vi "BeamPointing General hacking.vi"() -> ()   [LabVIEW 2013]
doc: "This example illustrates how to perform a continuous acquisition with a USB camera."
uses:
  <vilib>/vision/Image Controls.llb/IMAQ Image.ctl
  <vilib>/userdefined/High Color/IMAQdx.ctl
  shared programs/GUI_Template/GUI_master/tcp_new_data_event.ctl
  shared programs/GUI_Template/GUI_master/tcp new data cluster.ctl
  Add ROI Offset ImgData.vi
  Add Or Replace Coord Array.vi
  Add Or Replace Img Array.vi
  Add ROI Offset RectFilter.vi
  Add Or Replace String Array.vi
  <vilib>/regexp/Match Regular Expression.xnode
  <vilib>/vision/NI_Vision_Development_Module.lvlib
  <resource>/objmgr/IMAQImage.rc
  <vilib>/Analysis/NI_AALBase.lvlib
  <vilib>/Analysis/NI_AALPro.lvlib
panel:
  out "Main processing loop i":i32=3683
  out "image::1":T1(plugin-control) caption="Mode1"
  out "image::4":T1(plugin-control) caption="Mode1"
  out "image::5":T1(plugin-control) caption="Mode1"
  out "image::6":T1(plugin-control) caption="Mode1"
  out "image::7":T1(plugin-control) caption="Mode1"
  out "image::8":T1(plugin-control) caption="Mode1"
  out "GUIdevice 5":string="M1Cam"
  out "GUIdevice 4":string="M1Cam"
  out "GUIdevice 7":string="M1Cam"
  out "GUIdevice 6":string="M1Cam"
  out "GUIdevice 8":string="M1Cam"
  out "GUIdevice 9":string="M1Cam"
  out "image::9":T1(plugin-control) caption="Mode1"
  out "GUIdevice 3":string="M1Cam"
  out "GUIdevice 1":string="M1Cam"
  out "GUIdevice 2":string="M1Cam"
  out "image::2":T1(plugin-control) caption="Mode1"
  out "image::3":T1(plugin-control) caption="Mode1"
  out "error IO 2":errorcluster
  in  "insert tag":bool=TRUE
  out "tcp data event":T2
  out "configarraychanged":bool
  out "image names":string[](array[string])
  in  "recenter":bool
  out "Beam Detected":bool
  out "Move Y":bool
  out "Move X":bool
  in  "LoopMode":bool caption="Mode"
  in  "rescale":bool=TRUE
  in  "Step Size":u16=5
  in  "Feedback":bool
  out "MoveInProgress":bool caption="Move In Progress"
  in  "USB cameras":i32(listbox)=1 caption="Select Camera"
  in  "Manual Move":T3={"Down"=FALSE, "Up"=FALSE, "Right"=FALSE, "Left"=FALSE, "APulses X"=200, "APulses Y"=200, "StopButton"=FALSE}
  out "Status":string
  in  "Internal controls and indicators":T4(tab)
  out "grab loop i":i32=4
  out "Current ImageServer":cluster{"IPAddress":string, "Port":i32}={"IPAddress"="234.5.6.8", "Port"=58445}
  out "Ann. Images":T1[](array[typedef])=["imageserver0", "imageserver1", "imageserver2", "imageserver3", "imageserver4", "imageserver5"]
  in  "Tab Control 2":enum32{"Image saving", "stats", "TCP", "cams"}(tab)=enum."cams"
  in  "Boolean":bool
  in  "Base Directory":path
  out "SaveImgError":errorcluster
  in  "SavePict":bool
  out "error CamS":errorcluster
  out "Switch Time":u32=200
  out "one loop":u32=130
  out "# imgs in buffer":i32=5
  out "ImgBufferSize":i32=5
  out "AcqTime":u32=610845
  out "State":i32=12
  out "TCPconnecAnswer":bool=TRUE
  out "TCPconnecCmd":bool=TRUE
  out "error close connect":errorcluster
  in  "Remove Camera":bool
  in  "Mirror List Path":path=path "Z:/Software/control-common/Configuration files/DeviceList100TW.xml"
  out "XML Config File Path":path=path "Z:/Software/control-common/Configuration files/ConfigFile_192_168_10_184.xml"
  in  "Add Camera":bool
  out "# of cams":i32=6
  in  "Corr":bool[](array[boolean])=[FALSE, FALSE, FALSE, FALSE, FALSE, FALSE]
  out "Det":bool[](array[boolean])
  out "error out":errorcluster
  out "IMAQ status":bool
  out "Avg Img Buffer":u8[][][](array[numeric])
  out "Switch in":u32=299180745
  out "MirrorList":string[][](array[string])
  out "Corrective Move XY":T5(array[cluster])
  out "Cameras Names":string[](array[string])=["Null", "Null", "Null", "Null", "Null", "Null"]
  out "Deviation":cluster{"Dev. X":sgl, "Dev. Y":sgl}={"Dev. X"=0.0, "Dev. Y"=-5.0} {"Dev. X" format="%.1f"; "Dev. Y" format="%.1f"}
  out "Buffer2":T1
  out "DownloadedImg":T1
  out "CurrentName":string="*100TW M10"
  out "XML errors":bool
  out "Image Odd Out":T1
  out "DeviceNames":string[](array[string])=["no-device", "GasJet", "Godzilla_M1", "Godzilla_M2", "Godzilla_M3", "Godzilla_M4", "Godzilla_M6", "Godzilla_M8_Steer", "Chihuahua_M1", "Chihuahua_M2", "Collider_M4", "Collider_M5", "Collider_M8 Translation s3c4", "HeaterBlue-M1", "HeaterBlue-M2", "HeaterBlue-M3", "THz OAP Down", "G Spot Camera", "G Spot Monitor", "C Spot Monitor", "p15c4-Free", "THz_M5", "THz_M7A & Xtal", "THz_M7B", "THz MIrror Top", "THz OAP Top", "p2s2c2-Free", "p2s2c3-Free", "p2s2c4-Free", "Heater_M0", "Heater_M4", "Heater_M5", "Ignitor Iris", "Ignitor_M4", "Collider_M6", "Collder_M7", "C Spot Camera", "p2s5c1-FREE", "p2s5c2-FREE", "p2s5c3-FREE", "p2c5c4-FREE", "*100TW M9", "*100TW M10", "*100TW Preamp Up", "*100TW Input Preamp2", "*100TW Output Preamp2", "*100TW M0", "*100TW M2", "*100TW M4", "*100TW M6", "*100TW M8", "*100TW M13", "*100TW M20", "*100TW M22", "*100TW M23", "no pico", "no pico", "no pico", "mobile no ir", "regen out-salad#1", "preamp in-salad#2", "XPW 1", "blue periscope regen", "godzilla 1st", "godzilla IN", "Chihuahua IN", "Chihuahua 1st", "??XPW pico2", "Preamp 3rd pass", "Blue regen out"]
  out "size(s)":i32[](array[numeric])=[964, 1288]
  out "Iteration":u32
  in  "Onward":bool=TRUE
  out "Ellipse edges":cluster{"X":sgl, "Y":sgl}[](array[cluster])
  out "Buffer":T1
  out "Output Img":T1
  out "Reference Img":T1
  out "Background Img":T1
  out "counter":i32
  out "First step":bool
  out "IMAQ Session":refnum<k11>
  out "IMAQ Session Array":refnum<k11>[](array[refnum])
  out "Display Current":bool=TRUE
  out "Region of Interest":i32[](array[numeric])
  out "Acq Img":T1
  out "MoveInProgressTimeIN":u32=296721656
  out "IMAQdx Session":T6="cam2"
  out "start":u32=299180614
  out "Avg Deviation":cluster{sgl, sgl}={0.0, -5.0}
  out "InProgress":string[](array[string])
  out "Centroid Avg Buffer":cluster{"X Centroid":sgl, "Y Centroid":sgl}[](array[cluster])=[{"X Centroid"=343.0, "Y Centroid"=203.0}, {"X Centroid"=301.0, "Y Centroid"=181.0}, {"X Centroid"=334.0, "Y Centroid"=201.0}, {"X Centroid"=289.0, "Y Centroid"=154.0}, {"X Centroid"=319.0, "Y Centroid"=232.0}]
  out "Img Buffer":T1[](array[typedef])=["Buffer0", "Buffer1", "Buffer2", "Buffer3", "Buffer4"]
  out "OpenTime":u32=298569900
  out "RunON/OFF":bool
  out "last move time":u32=281970384
  out "DeviationArray":cluster{"X Centroid":sgl, "Y Centroid":sgl}[](array[cluster])
  out "ConnectArray":T7(array[cluster])=[{"IPaddress"="192.168.10.34", "Port"=63420, "connection ID"=refnum, "TCP error"={"status"=FALSE, "code"=0, "source"=""}}, {"IPaddress"="192.168.10.184", "Port"=63430, "connection ID"=refnum, "TCP error"={"status"=FALSE, "code"=0, "source"=""}}]
  out "Raw images":T1[](array[typedef])=["imageserver0", "imageserver1", "imageserver2", "imageserver3", "imageserver4", "imageserver5"]
  in  "XML Config File Path 2":path=path "H:/Software/control-common/Configuration files/ConfigFile_192_168_10_184.xml"
  out "AddCameraCluster":T8={"Add?"=FALSE, "Channel"=6, "Device Name"="no-device"}
  out "RemoveCameraCluster":cluster{"Remove?":bool, "number":i32}={"Remove?"=FALSE, "number"=-1}
  out "NewAvg":bool
  out "Thresh Img":T1
  out "Avg Img":T1
  out "really save cfg?":bool
  out "Buffer3":T1
  out "CamConfigArray":T9(array[cluster])=[{"ID"=64.0, "Name"="*100TW M8", "DeviceID"={"Slot Connector"=24, "IP Adress"="192.168.10.34", "Port"=63420, "Type"="picodriver"}, "CorrectConfig Cluster"={"Detection Parameters"={"Contrast"=0, "Treshold"=0, "Max Intensity"=0, "Max Intensity%"=0, "Rx"=0, "Ry"=0, "R%"=0.0}, "Reverse"={"Reverse X"=FALSE, "Reverse Y"=FALSE}, "Target"={"X Target"=0.0, "Y Target"=0.0}, "Region of Interest"=[0, 0, 0, 0], "Correction Parameters"={"X"=0.0, "Y"=0.0, "Movement Type"=0}, "Acquisition Parameters"={"Brightness"=0.0, "Contrast"=0.0, "Saturation"=0.0, "White level"=0.0}, "Background Path"=path "", "Reference Path"=path "", "XCalibration"=[], "YCalibration"=[]}, "Ontrak Channel"=0, "IMAQdx Session 2"="cam2", "ImageServer"={"IPAddress"="234.5.6.8", "Port"=58450}}, {"ID"=55.0, "Name"="*100TW M9", "DeviceID"={"Slot Connector"=31, "IP Adress"="192.168.10.34", "Port"=63420, "Type"="picodriver"}, "CorrectConfig Cluster"={"Detection Parameters"={"Contrast"=0, "Treshold"=0, "Max Intensity"=0, "Max Intensity%"=0, "Rx"=0, "Ry"=0, "R%"=0.0}, "Reverse"={"Reverse X"=FALSE, "Reverse Y"=FALSE}, "Target"={"X Target"=631.0, "Y Target"=473.0}, "Region of Interest"=[0, 0, 0, 0], "Correction Parameters"={"X"=0.0, "Y"=0.0, "Movement Type"=0}, "Acquisition Parameters"={"Brightness"=0.0, "Contrast"=0.0, "Saturation"=0.0, "White level"=0.0}, "Background Path"=path "", "Reference Path"=path "", "XCalibration"=[], "YCalibration"=[]}, "Ontrak Channel"=0, "IMAQdx Session 2"="cam2", "ImageServer"={"IPAddress"="234.5.6.8", "Port"=58444}}, {"ID"=56.0, "Name"="*100TW M10", "DeviceID"={"Slot Connector"=32, "IP Adress"="192.168.10.34", "Port"=63420, "Type"="picodriver"}, "CorrectConfig Cluster"={"Detection Parameters"={"Contrast"=53, "Treshold"=53, "Max Intensity"=255, "Max Intensity%"=80, "Rx"=116, "Ry"=92, "R%"=50.0}, "Reverse"={"Reverse X"=FALSE, "Reverse Y"=TRUE}, "Target"={"X Target"=334.0, "Y Target"=206.0}, "Region of Interest"=[0, 0, 0, 0], "Correction Parameters"={"X"=100.0, "Y"=100.0, "Movement Type"=0}, "Acquisition Parameters"={"Brightness"=0.0, "Contrast"=0.0, "Saturation"=0.0, "White level"=0.0}, "Background Path"=path "", "Reference Path"=path "", "XCalibration"=[], "YCalibration"=[]}, "Ontrak Channel"=0, "IMAQdx Session 2"="cam2", "ImageServer"={"IPAddress"="234.5.6.8", "Port"=58445}}, {"ID"=0.0, "Name"="*100TW M20", "DeviceID"={"Slot Connector"=1, "IP Adress"="192.168.10.184", "Port"=63430, "Type"="picodriver"}, "CorrectConfig Cluster"={"Detection Parameters"={"Contrast"=66, "Treshold"=66, "Max Intensity"=255, "Max Intensity%"=80, "Rx"=30, "Ry"=30, "R%"=50.0}, "Reverse"={"Reverse X"=TRUE, "Reverse Y"=TRUE}, "Target"={"X Target"=284.6373, "Y Target"=160.1435}, "Region of Interest"=[0, 0, 0, 0], "Correction Parameters"={"X"=20.0, "Y"=20.0, "Movement Type"=0}, "Acquisition Parameters"={"Brightness"=0.0, "Contrast"=0.0, "Saturation"=0.0, "White level"=0.0}, "Background Path"=path "", "Reference Path"=path "", "XCalibration"=[{-23000.0, -242.0}, {-22000.0, -229.0}, {-21000.0, -215.0}, {-20000.0, -203.0}, {-19000.0, -192.0}, {-18000.0, -182.0}, {-17000.0, -172.0}, {-16000.0, -162.0}, {-15000.0, -153.0}, {-14000.0, -141.0}, {-13000.0, -126.0}, {-12000.0, -105.0}, {-11000.0, -77.0}, {-10000.0, -44.0}, {0.0, 4.0}, {11000.0, 98.0}, {12000.0, 109.0}, {13000.0, 119.0}, {14000.0, 130.0}, {15000.0, 140.0}, {16000.0, 151.0}, {17000.0, 161.0}, {18000.0, 171.0}, {19000.0, 182.0}, {20000.0, 193.0}, {21000.0, 205.0}, {22000.0, 217.0}, {23000.0, 229.0}], "YCalibration"=[{-23000.0, 196.0}, {-22000.0, 189.0}, {-21000.0, 182.0}, {-20000.0, 174.0}, {-19000.0, 164.0}, {-18000.0, 153.0}, {-17000.0, 141.0}, {-16000.0, 133.0}, {-15000.0, 126.0}, {-14000.0, 117.0}, {-13000.0, 105.0}, {-12000.0, 90.0}, {-11000.0, 69.0}, {-10000.0, 42.0}, {0.0, -4.0}, {11000.0, -96.0}, {12000.0, -99.0}, {13000.0, -101.0}, {14000.0, -103.0}, {15000.0, -109.0}, {16000.0, -118.0}, {17000.0, -129.0}, {18000.0, -143.0}, {19000.0, -155.0}, {20000.0, -166.0}, {21000.0, -174.0}, {22000.0, -181.0}, {23000.0, -187.0}]}, "Ontrak Channel"=0, "IMAQdx Session 2"="cam2", "ImageServer"={"IPAddress"="234.5.6.8", "Port"=58443}}, {"ID"=12.0, "Name"="*100TW M22", "DeviceID"={"Slot Connector"=3, "IP Adress"="192.168.10.184", "Port"=63430, "Type"="picodriver"}, "CorrectConfig Cluster"={"Detection Parameters"={"Contrast"=59, "Treshold"=59, "Max Intensity"=255, "Max Intensity%"=80, "Rx"=47, "Ry"=33, "R%"=50.0}, "Reverse"={"Reverse X"=FALSE, "Reverse Y"=TRUE}, "Target"={"X Target"=319.0, "Y Target"=219.0}, "Region of Interest"=[0, 0, 0, 0], "Correction Parameters"={"X"=10000.0, "Y"=10000.0, "Movement Type"=0}, "Acquisition Parameters"={"Brightness"=0.0, "Contrast"=0.0, "Saturation"=0.0, "White level"=0.0}, "Background Path"=path "", "Reference Path"=path "", "XCalibration"=[], "YCalibration"=[]}, "Ontrak Channel"=0, "IMAQdx Session 2"="cam2", "ImageServer"={"IPAddress"="234.5.6.8", "Port"=58446}}, {"ID"=12.0, "Name"="*100TW M23", "DeviceID"={"Slot Connector"=4, "IP Adress"="192.168.10.184", "Port"=63430, "Type"="picodriver"}, "CorrectConfig Cluster"={"Detection Parameters"={"Contrast"=11, "Treshold"=11, "Max Intensity"=255, "Max Intensity%"=90, "Rx"=180, "Ry"=110, "R%"=50.0}, "Reverse"={"Reverse X"=FALSE, "Reverse Y"=TRUE}, "Target"={"X Target"=303.0, "Y Target"=342.0}, "Region of Interest"=[0, 0, 0, 0], "Correction Parameters"={"X"=0.0, "Y"=0.0, "Movement Type"=0}, "Acquisition Parameters"={"Brightness"=0.0, "Contrast"=0.0, "Saturation"=0.0, "White level"=0.0}, "Background Path"=path "", "Reference Path"=path "", "XCalibration"=[], "YCalibration"=[]}, "Ontrak Channel"=0, "IMAQdx Session 2"="cam2", "ImageServer"={"IPAddress"="234.5.6.8", "Port"=58442}}] {"CorrectConfig Cluster"."Acquisition Parameters"."White level" scale=0.3..1.26 scale format="%#_2f"; "CorrectConfig Cluster"."Acquisition Parameters"."Saturation" scale=0.5..1.5 scale format="%#_3f"; "CorrectConfig Cluster"."Acquisition Parameters"."Contrast" scale=0.4..1.5 scale format="%#_3f"; "CorrectConfig Cluster"."Acquisition Parameters"."Brightness" scale=-50.0..50.0 scale format="%#_2f"; "CorrectConfig Cluster"."Correction Parameters"."Movement Type" items=["Step", "Proportionnal"]; "CorrectConfig Cluster"."Target"."X Target" format="%#_5g"; "CorrectConfig Cluster"."Target"."Y Target" format="%#_5g"; "CorrectConfig Cluster"."Detection Parameters"."Max Intensity%" max=100 step=1}
  out "Ellipse":T10 {"Minor Axis"."Point 2"."Y" format="%.2f"; "Minor Axis"."Point 2"."X" format="%.2f"; "Minor Axis"."Point 1"."Y" format="%.2f"; "Minor Axis"."Point 1"."X" format="%.2f"; "Major Axis"."Point 2"."Y" format="%.2f"; "Major Axis"."Point 2"."X" format="%.2f"; "Major Axis"."Point 1"."Y" format="%.2f"; "Major Axis"."Point 1"."X" format="%.2f"; "Center"."Y" format="%.2f"; "Center"."X" format="%.2f"}
  out "Avg Variation":cluster{"mean X":dbl, "mean Y":dbl}={"mean X"=nan, "mean Y"=nan} {"mean X" format="%#_4g"; "mean Y" format="%#_4g"}
  in  "Acquisition Parameters dx":T11 {"Parameter4" min=0.0 max=0.1 scale=0.0..0.1 scale format="%#_2f"; "Parameter3" min=0.0 max=3.0 scale=0.0..3.0 scale format="%#_3f"; "Parameter2" min=1.0 max=10.0 scale=1.0..10.0 scale format="%#_3f"; "Parameter1" min=1 max=1048576 step=1 scale=1.0..1048576.0}
  in  "set scales":bool
  out "Image Ports":i32[](array[numeric])
  out "Image IPs":string[](array[string])
  out "device associated":string
  in  "Background Path":path
  in  "Reference Path":path
  out "BestRects Cluster":T12={"PreviousCenter"={"X"=0.0, "Y"=0.0}, "CurrentCenter"={"X"=334.0, "Y"=201.0}}
  out "Default devices":string[](array[string])=["*100TW M8", "*100TW M9", "*100TW M10", "*100TW M20", "*100TW M22", "*100TW M23"]
  out "Img Size":i32[](array[numeric])=[0, 0, 1288, 964]
  out "RectFilter":T13={"Left"=257, "Top"=144, "Right"=399, "Bottom"=260, "Rotation"=10.484647750854492} {"Rotation" format="%.2f"; "Left" scale=0.0..1024.0; "Right" scale=0.0..1024.0}
  out "History XY Buffer":T14(array[cluster])
  out "ImgDataArray":T15(array[cluster])
  out "DeviceList":T16(array[cluster])=[{"ID"=0.0, "Name"="no-device", "DeviceID"={"Slot Connector"=0, "IP Adress"="Ipaddress", "Port"=0, "Type"="Type"}, "Detection Parameters"={"Contrast"=0, "Treshold"=0, "Max Intensity"=0, "Max Intensity%"=0, "Rx"=0, "Ry"=0, "R%"=0.0}, "Reverse"={"Reverse X"=FALSE, "Reverse Y"=FALSE}, "Target"={"X Target"=0.0, "Y Target"=0.0}, "Region of Interest"=[0, 0, 0, 0], "Correction Parameters"={"X"=0.0, "Y"=0.0, "Movement Type"=0}, "Acquisition Parameters"={"Brightness"=0.0, "Contrast"=0.0, "Saturation"=0.0, "White level"=0.0}, "Background Path"=path "", "Reference Path"=path "", "XCalibration"=[], "YCalibration"=[], "ImageServer"={"IPAddress"="127.0.0.1", "Port"=3500}}, {"ID"=0.0, "Name"="GasJet", "DeviceID"={"Slot Connector"=44, "IP Adress"="192.168.10.183", "Port"=63400, "Type"="picodriver"}, "Detection Parameters"={"Contrast"=0, "Treshold"=0, "Max Intensity"=0, "Max Intensity%"=0, "Rx"=0, "Ry"=0, "R%"=0.0}, "Reverse"={"Reverse X"=FALSE, "Reverse Y"=FALSE}, "Target"={"X Target"=0.0, "Y Target"=0.0}, "Region of Interest"=[0, 0, 0, 0], "Correction Parameters"={"X"=0.0, "Y"=0.0, "Movement Type"=0}, "Acquisition Parameters"={"Brightness"=0.0, "Contrast"=0.0, "Saturation"=0.0, "White level"=0.0}, "Background Path"=path "", "Reference Path"=path "", "XCalibration"=[], "YCalibration"=[], "ImageServer"={"IPAddress"="127.0.0.1", "Port"=3500}}, {"ID"=14.0, "Name"="Godzilla_M1", "DeviceID"={"Slot Connector"=11, "IP Adress"="192.168.10.183", "Port"=63400, "Type"="picodriver"}, "Detection Parameters"={"Contrast"=0, "Treshold"=0, "Max Intensity"=0, "Max Intensity%"=0, "Rx"=0, "Ry"=0, "R%"=0.0}, "Reverse"={"Reverse X"=FALSE, "Reverse Y"=FALSE}, "Target"={"X Target"=0.0, "Y Target"=0.0}, "Region of Interest"=[0, 0, 0, 0], "Correction Parameters"={"X"=0.0, "Y"=0.0, "Movement Type"=0}, "Acquisition Parameters"={"Brightness"=0.0, "Contrast"=0.0, "Saturation"=0.0, "White level"=0.0}, "Background Path"=path "", "Reference Path"=path "", "XCalibration"=[], "YCalibration"=[], "ImageServer"={"IPAddress"="127.0.0.1", "Port"=3500}}, {"ID"=15.0, "Name"="Godzilla_M2", "DeviceID"={"Slot Connector"=12, "IP Adress"="192.168.10.183", "Port"=63400, "Type"="picodriver"}, "Detection Parameters"={"Contrast"=0, "Treshold"=0, "Max Intensity"=0, "Max Intensity%"=0, "Rx"=0, "Ry"=0, "R%"=0.0}, "Reverse"={"Reverse X"=FALSE, "Reverse Y"=FALSE}, "Target"={"X Target"=0.0, "Y Target"=0.0}, "Region of Interest"=[0, 0, 0, 0], "Correction Parameters"={"X"=0.0, "Y"=0.0, "Movement Type"=0}, "Acquisition Parameters"={"Brightness"=0.0, "Contrast"=0.0, "Saturation"=0.0, "White level"=0.0}, "Background Path"=path "", "Reference Path"=path "", "XCalibration"=[], "YCalibration"=[], "ImageServer"={"IPAddress"="127.0.0.1", "Port"=3500}}, {"ID"=16.0, "Name"="Godzilla_M3", "DeviceID"={"Slot Connector"=13, "IP Adress"="192.168.10.183", "Port"=63400, "Type"="picodriver"}, "Detection Parameters"={"Contrast"=0, "Treshold"=0, "Max Intensity"=0, "Max Intensity%"=0, "Rx"=0, "Ry"=0, "R%"=0.0}, "Reverse"={"Reverse X"=FALSE, "Reverse Y"=FALSE}, "Target"={"X Target"=0.0, "Y Target"=0.0}, "Region of Interest"=[0, 0, 0, 0], "Correction Parameters"={"X"=0.0, "Y"=0.0, "Movement Type"=0}, "Acquisition Parameters"={"Brightness"=0.0, "Contrast"=0.0, "Saturation"=0.0, "White level"=0.0}, "Background Path"=path "", "Reference Path"=path "", "XCalibration"=[], "YCalibration"=[], "ImageServer"={"IPAddress"="127.0.0.1", "Port"=3500}}, {"ID"=17.0, "Name"="Godzilla_M4", "DeviceID"={"Slot Connector"=14, "IP Adress"="192.168.10.183", "Port"=63400, "Type"="picodriver"}, "Detection Parameters"={"Contrast"=0, "Treshold"=0, "Max Intensity"=0, "Max Intensity%"=0, "Rx"=0, "Ry"=0, "R%"=0.0}, "Reverse"={"Reverse X"=FALSE, "Reverse Y"=FALSE}, "Target"={"X Target"=0.0, "Y Target"=0.0}, "Region of Interest"=[0, 0, 0, 0], "Correction Parameters"={"X"=0.0, "Y"=0.0, "Movement Type"=0}, "Acquisition Parameters"={"Brightness"=0.0, "Contrast"=0.0, "Saturation"=0.0, "White level"=0.0}, "Background Path"=path "", "Reference Path"=path "", "XCalibration"=[], "YCalibration"=[], "ImageServer"={"IPAddress"="127.0.0.1", "Port"=3500}}, {"ID"=18.0, "Name"="Godzilla_M6", "DeviceID"={"Slot Connector"=21, "IP Adress"="192.168.10.183", "Port"=63400, "Type"="picodriver"}, "Detection Parameters"={"Contrast"=0, "Treshold"=0, "Max Intensity"=0, "Max Intensity%"=0, "Rx"=0, "Ry"=0, "R%"=0.0}, "Reverse"={"Reverse X"=FALSE, "Reverse Y"=FALSE}, "Target"={"X Target"=0.0, "Y Target"=0.0}, "Region of Interest"=[0, 0, 0, 0], "Correction Parameters"={"X"=0.0, "Y"=0.0, "Movement Type"=0}, "Acquisition Parameters"={"Brightness"=0.0, "Contrast"=0.0, "Saturation"=0.0, "White level"=0.0}, "Background Path"=path "", "Reference Path"=path "", "XCalibration"=[], "YCalibration"=[], "ImageServer"={"IPAddress"="127.0.0.1", "Port"=3500}}, {"ID"=19.0, "Name"="Godzilla_M8_Steer", "DeviceID"={"Slot Connector"=22, "IP Adress"="192.168.10.183", "Port"=63400, "Type"="picodriver"}, "Detection Parameters"={"Contrast"=0, "Treshold"=0, "Max Intensity"=0, "Max Intensity%"=0, "Rx"=0, "Ry"=0, "R%"=0.0}, "Reverse"={"Reverse X"=FALSE, "Reverse Y"=FALSE}, "Target"={"X Target"=0.0, "Y Target"=0.0}, "Region of Interest"=[0, 0, 0, 0], "Correction Parameters"={"X"=0.0, "Y"=0.0, "Movement Type"=0}, "Acquisition Parameters"={"Brightness"=0.0, "Contrast"=0.0, "Saturation"=0.0, "White level"=0.0}, "Background Path"=path "", "Reference Path"=path "", "XCalibration"=[], "YCalibration"=[], "ImageServer"={"IPAddress"="127.0.0.1", "Port"=3500}}, {"ID"=20.0, "Name"="Chihuahua_M1", "DeviceID"={"Slot Connector"=23, "IP Adress"="192.168.10.183", "Port"=63400, "Type"="picodriver"}, "Detection Parameters"={"Contrast"=0, "Treshold"=0, "Max Intensity"=0, "Max Intensity%"=0, "Rx"=0, "Ry"=0, "R%"=0.0}, "Reverse"={"Reverse X"=FALSE, "Reverse Y"=FALSE}, "Target"={"X Target"=0.0, "Y Target"=0.0}, "Region of Interest"=[0, 0, 0, 0], "Correction Parameters"={"X"=0.0, "Y"=0.0, "Movement Type"=0}, "Acquisition Parameters"={"Brightness"=0.0, "Contrast"=0.0, "Saturation"=0.0, "White level"=0.0}, "Background Path"=path "", "Reference Path"=path "", "XCalibration"=[], "YCalibration"=[], "ImageServer"={"IPAddress"="127.0.0.1", "Port"=3500}}, {"ID"=21.0, "Name"="Chihuahua_M2", "DeviceID"={"Slot Connector"=24, "IP Adress"="192.168.10.183", "Port"=63400, "Type"="picodriver"}, "Detection Parameters"={"Contrast"=0, "Treshold"=0, "Max Intensity"=0, "Max Intensity%"=0, "Rx"=0, "Ry"=0, "R%"=0.0}, "Reverse"={"Reverse X"=FALSE, "Reverse Y"=FALSE}, "Target"={"X Target"=0.0, "Y Target"=0.0}, "Region of Interest"=[0, 0, 0, 0], "Correction Parameters"={"X"=0.0, "Y"=0.0, "Movement Type"=0}, "Acquisition Parameters"={"Brightness"=0.0, "Contrast"=0.0, "Saturation"=0.0, "White level"=0.0}, "Background Path"=path "", "Reference Path"=path "", "XCalibration"=[], "YCalibration"=[], "ImageServer"={"IPAddress"="127.0.0.1", "Port"=3500}}, {"ID"=22.0, "Name"="Collider_M4", "DeviceID"={"Slot Connector"=31, "IP Adress"="192.168.10.183", "Port"=63400, "Type"="picodriver"}, "Detection Parameters"={"Contrast"=0, "Treshold"=0, "Max Intensity"=0, "Max Intensity%"=0, "Rx"=0, "Ry"=0, "R%"=0.0}, "Reverse"={"Reverse X"=FALSE, "Reverse Y"=FALSE}, "Target"={"X Target"=0.0, "Y Target"=0.0}, "Region of Interest"=[0, 0, 0, 0], "Correction Parameters"={"X"=0.0, "Y"=0.0, "Movement Type"=0}, "Acquisition Parameters"={"Brightness"=0.0, "Contrast"=0.0, "Saturation"=0.0, "White level"=0.0}, "Background Path"=path "", "Reference Path"=path "", "XCalibration"=[], "YCalibration"=[], "ImageServer"={"IPAddress"="127.0.0.1", "Port"=3500}}, {"ID"=23.0, "Name"="Collider_M5", "DeviceID"={"Slot Connector"=32, "IP Adress"="192.168.10.183", "Port"=63400, "Type"="picodriver"}, "Detection Parameters"={"Contrast"=0, "Treshold"=0, "Max Intensity"=0, "Max Intensity%"=0, "Rx"=0, "Ry"=0, "R%"=0.0}, "Reverse"={"Reverse X"=FALSE, "Reverse Y"=FALSE}, "Target"={"X Target"=0.0, "Y Target"=0.0}, "Region of Interest"=[0, 0, 0, 0], "Correction Parameters"={"X"=0.0, "Y"=0.0, "Movement Type"=0}, "Acquisition Parameters"={"Brightness"=0.0, "Contrast"=0.0, "Saturation"=0.0, "White level"=0.0}, "Background Path"=path "", "Reference Path"=path "", "XCalibration"=[], "YCalibration"=[], "ImageServer"={"IPAddress"="127.0.0.1", "Port"=3500}}, {"ID"=24.0, "Name"="Collider_M8 Translation s3c4", "DeviceID"={"Slot Connector"=33, "IP Adress"="192.168.10.183", "Port"=63400, "Type"="picodriver"}, "Detection Parameters"={"Contrast"=0, "Treshold"=0, "Max Intensity"=0, "Max Intensity%"=0, "Rx"=0, "Ry"=0, "R%"=0.0}, "Reverse"={"Reverse X"=FALSE, "Reverse Y"=FALSE}, "Target"={"X Target"=0.0, "Y Target"=0.0}, "Region of Interest"=[0, 0, 0, 0], "Correction Parameters"={"X"=0.0, "Y"=0.0, "Movement Type"=0}, "Acquisition Parameters"={"Brightness"=0.0, "Contrast"=0.0, "Saturation"=0.0, "White level"=0.0}, "Background Path"=path "", "Reference Path"=path "", "XCalibration"=[], "YCalibration"=[], "ImageServer"={"IPAddress"="127.0.0.1", "Port"=3500}}, {"ID"=26.0, "Name"="HeaterBlue-M1", "DeviceID"={"Slot Connector"=34, "IP Adress"="192.168.10.183", "Port"=63400, "Type"="picodriver"}, "Detection Parameters"={"Contrast"=0, "Treshold"=0, "Max Intensity"=0, "Max Intensity%"=0, "Rx"=0, "Ry"=0, "R%"=0.0}, "Reverse"={"Reverse X"=FALSE, "Reverse Y"=FALSE}, "Target"={"X Target"=0.0, "Y Target"=0.0}, "Region of Interest"=[0, 0, 0, 0], "Correction Parameters"={"X"=0.0, "Y"=0.0, "Movement Type"=0}, "Acquisition Parameters"={"Brightness"=0.0, "Contrast"=0.0, "Saturation"=0.0, "White level"=0.0}, "Background Path"=path "", "Reference Path"=path "", "XCalibration"=[], "YCalibration"=[], "ImageServer"={"IPAddress"="127.0.0.1", "Port"=3500}}, {"ID"=27.0, "Name"="HeaterBlue-M2", "DeviceID"={"Slot Connector"=41, "IP Adress"="192.168.10.183", "Port"=63400, "Type"="picodriver"}, "Detection Parameters"={"Contrast"=0, "Treshold"=0, "Max Intensity"=0, "Max Intensity%"=0, "Rx"=0, "Ry"=0, "R%"=0.0}, "Reverse"={"Reverse X"=FALSE, "Reverse Y"=FALSE}, "Target"={"X Target"=0.0, "Y Target"=0.0}, "Region of Interest"=[0, 0, 0, 0], "Correction Parameters"={"X"=0.0, "Y"=0.0, "Movement Type"=0}, "Acquisition Parameters"={"Brightness"=0.0, "Contrast"=0.0, "Saturation"=0.0, "White level"=0.0}, "Background Path"=path "", "Reference Path"=path "", "XCalibration"=[], "YCalibration"=[], "ImageServer"={"IPAddress"="127.0.0.1", "Port"=3500}}, {"ID"=28.0, "Name"="HeaterBlue-M3", "DeviceID"={"Slot Connector"=42, "IP Adress"="192.168.10.183", "Port"=63400, "Type"="picodriver"}, "Detection Parameters"={"Contrast"=0, "Treshold"=0, "Max Intensity"=0, "Max Intensity%"=0, "Rx"=0, "Ry"=0, "R%"=0.0}, "Reverse"={"Reverse X"=FALSE, "Reverse Y"=FALSE}, "Target"={"X Target"=0.0, "Y Target"=0.0}, "Region of Interest"=[0, 0, 0, 0], "Correction Parameters"={"X"=0.0, "Y"=0.0, "Movement Type"=0}, "Acquisition Parameters"={"Brightness"=0.0, "Contrast"=0.0, "Saturation"=0.0, "White level"=0.0}, "Background Path"=path "", "Reference Path"=path "", "XCalibration"=[], "YCalibration"=[], "ImageServer"={"IPAddress"="127.0.0.1", "Port"=3500}}, {"ID"=29.0, "Name"="THz OAP Down", "DeviceID"={"Slot Connector"=43, "IP Adress"="192.168.10.183", "Port"=63400, "Type"="picodriver"}, "Detection Parameters"={"Contrast"=0, "Treshold"=0, "Max Intensity"=0, "Max Intensity%"=0, "Rx"=0, "Ry"=0, "R%"=0.0}, "Reverse"={"Reverse X"=FALSE, "Reverse Y"=FALSE}, "Target"={"X Target"=0.0, "Y Target"=0.0}, "Region of Interest"=[0, 0, 0, 0], "Correction Parameters"={"X"=0.0, "Y"=0.0, "Movement Type"=0}, "Acquisition Parameters"={"Brightness"=0.0, "Contrast"=0.0, "Saturation"=0.0, "White level"=0.0}, "Background Path"=path "", "Reference Path"=path "", "XCalibration"=[], "YCalibration"=[], "ImageServer"={"IPAddress"="127.0.0.1", "Port"=3500}}, {"ID"=30.0, "Name"="G Spot Camera", "DeviceID"={"Slot Connector"=51, "IP Adress"="192.168.10.183", "Port"=63400, "Type"="picodriver"}, "Detection Parameters"={"Contrast"=0, "Treshold"=0, "Max Intensity"=0, "Max Intensity%"=0, "Rx"=0, "Ry"=0, "R%"=0.0}, "Reverse"={"Reverse X"=FALSE, "Reverse Y"=FALSE}, "Target"={"X Target"=0.0, "Y Target"=0.0}, "Region of Interest"=[0, 0, 0, 0], "Correction Parameters"={"X"=0.0, "Y"=0.0, "Movement Type"=0}, "Acquisition Parameters"={"Brightness"=0.0, "Contrast"=0.0, "Saturation"=0.0, "White level"=0.0}, "Background Path"=path "", "Reference Path"=path "", "XCalibration"=[], "YCalibration"=[], "ImageServer"={"IPAddress"="127.0.0.1", "Port"=3500}}, {"ID"=31.0, "Name"="G Spot Monitor", "DeviceID"={"Slot Connector"=52, "IP Adress"="192.168.10.183", "Port"=63400, "Type"="picodriver"}, "Detection Parameters"={"Contrast"=0, "Treshold"=0, "Max Intensity"=0, "Max Intensity%"=0, "Rx"=0, "Ry"=0, "R%"=0.0}, "Reverse"={"Reverse X"=FALSE, "Reverse Y"=FALSE}, "Target"={"X Target"=0.0, "Y Target"=0.0}, "Region of Interest"=[0, 0, 0, 0], "Correction Parameters"={"X"=0.0, "Y"=0.0, "Movement Type"=0}, "Acquisition Parameters"={"Brightness"=0.0, "Contrast"=0.0, "Saturation"=0.0, "White level"=0.0}, "Background Path"=path "", "Reference Path"=path "", "XCalibration"=[], "YCalibration"=[], "ImageServer"={"IPAddress"="127.0.0.1", "Port"=3500}}, {"ID"=32.0, "Name"="C Spot Monitor", "DeviceID"={"Slot Connector"=53, "IP Adress"="192.168.10.183", "Port"=63400, "Type"="picodriver"}, "Detection Parameters"={"Contrast"=0, "Treshold"=0, "Max Intensity"=0, "Max Intensity%"=0, "Rx"=0, "Ry"=0, "R%"=0.0}, "Reverse"={"Reverse X"=FALSE, "Reverse Y"=FALSE}, "Target"={"X Target"=0.0, "Y Target"=0.0}, "Region of Interest"=[0, 0, 0, 0], "Correction Parameters"={"X"=0.0, "Y"=0.0, "Movement Type"=0}, "Acquisition Parameters"={"Brightness"=0.0, "Contrast"=0.0, "Saturation"=0.0, "White level"=0.0}, "Background Path"=path "", "Reference Path"=path "", "XCalibration"=[], "YCalibration"=[], "ImageServer"={"IPAddress"="127.0.0.1", "Port"=3500}}, {"ID"=33.0, "Name"="p15c4-Free", "DeviceID"={"Slot Connector"=54, "IP Adress"="192.168.10.183", "Port"=63400, "Type"="picodriver"}, "Detection Parameters"={"Contrast"=0, "Treshold"=0, "Max Intensity"=0, "Max Intensity%"=0, "Rx"=0, "Ry"=0, "R%"=0.0}, "Reverse"={"Reverse X"=FALSE, "Reverse Y"=FALSE}, "Target"={"X Target"=0.0, "Y Target"=0.0}, "Region of Interest"=[0, 0, 0, 0], "Correction Parameters"={"X"=0.0, "Y"=0.0, "Movement Type"=0}, "Acquisition Parameters"={"Brightness"=0.0, "Contrast"=0.0, "Saturation"=0.0, "White level"=0.0}, "Background Path"=path "", "Reference Path"=path "", "XCalibration"=[], "YCalibration"=[], "ImageServer"={"IPAddress"="127.0.0.1", "Port"=3500}}, {"ID"=34.0, "Name"="THz_M5", "DeviceID"={"Slot Connector"=11, "IP Adress"="192.168.10.183", "Port"=63410, "Type"="picodriver"}, "Detection Parameters"={"Contrast"=0, "Treshold"=0, "Max Intensity"=0, "Max Intensity%"=0, "Rx"=0, "Ry"=0, "R%"=0.0}, "Reverse"={"Reverse X"=FALSE, "Reverse Y"=FALSE}, "Target"={"X Target"=0.0, "Y Target"=0.0}, "Region of Interest"=[0, 0, 0, 0], "Correction Parameters"={"X"=0.0, "Y"=0.0, "Movement Type"=0}, "Acquisition Parameters"={"Brightness"=0.0, "Contrast"=0.0, "Saturation"=0.0, "White level"=0.0}, "Background Path"=path "", "Reference Path"=path "", "XCalibration"=[], "YCalibration"=[], "ImageServer"={"IPAddress"="127.0.0.1", "Port"=3500}}, {"ID"=35.0, "Name"="THz_M7A & Xtal", "DeviceID"={"Slot Connector"=12, "IP Adress"="192.168.10.183", "Port"=63410, "Type"="picodriver"}, "Detection Parameters"={"Contrast"=0, "Treshold"=0, "Max Intensity"=0, "Max Intensity%"=0, "Rx"=0, "Ry"=0, "R%"=0.0}, "Reverse"={"Reverse X"=FALSE, "Reverse Y"=FALSE}, "Target"={"X Target"=0.0, "Y Target"=0.0}, "Region of Interest"=[0, 0, 0, 0], "Correction Parameters"={"X"=0.0, "Y"=0.0, "Movement Type"=0}, "Acquisition Parameters"={"Brightness"=0.0, "Contrast"=0.0, "Saturation"=0.0, "White level"=0.0}, "Background Path"=path "", "Reference Path"=path "", "XCalibration"=[], "YCalibration"=[], "ImageServer"={"IPAddress"="127.0.0.1", "Port"=3500}}, {"ID"=36.0, "Name"="THz_M7B", "DeviceID"={"Slot Connector"=13, "IP Adress"="192.168.10.183", "Port"=63410, "Type"="picodriver"}, "Detection Parameters"={"Contrast"=0, "Treshold"=0, "Max Intensity"=0, "Max Intensity%"=0, "Rx"=0, "Ry"=0, "R%"=0.0}, "Reverse"={"Reverse X"=FALSE, "Reverse Y"=FALSE}, "Target"={"X Target"=0.0, "Y Target"=0.0}, "Region of Interest"=[0, 0, 0, 0], "Correction Parameters"={"X"=0.0, "Y"=0.0, "Movement Type"=0}, "Acquisition Parameters"={"Brightness"=0.0, "Contrast"=0.0, "Saturation"=0.0, "White level"=0.0}, "Background Path"=path "", "Reference Path"=path "", "XCalibration"=[], "YCalibration"=[], "ImageServer"={"IPAddress"="127.0.0.1", "Port"=3500}}, {"ID"=37.0, "Name"="THz MIrror Top", "DeviceID"={"Slot Connector"=14, "IP Adress"="192.168.10.183", "Port"=63410, "Type"="picodriver"}, "Detection Parameters"={"Contrast"=0, "Treshold"=0, "Max Intensity"=0, "Max Intensity%"=0, "Rx"=0, "Ry"=0, "R%"=0.0}, "Reverse"={"Reverse X"=FALSE, "Reverse Y"=FALSE}, "Target"={"X Target"=0.0, "Y Target"=0.0}, "Region of Interest"=[0, 0, 0, 0], "Correction Parameters"={"X"=0.0, "Y"=0.0, "Movement Type"=0}, "Acquisition Parameters"={"Brightness"=0.0, "Contrast"=0.0, "Saturation"=0.0, "White level"=0.0}, "Background Path"=path "", "Reference Path"=path "", "XCalibration"=[], "YCalibration"=[], "ImageServer"={"IPAddress"="127.0.0.1", "Port"=3500}}, {"ID"=38.0, "Name"="THz OAP Top", "DeviceID"={"Slot Connector"=21, "IP Adress"="192.168.10.183", "Port"=63410, "Type"="picodriver"}, "Detection Parameters"={"Contrast"=0, "Treshold"=0, "Max Intensity"=0, "Max Intensity%"=0, "Rx"=0, "Ry"=0, "R%"=0.0}, "Reverse"={"Reverse X"=FALSE, "Reverse Y"=FALSE}, "Target"={"X Target"=0.0, "Y Target"=0.0}, "Region of Interest"=[0, 0, 0, 0], "Correction Parameters"={"X"=0.0, "Y"=0.0, "Movement Type"=0}, "Acquisition Parameters"={"Brightness"=0.0, "Contrast"=0.0, "Saturation"=0.0, "White level"=0.0}, "Background Path"=path "", "Reference Path"=path "", "XCalibration"=[], "YCalibration"=[], "ImageServer"={"IPAddress"="127.0.0.1", "Port"=3500}}, {"ID"=39.0, "Name"="p2s2c2-Free", "DeviceID"={"Slot Connector"=22, "IP Adress"="192.168.10.183", "Port"=63410, "Type"="picodriver"}, "Detection Parameters"={"Contrast"=0, "Treshold"=0, "Max Intensity"=0, "Max Intensity%"=0, "Rx"=0, "Ry"=0, "R%"=0.0}, "Reverse"={"Reverse X"=FALSE, "Reverse Y"=FALSE}, "Target"={"X Target"=0.0, "Y Target"=0.0}, "Region of Interest"=[0, 0, 0, 0], "Correction Parameters"={"X"=0.0, "Y"=0.0, "Movement Type"=0}, "Acquisition Parameters"={"Brightness"=0.0, "Contrast"=0.0, "Saturation"=0.0, "White level"=0.0}, "Background Path"=path "", "Reference Path"=path "", "XCalibration"=[], "YCalibration"=[], "ImageServer"={"IPAddress"="127.0.0.1", "Port"=3500}}, {"ID"=40.0, "Name"="p2s2c3-Free", "DeviceID"={"Slot Connector"=23, "IP Adress"="192.168.10.183", "Port"=63410, "Type"="picodriver"}, "Detection Parameters"={"Contrast"=0, "Treshold"=0, "Max Intensity"=0, "Max Intensity%"=0, "Rx"=0, "Ry"=0, "R%"=0.0}, "Reverse"={"Reverse X"=FALSE, "Reverse Y"=FALSE}, "Target"={"X Target"=0.0, "Y Target"=0.0}, "Region of Interest"=[0, 0, 0, 0], "Correction Parameters"={"X"=0.0, "Y"=0.0, "Movement Type"=0}, "Acquisition Parameters"={"Brightness"=0.0, "Contrast"=0.0, "Saturation"=0.0, "White level"=0.0}, "Background Path"=path "", "Reference Path"=path "", "XCalibration"=[], "YCalibration"=[], "ImageServer"={"IPAddress"="127.0.0.1", "Port"=3500}}, {"ID"=41.0, "Name"="p2s2c4-Free", "DeviceID"={"Slot Connector"=24, "IP Adress"="192.168.10.183", "Port"=63410, "Type"="picodriver"}, "Detection Parameters"={"Contrast"=0, "Treshold"=0, "Max Intensity"=0, "Max Intensity%"=0, "Rx"=0, "Ry"=0, "R%"=0.0}, "Reverse"={"Reverse X"=FALSE, "Reverse Y"=FALSE}, "Target"={"X Target"=0.0, "Y Target"=0.0}, "Region of Interest"=[0, 0, 0, 0], "Correction Parameters"={"X"=0.0, "Y"=0.0, "Movement Type"=0}, "Acquisition Parameters"={"Brightness"=0.0, "Contrast"=0.0, "Saturation"=0.0, "White level"=0.0}, "Background Path"=path "", "Reference Path"=path "", "XCalibration"=[], "YCalibration"=[], "ImageServer"={"IPAddress"="127.0.0.1", "Port"=3500}}, {"ID"=42.0, "Name"="Heater_M0", "DeviceID"={"Slot Connector"=31, "IP Adress"="192.168.10.183", "Port"=63410, "Type"="picodriver"}, "Detection Parameters"={"Contrast"=0, "Treshold"=0, "Max Intensity"=0, "Max Intensity%"=0, "Rx"=0, "Ry"=0, "R%"=0.0}, "Reverse"={"Reverse X"=FALSE, "Reverse Y"=FALSE}, "Target"={"X Target"=0.0, "Y Target"=0.0}, "Region of Interest"=[0, 0, 0, 0], "Correction Parameters"={"X"=0.0, "Y"=0.0, "Movement Type"=0}, "Acquisition Parameters"={"Brightness"=0.0, "Contrast"=0.0, "Saturation"=0.0, "White level"=0.0}, "Background Path"=path "", "Reference Path"=path "", "XCalibration"=[], "YCalibration"=[], "ImageServer"={"IPAddress"="127.0.0.1", "Port"=3500}}, {"ID"=43.0, "Name"="Heater_M4", "DeviceID"={"Slot Connector"=32, "IP Adress"="192.168.10.183", "Port"=63410, "Type"="picodriver"}, "Detection Parameters"={"Contrast"=0, "Treshold"=0, "Max Intensity"=0, "Max Intensity%"=0, "Rx"=0, "Ry"=0, "R%"=0.0}, "Reverse"={"Reverse X"=FALSE, "Reverse Y"=FALSE}, "Target"={"X Target"=0.0, "Y Target"=0.0}, "Region of Interest"=[0, 0, 0, 0], "Correction Parameters"={"X"=0.0, "Y"=0.0, "Movement Type"=0}, "Acquisition Parameters"={"Brightness"=0.0, "Contrast"=0.0, "Saturation"=0.0, "White level"=0.0}, "Background Path"=path "", "Reference Path"=path "", "XCalibration"=[], "YCalibration"=[], "ImageServer"={"IPAddress"="127.0.0.1", "Port"=3500}}, {"ID"=44.0, "Name"="Heater_M5", "DeviceID"={"Slot Connector"=33, "IP Adress"="192.168.10.183", "Port"=63410, "Type"="picodriver"}, "Detection Parameters"={"Contrast"=0, "Treshold"=0, "Max Intensity"=0, "Max Intensity%"=0, "Rx"=0, "Ry"=0, "R%"=0.0}, "Reverse"={"Reverse X"=FALSE, "Reverse Y"=FALSE}, "Target"={"X Target"=0.0, "Y Target"=0.0}, "Region of Interest"=[0, 0, 0, 0], "Correction Parameters"={"X"=0.0, "Y"=0.0, "Movement Type"=0}, "Acquisition Parameters"={"Brightness"=0.0, "Contrast"=0.0, "Saturation"=0.0, "White level"=0.0}, "Background Path"=path "", "Reference Path"=path "", "XCalibration"=[], "YCalibration"=[], "ImageServer"={"IPAddress"="127.0.0.1", "Port"=3500}}, {"ID"=45.0, "Name"="Ignitor Iris", "DeviceID"={"Slot Connector"=34, "IP Adress"="192.168.10.183", "Port"=63410, "Type"="picodriver"}, "Detection Parameters"={"Contrast"=0, "Treshold"=0, "Max Intensity"=0, "Max Intensity%"=0, "Rx"=0, "Ry"=0, "R%"=0.0}, "Reverse"={"Reverse X"=FALSE, "Reverse Y"=FALSE}, "Target"={"X Target"=0.0, "Y Target"=0.0}, "Region of Interest"=[0, 0, 0, 0], "Correction Parameters"={"X"=0.0, "Y"=0.0, "Movement Type"=0}, "Acquisition Parameters"={"Brightness"=0.0, "Contrast"=0.0, "Saturation"=0.0, "White level"=0.0}, "Background Path"=path "", "Reference Path"=path "", "XCalibration"=[], "YCalibration"=[], "ImageServer"={"IPAddress"="127.0.0.1", "Port"=3500}}, {"ID"=46.0, "Name"="Ignitor_M4", "DeviceID"={"Slot Connector"=41, "IP Adress"="192.168.10.183", "Port"=63410, "Type"="picodriver"}, "Detection Parameters"={"Contrast"=0, "Treshold"=0, "Max Intensity"=0, "Max Intensity%"=0, "Rx"=0, "Ry"=0, "R%"=0.0}, "Reverse"={"Reverse X"=FALSE, "Reverse Y"=FALSE}, "Target"={"X Target"=0.0, "Y Target"=0.0}, "Region of Interest"=[0, 0, 0, 0], "Correction Parameters"={"X"=0.0, "Y"=0.0, "Movement Type"=0}, "Acquisition Parameters"={"Brightness"=0.0, "Contrast"=0.0, "Saturation"=0.0, "White level"=0.0}, "Background Path"=path "", "Reference Path"=path "", "XCalibration"=[], "YCalibration"=[], "ImageServer"={"IPAddress"="127.0.0.1", "Port"=3500}}, {"ID"=47.0, "Name"="Collider_M6", "DeviceID"={"Slot Connector"=42, "IP Adress"="192.168.10.183", "Port"=63410, "Type"="picodriver"}, "Detection Parameters"={"Contrast"=0, "Treshold"=0, "Max Intensity"=0, "Max Intensity%"=0, "Rx"=0, "Ry"=0, "R%"=0.0}, "Reverse"={"Reverse X"=FALSE, "Reverse Y"=FALSE}, "Target"={"X Target"=0.0, "Y Target"=0.0}, "Region of Interest"=[0, 0, 0, 0], "Correction Parameters"={"X"=0.0, "Y"=0.0, "Movement Type"=0}, "Acquisition Parameters"={"Brightness"=0.0, "Contrast"=0.0, "Saturation"=0.0, "White level"=0.0}, "Background Path"=path "", "Reference Path"=path "", "XCalibration"=[], "YCalibration"=[], "ImageServer"={"IPAddress"="127.0.0.1", "Port"=3500}}, {"ID"=48.0, "Name"="Collder_M7", "DeviceID"={"Slot Connector"=43, "IP Adress"="192.168.10.183", "Port"=63410, "Type"="picodriver"}, "Detection Parameters"={"Contrast"=0, "Treshold"=0, "Max Intensity"=0, "Max Intensity%"=0, "Rx"=0, "Ry"=0, "R%"=0.0}, "Reverse"={"Reverse X"=FALSE, "Reverse Y"=FALSE}, "Target"={"X Target"=0.0, "Y Target"=0.0}, "Region of Interest"=[0, 0, 0, 0], "Correction Parameters"={"X"=0.0, "Y"=0.0, "Movement Type"=0}, "Acquisition Parameters"={"Brightness"=0.0, "Contrast"=0.0, "Saturation"=0.0, "White level"=0.0}, "Background Path"=path "", "Reference Path"=path "", "XCalibration"=[], "YCalibration"=[], "ImageServer"={"IPAddress"="127.0.0.1", "Port"=3500}}, {"ID"=49.0, "Name"="C Spot Camera", "DeviceID"={"Slot Connector"=44, "IP Adress"="192.168.10.183", "Port"=63410, "Type"="picodriver"}, "Detection Parameters"={"Contrast"=0, "Treshold"=0, "Max Intensity"=0, "Max Intensity%"=0, "Rx"=0, "Ry"=0, "R%"=0.0}, "Reverse"={"Reverse X"=FALSE, "Reverse Y"=FALSE}, "Target"={"X Target"=0.0, "Y Target"=0.0}, "Region of Interest"=[0, 0, 0, 0], "Correction Parameters"={"X"=0.0, "Y"=0.0, "Movement Type"=0}, "Acquisition Parameters"={"Brightness"=0.0, "Contrast"=0.0, "Saturation"=0.0, "White level"=0.0}, "Background Path"=path "", "Reference Path"=path "", "XCalibration"=[], "YCalibration"=[], "ImageServer"={"IPAddress"="127.0.0.1", "Port"=3500}}, {"ID"=50.0, "Name"="p2s5c1-FREE", "DeviceID"={"Slot Connector"=51, "IP Adress"="192.168.10.183", "Port"=63410, "Type"="picodriver"}, "Detection Parameters"={"Contrast"=0, "Treshold"=0, "Max Intensity"=0, "Max Intensity%"=0, "Rx"=0, "Ry"=0, "R%"=0.0}, "Reverse"={"Reverse X"=FALSE, "Reverse Y"=FALSE}, "Target"={"X Target"=0.0, "Y Target"=0.0}, "Region of Interest"=[0, 0, 0, 0], "Correction Parameters"={"X"=0.0, "Y"=0.0, "Movement Type"=0}, "Acquisition Parameters"={"Brightness"=0.0, "Contrast"=0.0, "Saturation"=0.0, "White level"=0.0}, "Background Path"=path "", "Reference Path"=path "", "XCalibration"=[], "YCalibration"=[], "ImageServer"={"IPAddress"="127.0.0.1", "Port"=3500}}, {"ID"=51.0, "Name"="p2s5c2-FREE", "DeviceID"={"Slot Connector"=52, "IP Adress"="192.168.10.183", "Port"=63410, "Type"="picodriver"}, "Detection Parameters"={"Contrast"=0, "Treshold"=0, "Max Intensity"=0, "Max Intensity%"=0, "Rx"=0, "Ry"=0, "R%"=0.0}, "Reverse"={"Reverse X"=FALSE, "Reverse Y"=FALSE}, "Target"={"X Target"=0.0, "Y Target"=0.0}, "Region of Interest"=[0, 0, 0, 0], "Correction Parameters"={"X"=0.0, "Y"=0.0, "Movement Type"=0}, "Acquisition Parameters"={"Brightness"=0.0, "Contrast"=0.0, "Saturation"=0.0, "White level"=0.0}, "Background Path"=path "", "Reference Path"=path "", "XCalibration"=[], "YCalibration"=[], "ImageServer"={"IPAddress"="127.0.0.1", "Port"=3500}}, {"ID"=52.0, "Name"="p2s5c3-FREE", "DeviceID"={"Slot Connector"=53, "IP Adress"="192.168.10.183", "Port"=63410, "Type"="picodriver"}, "Detection Parameters"={"Contrast"=0, "Treshold"=0, "Max Intensity"=0, "Max Intensity%"=0, "Rx"=0, "Ry"=0, "R%"=0.0}, "Reverse"={"Reverse X"=FALSE, "Reverse Y"=FALSE}, "Target"={"X Target"=0.0, "Y Target"=0.0}, "Region of Interest"=[0, 0, 0, 0], "Correction Parameters"={"X"=0.0, "Y"=0.0, "Movement Type"=0}, "Acquisition Parameters"={"Brightness"=0.0, "Contrast"=0.0, "Saturation"=0.0, "White level"=0.0}, "Background Path"=path "", "Reference Path"=path "", "XCalibration"=[], "YCalibration"=[], "ImageServer"={"IPAddress"="127.0.0.1", "Port"=3500}}, {"ID"=53.0, "Name"="p2c5c4-FREE", "DeviceID"={"Slot Connector"=54, "IP Adress"="192.168.10.183", "Port"=63410, "Type"="picodriver"}, "Detection Parameters"={"Contrast"=0, "Treshold"=0, "Max Intensity"=0, "Max Intensity%"=0, "Rx"=0, "Ry"=0, "R%"=0.0}, "Reverse"={"Reverse X"=FALSE, "Reverse Y"=FALSE}, "Target"={"X Target"=0.0, "Y Target"=0.0}, "Region of Interest"=[0, 0, 0, 0], "Correction Parameters"={"X"=0.0, "Y"=0.0, "Movement Type"=0}, "Acquisition Parameters"={"Brightness"=0.0, "Contrast"=0.0, "Saturation"=0.0, "White level"=0.0}, "Background Path"=path "", "Reference Path"=path "", "XCalibration"=[], "YCalibration"=[], "ImageServer"={"IPAddress"="127.0.0.1", "Port"=3500}}, {"ID"=55.0, "Name"="*100TW M9", "DeviceID"={"Slot Connector"=31, "IP Adress"="192.168.10.34", "Port"=63420, "Type"="picodriver"}, "Detection Parameters"={"Contrast"=0, "Treshold"=0, "Max Intensity"=0, "Max Intensity%"=0, "Rx"=0, "Ry"=0, "R%"=0.0}, "Reverse"={"Reverse X"=FALSE, "Reverse Y"=FALSE}, "Target"={"X Target"=631.0, "Y Target"=473.0}, "Region of Interest"=[0, 0, 0, 0], "Correction Parameters"={"X"=0.0, "Y"=0.0, "Movement Type"=0}, "Acquisition Parameters"={"Brightness"=0.0, "Contrast"=0.0, "Saturation"=0.0, "White level"=0.0}, "Background Path"=path "", "Reference Path"=path "", "XCalibration"=[], "YCalibration"=[], "ImageServer"={"IPAddress"="234.5.6.8", "Port"=58444}}, {"ID"=56.0, "Name"="*100TW M10", "DeviceID"={"Slot Connector"=32, "IP Adress"="192.168.10.34", "Port"=63420, "Type"="picodriver"}, "Detection Parameters"={"Contrast"=53, "Treshold"=53, "Max Intensity"=255, "Max Intensity%"=80, "Rx"=116, "Ry"=92, "R%"=50.0}, "Reverse"={"Reverse X"=FALSE, "Reverse Y"=TRUE}, "Target"={"X Target"=334.0, "Y Target"=206.0}, "Region of Interest"=[0, 0, 0, 0], "Correction Parameters"={"X"=100.0, "Y"=100.0, "Movement Type"=0}, "Acquisition Parameters"={"Brightness"=0.0, "Contrast"=0.0, "Saturation"=0.0, "White level"=0.0}, "Background Path"=path "", "Reference Path"=path "", "XCalibration"=[], "YCalibration"=[], "ImageServer"={"IPAddress"="234.5.6.8", "Port"=58445}}, {"ID"=57.0, "Name"="*100TW Preamp Up", "DeviceID"={"Slot Connector"=11, "IP Adress"="192.168.10.34", "Port"=63420, "Type"="picodriver"}, "Detection Parameters"={"Contrast"=0, "Treshold"=0, "Max Intensity"=0, "Max Intensity%"=0, "Rx"=0, "Ry"=0, "R%"=0.0}, "Reverse"={"Reverse X"=FALSE, "Reverse Y"=FALSE}, "Target"={"X Target"=0.0, "Y Target"=0.0}, "Region of Interest"=[0, 0, 0, 0], "Correction Parameters"={"X"=0.0, "Y"=0.0, "Movement Type"=0}, "Acquisition Parameters"={"Brightness"=0.0, "Contrast"=0.0, "Saturation"=0.0, "White level"=0.0}, "Background Path"=path "", "Reference Path"=path "", "XCalibration"=[], "YCalibration"=[], "ImageServer"={"IPAddress"="127.0.0.1", "Port"=3500}}, {"ID"=58.0, "Name"="*100TW Input Preamp2", "DeviceID"={"Slot Connector"=12, "IP Adress"="192.168.10.34", "Port"=63420, "Type"="picodriver"}, "Detection Parameters"={"Contrast"=0, "Treshold"=0, "Max Intensity"=0, "Max Intensity%"=0, "Rx"=0, "Ry"=0, "R%"=0.0}, "Reverse"={"Reverse X"=FALSE, "Reverse Y"=FALSE}, "Target"={"X Target"=0.0, "Y Target"=0.0}, "Region of Interest"=[0, 0, 0, 0], "Correction Parameters"={"X"=0.0, "Y"=0.0, "Movement Type"=0}, "Acquisition Parameters"={"Brightness"=0.0, "Contrast"=0.0, "Saturation"=0.0, "White level"=0.0}, "Background Path"=path "", "Reference Path"=path "", "XCalibration"=[], "YCalibration"=[], "ImageServer"={"IPAddress"="127.0.0.1", "Port"=3500}}, {"ID"=59.0, "Name"="*100TW Output Preamp2", "DeviceID"={"Slot Connector"=14, "IP Adress"="192.168.10.34", "Port"=63420, "Type"="picodriver"}, "Detection Parameters"={"Contrast"=0, "Treshold"=0, "Max Intensity"=0, "Max Intensity%"=0, "Rx"=0, "Ry"=0, "R%"=0.0}, "Reverse"={"Reverse X"=FALSE, "Reverse Y"=FALSE}, "Target"={"X Target"=0.0, "Y Target"=0.0}, "Region of Interest"=[0, 0, 0, 0], "Correction Parameters"={"X"=0.0, "Y"=0.0, "Movement Type"=0}, "Acquisition Parameters"={"Brightness"=0.0, "Contrast"=0.0, "Saturation"=0.0, "White level"=0.0}, "Background Path"=path "", "Reference Path"=path "", "XCalibration"=[], "YCalibration"=[], "ImageServer"={"IPAddress"="127.0.0.1", "Port"=3500}}, {"ID"=60.0, "Name"="*100TW M0", "DeviceID"={"Slot Connector"=13, "IP Adress"="192.168.10.34", "Port"=63420, "Type"="picodriver"}, "Detection Parameters"={"Contrast"=0, "Treshold"=0, "Max Intensity"=0, "Max Intensity%"=0, "Rx"=0, "Ry"=0, "R%"=0.0}, "Reverse"={"Reverse X"=FALSE, "Reverse Y"=FALSE}, "Target"={"X Target"=0.0, "Y Target"=0.0}, "Region of Interest"=[0, 0, 0, 0], "Correction Parameters"={"X"=0.0, "Y"=0.0, "Movement Type"=0}, "Acquisition Parameters"={"Brightness"=0.0, "Contrast"=0.0, "Saturation"=0.0, "White level"=0.0}, "Background Path"=path "", "Reference Path"=path "", "XCalibration"=[], "YCalibration"=[], "ImageServer"={"IPAddress"="127.0.0.1", "Port"=3500}}, {"ID"=61.0, "Name"="*100TW M2", "DeviceID"={"Slot Connector"=21, "IP Adress"="192.168.10.34", "Port"=63420, "Type"="picodriver"}, "Detection Parameters"={"Contrast"=0, "Treshold"=0, "Max Intensity"=0, "Max Intensity%"=0, "Rx"=0, "Ry"=0, "R%"=0.0}, "Reverse"={"Reverse X"=FALSE, "Reverse Y"=FALSE}, "Target"={"X Target"=0.0, "Y Target"=0.0}, "Region of Interest"=[0, 0, 0, 0], "Correction Parameters"={"X"=0.0, "Y"=0.0, "Movement Type"=0}, "Acquisition Parameters"={"Brightness"=0.0, "Contrast"=0.0, "Saturation"=0.0, "White level"=0.0}, "Background Path"=path "", "Reference Path"=path "", "XCalibration"=[], "YCalibration"=[], "ImageServer"={"IPAddress"="127.0.0.1", "Port"=3500}}, {"ID"=62.0, "Name"="*100TW M4", "DeviceID"={"Slot Connector"=22, "IP Adress"="192.168.10.34", "Port"=63420, "Type"="picodriver"}, "Detection Parameters"={"Contrast"=0, "Treshold"=0, "Max Intensity"=0, "Max Intensity%"=0, "Rx"=0, "Ry"=0, "R%"=0.0}, "Reverse"={"Reverse X"=FALSE, "Reverse Y"=FALSE}, "Target"={"X Target"=0.0, "Y Target"=0.0}, "Region of Interest"=[0, 0, 0, 0], "Correction Parameters"={"X"=0.0, "Y"=0.0, "Movement Type"=0}, "Acquisition Parameters"={"Brightness"=0.0, "Contrast"=0.0, "Saturation"=0.0, "White level"=0.0}, "Background Path"=path "", "Reference Path"=path "", "XCalibration"=[], "YCalibration"=[], "ImageServer"={"IPAddress"="127.0.0.1", "Port"=3500}}, {"ID"=63.0, "Name"="*100TW M6", "DeviceID"={"Slot Connector"=23, "IP Adress"="192.168.10.34", "Port"=63420, "Type"="picodriver"}, "Detection Parameters"={"Contrast"=0, "Treshold"=0, "Max Intensity"=0, "Max Intensity%"=0, "Rx"=0, "Ry"=0, "R%"=0.0}, "Reverse"={"Reverse X"=FALSE, "Reverse Y"=FALSE}, "Target"={"X Target"=0.0, "Y Target"=0.0}, "Region of Interest"=[0, 0, 0, 0], "Correction Parameters"={"X"=0.0, "Y"=0.0, "Movement Type"=0}, "Acquisition Parameters"={"Brightness"=0.0, "Contrast"=0.0, "Saturation"=0.0, "White level"=0.0}, "Background Path"=path "", "Reference Path"=path "", "XCalibration"=[], "YCalibration"=[], "ImageServer"={"IPAddress"="127.0.0.1", "Port"=3500}}, {"ID"=64.0, "Name"="*100TW M8", "DeviceID"={"Slot Connector"=24, "IP Adress"="192.168.10.34", "Port"=63420, "Type"="picodriver"}, "Detection Parameters"={"Contrast"=0, "Treshold"=0, "Max Intensity"=0, "Max Intensity%"=0, "Rx"=0, "Ry"=0, "R%"=0.0}, "Reverse"={"Reverse X"=FALSE, "Reverse Y"=FALSE}, "Target"={"X Target"=0.0, "Y Target"=0.0}, "Region of Interest"=[0, 0, 0, 0], "Correction Parameters"={"X"=0.0, "Y"=0.0, "Movement Type"=0}, "Acquisition Parameters"={"Brightness"=0.0, "Contrast"=0.0, "Saturation"=0.0, "White level"=0.0}, "Background Path"=path "", "Reference Path"=path "", "XCalibration"=[], "YCalibration"=[], "ImageServer"={"IPAddress"="234.5.6.8", "Port"=58450}}, {"ID"=65.0, "Name"="*100TW M13", "DeviceID"={"Slot Connector"=33, "IP Adress"="192.168.10.34", "Port"=63420, "Type"="picodriver"}, "Detection Parameters"={"Contrast"=0, "Treshold"=0, "Max Intensity"=0, "Max Intensity%"=0, "Rx"=0, "Ry"=0, "R%"=0.0}, "Reverse"={"Reverse X"=FALSE, "Reverse Y"=FALSE}, "Target"={"X Target"=0.0, "Y Target"=0.0}, "Region of Interest"=[0, 0, 0, 0], "Correction Parameters"={"X"=0.0, "Y"=0.0, "Movement Type"=0}, "Acquisition Parameters"={"Brightness"=0.0, "Contrast"=0.0, "Saturation"=0.0, "White level"=0.0}, "Background Path"=path "", "Reference Path"=path "", "XCalibration"=[], "YCalibration"=[], "ImageServer"={"IPAddress"="127.0.0.1", "Port"=3500}}, {"ID"=0.0, "Name"="*100TW M20", "DeviceID"={"Slot Connector"=1, "IP Adress"="192.168.10.184", "Port"=63430, "Type"="picodriver"}, "Detection Parameters"={"Contrast"=66, "Treshold"=66, "Max Intensity"=255, "Max Intensity%"=80, "Rx"=30, "Ry"=30, "R%"=50.0}, "Reverse"={"Reverse X"=TRUE, "Reverse Y"=TRUE}, "Target"={"X Target"=295.0, "Y Target"=162.0}, "Region of Interest"=[0, 0, 0, 0], "Correction Parameters"={"X"=20.0, "Y"=20.0, "Movement Type"=0}, "Acquisition Parameters"={"Brightness"=0.0, "Contrast"=0.0, "Saturation"=0.0, "White level"=0.0}, "Background Path"=path "", "Reference Path"=path "", "XCalibration"=[{-23000.0, -242.0}, {-22000.0, -229.0}, {-21000.0, -215.0}, {-20000.0, -203.0}, {-19000.0, -192.0}, {-18000.0, -182.0}, {-17000.0, -172.0}, {-16000.0, -162.0}, {-15000.0, -153.0}, {-14000.0, -141.0}, {-13000.0, -126.0}, {-12000.0, -105.0}, {-11000.0, -77.0}, {-10000.0, -44.0}, {0.0, 4.0}, {11000.0, 98.0}, {12000.0, 109.0}, {13000.0, 119.0}, {14000.0, 130.0}, {15000.0, 140.0}, {16000.0, 151.0}, {17000.0, 161.0}, {18000.0, 171.0}, {19000.0, 182.0}, {20000.0, 193.0}, {21000.0, 205.0}, {22000.0, 217.0}, {23000.0, 229.0}], "YCalibration"=[{-23000.0, 196.0}, {-22000.0, 189.0}, {-21000.0, 182.0}, {-20000.0, 174.0}, {-19000.0, 164.0}, {-18000.0, 153.0}, {-17000.0, 141.0}, {-16000.0, 133.0}, {-15000.0, 126.0}, {-14000.0, 117.0}, {-13000.0, 105.0}, {-12000.0, 90.0}, {-11000.0, 69.0}, {-10000.0, 42.0}, {0.0, -4.0}, {11000.0, -96.0}, {12000.0, -99.0}, {13000.0, -101.0}, {14000.0, -103.0}, {15000.0, -109.0}, {16000.0, -118.0}, {17000.0, -129.0}, {18000.0, -143.0}, {19000.0, -155.0}, {20000.0, -166.0}, {21000.0, -174.0}, {22000.0, -181.0}, {23000.0, -187.0}], "ImageServer"={"IPAddress"="234.5.6.8", "Port"=58443}}, {"ID"=12.0, "Name"="*100TW M22", "DeviceID"={"Slot Connector"=3, "IP Adress"="192.168.10.184", "Port"=63430, "Type"="picodriver"}, "Detection Parameters"={"Contrast"=59, "Treshold"=59, "Max Intensity"=255, "Max Intensity%"=80, "Rx"=47, "Ry"=33, "R%"=50.0}, "Reverse"={"Reverse X"=FALSE, "Reverse Y"=TRUE}, "Target"={"X Target"=319.0, "Y Target"=219.0}, "Region of Interest"=[0, 0, 0, 0], "Correction Parameters"={"X"=10000.0, "Y"=10000.0, "Movement Type"=0}, "Acquisition Parameters"={"Brightness"=0.0, "Contrast"=0.0, "Saturation"=0.0, "White level"=0.0}, "Background Path"=path "", "Reference Path"=path "", "XCalibration"=[], "YCalibration"=[], "ImageServer"={"IPAddress"="234.5.6.8", "Port"=58446}}, {"ID"=12.0, "Name"="*100TW M23", "DeviceID"={"Slot Connector"=4, "IP Adress"="192.168.10.184", "Port"=63430, "Type"="picodriver"}, "Detection Parameters"={"Contrast"=11, "Treshold"=11, "Max Intensity"=255, "Max Intensity%"=90, "Rx"=180, "Ry"=110, "R%"=50.0}, "Reverse"={"Reverse X"=FALSE, "Reverse Y"=TRUE}, "Target"={"X Target"=303.0, "Y Target"=342.0}, "Region of Interest"=[0, 0, 0, 0], "Correction Parameters"={"X"=0.0, "Y"=0.0, "Movement Type"=0}, "Acquisition Parameters"={"Brightness"=0.0, "Contrast"=0.0, "Saturation"=0.0, "White level"=0.0}, "Background Path"=path "", "Reference Path"=path "", "XCalibration"=[], "YCalibration"=[], "ImageServer"={"IPAddress"="234.5.6.8", "Port"=58442}}, {"ID"=6.0, "Name"="no pico", "DeviceID"={"Slot Connector"=0, "IP Adress"="127.0.0.1", "Port"=0, "Type"="picodriver"}, "Detection Parameters"={"Contrast"=0, "Treshold"=0, "Max Intensity"=0, "Max Intensity%"=0, "Rx"=0, "Ry"=0, "R%"=0.0}, "Reverse"={"Reverse X"=FALSE, "Reverse Y"=FALSE}, "Target"={"X Target"=0.0, "Y Target"=0.0}, "Region of Interest"=[0, 0, 0, 0], "Correction Parameters"={"X"=0.0, "Y"=0.0, "Movement Type"=0}, "Acquisition Parameters"={"Brightness"=0.0, "Contrast"=0.0, "Saturation"=0.0, "White level"=0.0}, "Background Path"=path "", "Reference Path"=path "", "XCalibration"=[], "YCalibration"=[], "ImageServer"={"IPAddress"="127.0.0.1", "Port"=3500}}, {"ID"=6.0, "Name"="no pico", "DeviceID"={"Slot Connector"=0, "IP Adress"="127.0.0.1", "Port"=0, "Type"="picodriver"}, "Detection Parameters"={"Contrast"=0, "Treshold"=0, "Max Intensity"=0, "Max Intensity%"=0, "Rx"=0, "Ry"=0, "R%"=0.0}, "Reverse"={"Reverse X"=FALSE, "Reverse Y"=FALSE}, "Target"={"X Target"=0.0, "Y Target"=0.0}, "Region of Interest"=[0, 0, 0, 0], "Correction Parameters"={"X"=0.0, "Y"=0.0, "Movement Type"=0}, "Acquisition Parameters"={"Brightness"=0.0, "Contrast"=0.0, "Saturation"=0.0, "White level"=0.0}, "Background Path"=path "", "Reference Path"=path "", "XCalibration"=[], "YCalibration"=[], "ImageServer"={"IPAddress"="127.0.0.1", "Port"=3500}}, {"ID"=6.0, "Name"="no pico", "DeviceID"={"Slot Connector"=0, "IP Adress"="127.0.0.1", "Port"=0, "Type"="picodriver"}, "Detection Parameters"={"Contrast"=0, "Treshold"=0, "Max Intensity"=0, "Max Intensity%"=0, "Rx"=0, "Ry"=0, "R%"=0.0}, "Reverse"={"Reverse X"=FALSE, "Reverse Y"=FALSE}, "Target"={"X Target"=0.0, "Y Target"=0.0}, "Region of Interest"=[0, 0, 0, 0], "Correction Parameters"={"X"=0.0, "Y"=0.0, "Movement Type"=0}, "Acquisition Parameters"={"Brightness"=0.0, "Contrast"=0.0, "Saturation"=0.0, "White level"=0.0}, "Background Path"=path "", "Reference Path"=path "", "XCalibration"=[], "YCalibration"=[], "ImageServer"={"IPAddress"="127.0.0.1", "Port"=3500}}, {"ID"=6.0, "Name"="mobile no ir", "DeviceID"={"Slot Connector"=0, "IP Adress"="127.0.0.1", "Port"=0, "Type"="picodriver"}, "Detection Parameters"={"Contrast"=0, "Treshold"=0, "Max Intensity"=0, "Max Intensity%"=0, "Rx"=0, "Ry"=0, "R%"=0.0}, "Reverse"={"Reverse X"=FALSE, "Reverse Y"=FALSE}, "Target"={"X Target"=0.0, "Y Target"=0.0}, "Region of Interest"=[0, 0, 0, 0], "Correction Parameters"={"X"=0.0, "Y"=0.0, "Movement Type"=0}, "Acquisition Parameters"={"Brightness"=0.0, "Contrast"=0.0, "Saturation"=0.0, "White level"=0.0}, "Background Path"=path "", "Reference Path"=path "", "XCalibration"=[], "YCalibration"=[], "ImageServer"={"IPAddress"="127.0.0.1", "Port"=3500}}, {"ID"=1.0, "Name"="regen out-salad#1", "DeviceID"={"Slot Connector"=11, "IP Adress"="192.168.10.11", "Port"=63450, "Type"="picodriver"}, "Detection Parameters"={"Contrast"=0, "Treshold"=0, "Max Intensity"=0, "Max Intensity%"=0, "Rx"=0, "Ry"=0, "R%"=0.0}, "Reverse"={"Reverse X"=FALSE, "Reverse Y"=FALSE}, "Target"={"X Target"=0.0, "Y Target"=0.0}, "Region of Interest"=[0, 0, 0, 0], "Correction Parameters"={"X"=0.0, "Y"=0.0, "Movement Type"=0}, "Acquisition Parameters"={"Brightness"=0.0, "Contrast"=0.0, "Saturation"=0.0, "White level"=0.0}, "Background Path"=path "", "Reference Path"=path "", "XCalibration"=[], "YCalibration"=[], "ImageServer"={"IPAddress"="127.0.0.1", "Port"=3500}}, {"ID"=2.0, "Name"="preamp in-salad#2", "DeviceID"={"Slot Connector"=12, "IP Adress"="192.168.10.11", "Port"=63450, "Type"="picodriver"}, "Detection Parameters"={"Contrast"=0, "Treshold"=0, "Max Intensity"=0, "Max Intensity%"=0, "Rx"=0, "Ry"=0, "R%"=0.0}, "Reverse"={"Reverse X"=FALSE, "Reverse Y"=FALSE}, "Target"={"X Target"=0.0, "Y Target"=0.0}, "Region of Interest"=[0, 0, 0, 0], "Correction Parameters"={"X"=0.0, "Y"=0.0, "Movement Type"=0}, "Acquisition Parameters"={"Brightness"=0.0, "Contrast"=0.0, "Saturation"=0.0, "White level"=0.0}, "Background Path"=path "", "Reference Path"=path "", "XCalibration"=[], "YCalibration"=[], "ImageServer"={"IPAddress"="127.0.0.1", "Port"=3500}}, {"ID"=3.0, "Name"="XPW 1", "DeviceID"={"Slot Connector"=13, "IP Adress"="192.168.10.11", "Port"=63450, "Type"="picodriver"}, "Detection Parameters"={"Contrast"=0, "Treshold"=0, "Max Intensity"=0, "Max Intensity%"=0, "Rx"=0, "Ry"=0, "R%"=0.0}, "Reverse"={"Reverse X"=FALSE, "Reverse Y"=FALSE}, "Target"={"X Target"=0.0, "Y Target"=0.0}, "Region of Interest"=[0, 0, 0, 0], "Correction Parameters"={"X"=0.0, "Y"=0.0, "Movement Type"=0}, "Acquisition Parameters"={"Brightness"=0.0, "Contrast"=0.0, "Saturation"=0.0, "White level"=0.0}, "Background Path"=path "", "Reference Path"=path "", "XCalibration"=[], "YCalibration"=[], "ImageServer"={"IPAddress"="127.0.0.1", "Port"=3500}}, {"ID"=4.0, "Name"="blue periscope regen", "DeviceID"={"Slot Connector"=14, "IP Adress"="192.168.10.11", "Port"=63450, "Type"="picodriver"}, "Detection Parameters"={"Contrast"=0, "Treshold"=0, "Max Intensity"=0, "Max Intensity%"=0, "Rx"=0, "Ry"=0, "R%"=0.0}, "Reverse"={"Reverse X"=FALSE, "Reverse Y"=FALSE}, "Target"={"X Target"=0.0, "Y Target"=0.0}, "Region of Interest"=[0, 0, 0, 0], "Correction Parameters"={"X"=0.0, "Y"=0.0, "Movement Type"=0}, "Acquisition Parameters"={"Brightness"=0.0, "Contrast"=0.0, "Saturation"=0.0, "White level"=0.0}, "Background Path"=path "", "Reference Path"=path "", "XCalibration"=[], "YCalibration"=[], "ImageServer"={"IPAddress"="127.0.0.1", "Port"=3500}}, {"ID"=8.0, "Name"="godzilla 1st", "DeviceID"={"Slot Connector"=22, "IP Adress"="192.168.10.11", "Port"=63450, "Type"="picodriver"}, "Detection Parameters"={"Contrast"=0, "Treshold"=0, "Max Intensity"=0, "Max Intensity%"=0, "Rx"=0, "Ry"=0, "R%"=0.0}, "Reverse"={"Reverse X"=FALSE, "Reverse Y"=FALSE}, "Target"={"X Target"=0.0, "Y Target"=0.0}, "Region of Interest"=[0, 0, 0, 0], "Correction Parameters"={"X"=0.0, "Y"=0.0, "Movement Type"=0}, "Acquisition Parameters"={"Brightness"=0.0, "Contrast"=0.0, "Saturation"=0.0, "White level"=0.0}, "Background Path"=path "", "Reference Path"=path "", "XCalibration"=[], "YCalibration"=[], "ImageServer"={"IPAddress"="127.0.0.1", "Port"=3500}}, {"ID"=9.0, "Name"="godzilla IN", "DeviceID"={"Slot Connector"=21, "IP Adress"="192.168.10.11", "Port"=63450, "Type"="picodriver"}, "Detection Parameters"={"Contrast"=0, "Treshold"=0, "Max Intensity"=0, "Max Intensity%"=0, "Rx"=0, "Ry"=0, "R%"=0.0}, "Reverse"={"Reverse X"=FALSE, "Reverse Y"=FALSE}, "Target"={"X Target"=0.0, "Y Target"=0.0}, "Region of Interest"=[0, 0, 0, 0], "Correction Parameters"={"X"=0.0, "Y"=0.0, "Movement Type"=0}, "Acquisition Parameters"={"Brightness"=0.0, "Contrast"=0.0, "Saturation"=0.0, "White level"=0.0}, "Background Path"=path "", "Reference Path"=path "", "XCalibration"=[], "YCalibration"=[], "ImageServer"={"IPAddress"="127.0.0.1", "Port"=3500}}, {"ID"=10.0, "Name"="Chihuahua IN", "DeviceID"={"Slot Connector"=23, "IP Adress"="192.168.10.11", "Port"=63450, "Type"="picodriver"}, "Detection Parameters"={"Contrast"=0, "Treshold"=0, "Max Intensity"=0, "Max Intensity%"=0, "Rx"=0, "Ry"=0, "R%"=0.0}, "Reverse"={"Reverse X"=FALSE, "Reverse Y"=FALSE}, "Target"={"X Target"=0.0, "Y Target"=0.0}, "Region of Interest"=[0, 0, 0, 0], "Correction Parameters"={"X"=0.0, "Y"=0.0, "Movement Type"=0}, "Acquisition Parameters"={"Brightness"=0.0, "Contrast"=0.0, "Saturation"=0.0, "White level"=0.0}, "Background Path"=path "", "Reference Path"=path "", "XCalibration"=[], "YCalibration"=[], "ImageServer"={"IPAddress"="127.0.0.1", "Port"=3500}}, {"ID"=11.0, "Name"="Chihuahua 1st", "DeviceID"={"Slot Connector"=24, "IP Adress"="192.168.10.11", "Port"=63450, "Type"="picodriver"}, "Detection Parameters"={"Contrast"=0, "Treshold"=0, "Max Intensity"=0, "Max Intensity%"=0, "Rx"=0, "Ry"=0, "R%"=0.0}, "Reverse"={"Reverse X"=FALSE, "Reverse Y"=FALSE}, "Target"={"X Target"=0.0, "Y Target"=0.0}, "Region of Interest"=[0, 0, 0, 0], "Correction Parameters"={"X"=0.0, "Y"=0.0, "Movement Type"=0}, "Acquisition Parameters"={"Brightness"=0.0, "Contrast"=0.0, "Saturation"=0.0, "White level"=0.0}, "Background Path"=path "", "Reference Path"=path "", "XCalibration"=[], "YCalibration"=[], "ImageServer"={"IPAddress"="127.0.0.1", "Port"=3500}}, {"ID"=12.0, "Name"="??XPW pico2", "DeviceID"={"Slot Connector"=34, "IP Adress"="192.168.10.11", "Port"=63450, "Type"="picodriver"}, "Detection Parameters"={"Contrast"=0, "Treshold"=0, "Max Intensity"=0, "Max Intensity%"=0, "Rx"=0, "Ry"=0, "R%"=0.0}, "Reverse"={"Reverse X"=FALSE, "Reverse Y"=FALSE}, "Target"={"X Target"=0.0, "Y Target"=0.0}, "Region of Interest"=[0, 0, 0, 0], "Correction Parameters"={"X"=0.0, "Y"=0.0, "Movement Type"=0}, "Acquisition Parameters"={"Brightness"=0.0, "Contrast"=0.0, "Saturation"=0.0, "White level"=0.0}, "Background Path"=path "", "Reference Path"=path "", "XCalibration"=[], "YCalibration"=[], "ImageServer"={"IPAddress"="127.0.0.1", "Port"=3500}}, {"ID"=13.0, "Name"="Preamp 3rd pass", "DeviceID"={"Slot Connector"=31, "IP Adress"="192.168.10.11", "Port"=63450, "Type"="picodriver"}, "Detection Parameters"={"Contrast"=0, "Treshold"=0, "Max Intensity"=0, "Max Intensity%"=0, "Rx"=0, "Ry"=0, "R%"=0.0}, "Reverse"={"Reverse X"=FALSE, "Reverse Y"=FALSE}, "Target"={"X Target"=0.0, "Y Target"=0.0}, "Region of Interest"=[0, 0, 0, 0], "Correction Parameters"={"X"=0.0, "Y"=0.0, "Movement Type"=0}, "Acquisition Parameters"={"Brightness"=0.0, "Contrast"=0.0, "Saturation"=0.0, "White level"=0.0}, "Background Path"=path "", "Reference Path"=path "", "XCalibration"=[], "YCalibration"=[], "ImageServer"={"IPAddress"="127.0.0.1", "Port"=3500}}, {"ID"=14.0, "Name"="Blue regen out", "DeviceID"={"Slot Connector"=33, "IP Adress"="192.168.10.11", "Port"=63450, "Type"="picodriver"}, "Detection Parameters"={"Contrast"=0, "Treshold"=0, "Max Intensity"=0, "Max Intensity%"=0, "Rx"=0, "Ry"=0, "R%"=0.0}, "Reverse"={"Reverse X"=FALSE, "Reverse Y"=FALSE}, "Target"={"X Target"=0.0, "Y Target"=0.0}, "Region of Interest"=[0, 0, 0, 0], "Correction Parameters"={"X"=0.0, "Y"=0.0, "Movement Type"=0}, "Acquisition Parameters"={"Brightness"=0.0, "Contrast"=0.0, "Saturation"=0.0, "White level"=0.0}, "Background Path"=path "", "Reference Path"=path "", "XCalibration"=[], "YCalibration"=[], "ImageServer"={"IPAddress"="127.0.0.1", "Port"=3500}}] {"Acquisition Parameters"."White level" scale=0.3..1.26 scale format="%#_2f"; "Acquisition Parameters"."Saturation" scale=0.5..1.5 scale format="%#_3f"; "Acquisition Parameters"."Contrast" scale=0.4..1.5 scale format="%#_3f"; "Acquisition Parameters"."Brightness" scale=-50.0..50.0 scale format="%#_2f"; "Correction Parameters"."Movement Type" items=["Step", "Proportionnal"]; "Target"."X Target" format="%#_5g"; "Target"."Y Target" format="%#_5g"; "Detection Parameters"."Max Intensity%" max=100 step=1}
  out "Images for analysis":T1[](array[typedef])=["imageserver0", "imageserver1", "imageserver2", "imageserver3", "imageserver4", "imageserver5"]
  out "history last shots":T17(array[cluster])
  out "Fancy Display":picture
  in  "Main tab":T18(tab)=enum."Expert Configure"
  out "Detection status":string[](array[string])
  out "MirrorsNames":string[](array[string])
  in  "CamOn":bool[](array[boolean])=[FALSE, FALSE, FALSE, FALSE, FALSE, FALSE, FALSE, FALSE, FALSE]
  in  "Auto":bool[](array[boolean])=[FALSE, FALSE, FALSE, FALSE, FALSE, FALSE, FALSE, FALSE, FALSE]
  out "Last Move":string[](array[string])
  out "element 9":string
  out "element 8":string
  out "element 7":string
  out "element 6":string
  out "element 5":string
  out "element 4":string
  out "element 3":string
  out "element 2":string
  out "Image 9":T1(plugin-control) caption="no cam"
  out "Image 8":T1(plugin-control) caption="no cam"
  out "Image 7":T1(plugin-control) caption="no cam"
  out "Image 6":T1(plugin-control) caption="no cam"
  out "Image 5":T1(plugin-control) caption="no cam"
  out "Image 4":T1(plugin-control) caption="no cam"
  out "Image 3":T1(plugin-control) caption="no cam"
  out "Image 2":T1(plugin-control) caption="no cam"
  out "Image":T1(plugin-control) caption="no cam"
  out "element":string
  out "History Display 2":cluster{timestamp[], dbl[]}[](graph)
  in  "History # of points":i32=1000
  out "History Display 3":cluster{timestamp[], dbl[]}[](graph)
  out "History Display 4":cluster{timestamp[], dbl[]}[](graph)
  out "History Display 5":cluster{timestamp[], dbl[]}[](graph)
  out "History Display 6":cluster{timestamp[], dbl[]}[](graph)
  out "History Display 7":cluster{timestamp[], dbl[]}[](graph)
  out "History Display 8":cluster{timestamp[], dbl[]}[](graph)
  out "History Display 9":cluster{timestamp[], dbl[]}[](graph)
  out "History Display 10":cluster{timestamp[], dbl[]}[](graph)
  out "will move":bool caption="Move In Progress"
  in  "Image Selector":u16(ring) items=["Acquired Image", "Averaged Image", "Thresholded Image"]
  in  "Tab Control":T19(tab)=enum."Correction"
  in  "Tab Control 4":enum32{"User", "Advanced 1", "Advanced 2"}(tab)
  in  "Auto Detect Param":bool
  in  "Set Target (Cursor)":bool
  in  "Set Centroid as Target":bool
  in  "Target":cluster{"X Target":sgl, "Y Target":sgl}={"X Target"=334.0, "Y Target"=206.0} {"X Target" format="%#_5g"; "Y Target" format="%#_5g"}
  in  "Grab reference Image":bool
  in  "Grab Backround Image":bool
  in  "Substract":u16(ring) items=["None", "Background", "Reference"]
  in  "Reset ROI":bool
  in  "Select ROI":bool
  in  "smooth":bool=TRUE
  in  "Size & Tolerance":T20={"X Size"=5, "Y Size"=5, "% Tolerance"=10}
  out "Centroid Detection":bool=TRUE caption="Detection"
  in  "Detection Parameters":T21={"Contrast"=53, "Treshold"=53, "Max Intensity"=255, "Max Intensity%"=80, "Rx"=116, "Ry"=92, "R%"=50.0} {"Max Intensity%" max=100 step=1}
  out "Img Data":T22 caption="Current Image Data" {"Centroid"."X" format="%#_5g"; "Centroid"."Y" format="%#_5g"; "Max Intensity" format="%#_4g"; "Radius"."Rx" format="%#_5g"; "Radius"."Ry" format="%#_5g"}
  out "ImgData Avg":T23={"Centroid Avg"={"X"=334.0, "Y"=201.0}, "Max Intensity Avg"=255.0, "Radius Avg"={"Rx"=122.0, "Ry"=109.0}} caption="Data Average" {"Centroid Avg"."X" format="%#_5g"; "Centroid Avg"."Y" format="%#_5g"; "Max Intensity Avg" format="%#_4g"; "Radius Avg"."Rx" format="%#_5g"; "Radius Avg"."Ry" format="%#_5g"}
  in  "Pretreatment":bool
  in  "milliseconds to wait":u32
  in  "# imgs/trigger":i32=3 caption="# imgs grabbed after trigger"
  in  "Avg data/ data of avg img":bool
  in  "Tab Control 3":enum32{"User", "Advanced 1", "Advanced 2"}(tab)
  in  "# imgs to avg":i32=10
  in  "Initiate Correction Range":i16=3 min=0 max=100 step=1
  in  "Correction Parameters":cluster{"X":sgl, "Y":sgl, "Movement Type":u16}={"X"=100.0, "Y"=100.0, "Movement Type"=0} {"Movement Type" items=["Step", "Proportionnal"]}
  out "Move":bool
  in  "Calibrate":bool
  out "% XY State True":cluster{"X":dbl, "Y":dbl}={"X"=0.0, "Y"=100.0}
  in  "Threshold [%]":dbl=50.0
  in  "use % Out of Range":bool
  in  "use Avg Out of Range?":bool=TRUE
  out "Out of Range?":cluster{"Dev. X":bool, "Dev. Y":bool}
  out "%Out of Range":cluster{"Dev. X":bool, "Dev. Y":bool}
  in  "Auto Time Out (ms)":u32=10000
  in  "Min time between moves (s)":u32=5
  in  "Mirrors":u8[](array[ring])=[50, 41, 42, 52, 53, 54]
  in  "UDP timeout ms":i32=200
  out "#loops waiting for new image":i32
  out "# loops waiting 4 move":i32
  in  "Reverse":cluster{"Reverse X":bool, "Reverse Y":bool}={"Reverse X"=FALSE, "Reverse Y"=TRUE}
  in  "Fancy Display Options":T24
  in  "Target Area  Display":T25={"Show Variance"=FALSE, "Show Target Reached"=TRUE, "Show Init Correction"=TRUE}
  in  "Display":T26={"Show Best Rect"=TRUE, "Show Centroid"=TRUE, "Show Avg Centroid"=FALSE, "Show Target"=FALSE, "Show Target Area"=TRUE}
  in  "Open CamCenter":bool
  in  "Set Color Map":bool
  in  "Acquisition Parameters":T27 {"White level" scale=0.3..1.26 scale format="%#_2f"; "Saturation" scale=0.5..1.5 scale format="%#_3f"; "Contrast" scale=0.4..1.5 scale format="%#_3f"; "Brightness" scale=-50.0..50.0 scale format="%#_2f"}
  in  "Graph":T28(tab)=enum."X Cal"
  out "X Intensity":u8[](graph)
  out "Y Intensity":u8[][](graph)
  out "Target Area":cluster{dbl[], dbl[]}[](graph)=[{[0.0, 0.0006342391823892943, 0.0012659245074418742, 0.0018925124013031524, 0.002511479815674843, 0.0031203343872399612, 0.0037166244735302428, 0.004297949024825067, 0.004861967252331248, 0.005406408053713336, 0.005929079158021155, 0.006427875953191165, 0.0069007899605764405, 0.00734591692238129, 0.0077614644694353144, 0.008145759338431443, 0.008497254109566709, 0.00881453343745564, 0.009096319750226588, 0.00934147839385275, 0.009549022201003456, 0.009718115466018603, 0.009848077310000394, 0.009938384422472335, 0.009988673168565831, 0.009998741053249468, 0.009968547536705018, 0.009898214197566995, 0.009788024243368392, 0.009638421370163911, 0.009450007975922542, 0.009223542734883563, 0.008959937542643143, 0.008660253844272625, 0.00832569836025385, 0.007957618227441692, 0.007557495574619389, 0.00712694155448907, 0.006667689856128432, 0.0061815897240367545, 0.005670598511879952, 0.005136773800918219, 0.004582265114852496, 0.004009305264451178, 0.0034202013568092296, 0.0028173255054421632, 0.0022031052786221665, 0.0015800139244174349, 0.0009505604117951475, 0.0003172793278889308, -0.00031727932788892837, -0.000950560411795145, -0.0015800139244174323, -0.0022031052786221643, -0.00281732550544216, -0.0034202013568092274, -0.004009305264451176, -0.004582265114852494, -0.005136773800918217, -0.00567059851187995, -0.006181589724036752, -0.0066676898561284295, -0.007126941554489069, -0.0075574955746193885, -0.007957618227441688, -0.008325698360253849, -0.008660253844272622, -0.008959937542643145, -0.009223542734883563, -0.00945000797592254, -0.00963842137016391, -0.009788024243368392, -0.009898214197566995, -0.009968547536705017, -0.009998741053249468, -0.009988673168565831, -0.009938384422472335, -0.009848077310000395, -0.009718115466018607, -0.009549022201003456, -0.00934147839385275, -0.009096319750226591, -0.00881453343745564, -0.008497254109566709, -0.008145759338431445, -0.007761464469435318, -0.00734591692238129, -0.006900789960576441, -0.006427875953191169, -0.00592907915802116, -0.005406408053713335, -0.004861967252331249, -0.0042979490248250705, -0.0037166244735302484, -0.0031203343872399604, -0.002511479815674844, -0.0018925124013031568, -0.001265924507441881, -0.0006342391823892944, -2.4492126529005845e-18], [0.009999999776482582, 0.00997986654165144, 0.009919547906588775, 0.009819286753148901, 0.009679486797610168, 0.009500710965052011, 0.009283679122654322, 0.009029265181046405, 0.008738493575377293, 0.008412535140276995, 0.008052702395318658, 0.007660444259965505, 0.0072373402192835385, 0.00678509396391265, 0.006305526529905721, 0.005800568966059159, 0.005272254558260948, 0.004722710642166016, 0.004154150037166373, 0.0035688621361484323, 0.0029692036869158737, 0.0023575893023980443, 0.0017364817378559118, 0.0011083819742358427, 0.0004758191476020371, -0.0001586596348017588, -0.0007924995508541375, -0.0014231483509230048, -0.0020480666348740477, -0.0026647380773388092, -0.00327067956006883, -0.003863451170576422, -0.004440666026801119, -0.0049999998882412884, -0.0055392005148503206, -0.006056096736012351, -0.00654860719308007, -0.007014748720271355, -0.007452644330177961, -0.007860530771731315, -0.008236765630192265, -0.008579833940575534, -0.008888354287879029, -0.0091610843695545, -0.009396925997821414, -0.009594929521681582, -0.009754297650828523, -0.009874388666054152, -0.009954719003225532, -0.009994965200426965, -0.009994965200426965, -0.009954719003225532, -0.009874388666054154, -0.009754297650828523, -0.009594929521681584, -0.009396925997821416, -0.0091610843695545, -0.00888835428787903, -0.008579833940575534, -0.008236765630192265, -0.007860530771731315, -0.007452644330177963, -0.007014748720271357, -0.006548607193080072, -0.006056096736012352, -0.005539200514850322, -0.004999999888241295, -0.004440666026801117, -0.003863451170576422, -0.0032706795600688323, -0.002664738077338816, -0.0020480666348740477, -0.0014231483509230072, -0.0007924995508541421, -0.0001586596348017657, 0.00047581914760203687, 0.0011083819742358403, 0.0017364817378559075, 0.002357589302398038, 0.0029692036869158737, 0.00356886213614843, 0.0041541500371663695, 0.004722710642166017, 0.005272254558260948, 0.005800568966059157, 0.006305526529905717, 0.006785093963912651, 0.007237340219283538, 0.007660444259965502, 0.008052702395318655, 0.008412535140276995, 0.008738493575377293, 0.009029265181046402, 0.00928367912265432, 0.009500710965052011, 0.009679486797610168, 0.0098192867531489, 0.009919547906588774, 0.00997986654165144, 0.009999999776482582]}, {[], []}, {[nan, nan, nan, nan, nan, nan, nan, nan, nan, nan, nan, nan, nan, nan, nan, nan, nan, nan, nan, nan, nan, nan, nan, nan, nan, nan, nan, nan, nan, nan, nan, nan, nan, nan, nan, nan, nan, nan, nan, nan, nan, nan, nan, nan, nan, nan, nan, nan, nan, nan, nan, nan, nan, nan, nan, nan, nan, nan, nan, nan, nan, nan, nan, nan, nan, nan, nan, nan, nan, nan, nan, nan, nan, nan, nan, nan, nan, nan, nan, nan, nan, nan, nan, nan, nan, nan, nan, nan, nan, nan, nan, nan, nan, nan, nan, nan, nan, nan, nan, nan], [nan, nan, nan, nan, nan, nan, nan, nan, nan, nan, nan, nan, nan, nan, nan, nan, nan, nan, nan, nan, nan, nan, nan, nan, nan, nan, nan, nan, nan, nan, nan, nan, nan, nan, nan, nan, nan, nan, nan, nan, nan, nan, nan, nan, nan, nan, nan, nan, nan, nan, nan, nan, nan, nan, nan, nan, nan, nan, nan, nan, nan, nan, nan, nan, nan, nan, nan, nan, nan, nan, nan, nan, nan, nan, nan, nan, nan, nan, nan, nan, nan, nan, nan, nan, nan, nan, nan, nan, nan, nan, nan, nan, nan, nan, nan, nan, nan, nan, nan, nan]}]
  out "History Display":T17(graph)=[{"seconds since 1Jan1904"=timestamp(3366343832.03125 s since 1904-01-01), "number: 0 to 1"=334.0, "number: 0 to 1"=201.0}, {"seconds since 1Jan1904"=timestamp(3366343831.828125 s since 1904-01-01), "number: 0 to 1"=334.0, "number: 0 to 1"=201.0}, {"seconds since 1Jan1904"=timestamp(3366343831.71875 s since 1904-01-01), "number: 0 to 1"=334.0, "number: 0 to 1"=201.0}, {"seconds since 1Jan1904"=timestamp(3366343831.59375 s since 1904-01-01), "number: 0 to 1"=334.0, "number: 0 to 1"=201.0}, {"seconds since 1Jan1904"=timestamp(3366343831.484375 s since 1904-01-01), "number: 0 to 1"=334.0, "number: 0 to 1"=201.0}, {"seconds since 1Jan1904"=timestamp(3366343831.359375 s since 1904-01-01), "number: 0 to 1"=334.0, "number: 0 to 1"=201.0}, {"seconds since 1Jan1904"=timestamp(3366343831.21875 s since 1904-01-01), "number: 0 to 1"=334.0, "number: 0 to 1"=201.0}, {"seconds since 1Jan1904"=timestamp(3366343831.09375 s since 1904-01-01), "number: 0 to 1"=334.0, "number: 0 to 1"=201.0}, {"seconds since 1Jan1904"=timestamp(3366343830.984375 s since 1904-01-01), "number: 0 to 1"=334.0, "number: 0 to 1"=201.0}, {"seconds since 1Jan1904"=timestamp(3366343830.859375 s since 1904-01-01), "number: 0 to 1"=334.0, "number: 0 to 1"=201.0}, {"seconds since 1Jan1904"=timestamp(3366343830.734375 s since 1904-01-01), "number: 0 to 1"=334.0, "number: 0 to 1"=201.0}, {"seconds since 1Jan1904"=timestamp(3366343830.59375 s since 1904-01-01), "number: 0 to 1"=334.0, "number: 0 to 1"=201.0}, {"seconds since 1Jan1904"=timestamp(3366343830.46875 s since 1904-01-01), "number: 0 to 1"=334.0, "number: 0 to 1"=201.0}, {"seconds since 1Jan1904"=timestamp(3366343830.359375 s since 1904-01-01), "number: 0 to 1"=334.0, "number: 0 to 1"=201.0}, {"seconds since 1Jan1904"=timestamp(3366343830.234375 s since 1904-01-01), "number: 0 to 1"=334.0, "number: 0 to 1"=201.0}, {"seconds since 1Jan1904"=timestamp(3366343830.109375 s since 1904-01-01), "number: 0 to 1"=334.0, "number: 0 to 1"=201.0}, {"seconds since 1Jan1904"=timestamp(3366343829.96875 s since 1904-01-01), "number: 0 to 1"=334.0, "number: 0 to 1"=201.0}, {"seconds since 1Jan1904"=timestamp(3366343829.859375 s since 1904-01-01), "number: 0 to 1"=334.0, "number: 0 to 1"=201.0}, {"seconds since 1Jan1904"=timestamp(3366343829.734375 s since 1904-01-01), "number: 0 to 1"=334.0, "number: 0 to 1"=201.0}, {"seconds since 1Jan1904"=timestamp(3366343829.578125 s since 1904-01-01), "number: 0 to 1"=334.0, "number: 0 to 1"=201.0}]
  out "X calibration":cluster{dbl, dbl}[](graph)
  out "Y calibration":cluster{dbl, dbl}[](graph)
  out "Displayed Image":u8[][](graph)
  in  "restart":bool
  out "conn req":bool caption="Move In Progress"
  out "MoveInProgress 2":bool caption="Move In Progress"
  out "Image IP":string
  out "Image to save":u8[][](graph)
  in  "Save Changes?":bool=TRUE
  out "Warning !":string="Warning : The beam has not been detected, so the averaged and tresholded images have not been calculated"
  in  "stop":bool
  out "USB cameras Indic":i32(listbox)=1 caption="USB cameras"
  # "Beam Pointing 20120418, LOASIS Program"
  # "Times"
  # "MOTOR/CAMERA LIST"
  # "CONTROLS"
  # "INDICATORS"
  # "loop mode diagnostics"
  # "px"
  # "px"
  # "Int"
  # "Int"
  # "Int"
  # "% of Max"
  # "px"
  # "px"
  # "% of Radius"
  # "Int"
  # "Int"
  # "% of Radius"
  # "Detection settings :                                                                                                                                                                         - contrast : This parameter is used during the edge detection of the beam. Contrast specifies the threshold for the contrast of the edge. Only edges with a contrast greater than this value are used in the detection process. Contrast is defined as the difference between the average pixel intensity before the edge and the average pixel intensity after the edge.                                                                                                                                                                                     - The treshold value is used during the processing of the tresholded image. Each pixel intensity value (ranged between 0 and 255) below this parameter will be set to 0, and each pixel above this value will be set to 255.                                                     - Max intensity is maximum intensity of the beam.                                                                                                                         - Max Intensity % is the tolerance about the beam maximum intensity. Practically, to be detected, the peak intensity in the picture must be ranged between Max intensity +/- Max intensity %                                                                                             - Rx is the beam radius on the X axis (in pixels).                                                                                                                                             - Ry is the beam radius on the Y axis (in pixels).                                                                                                                                             - R% is the tolerance about the beam radius. Practically, the X and Y radius must respectively be comprised between Rx +/- R% and Ry +/- R%"
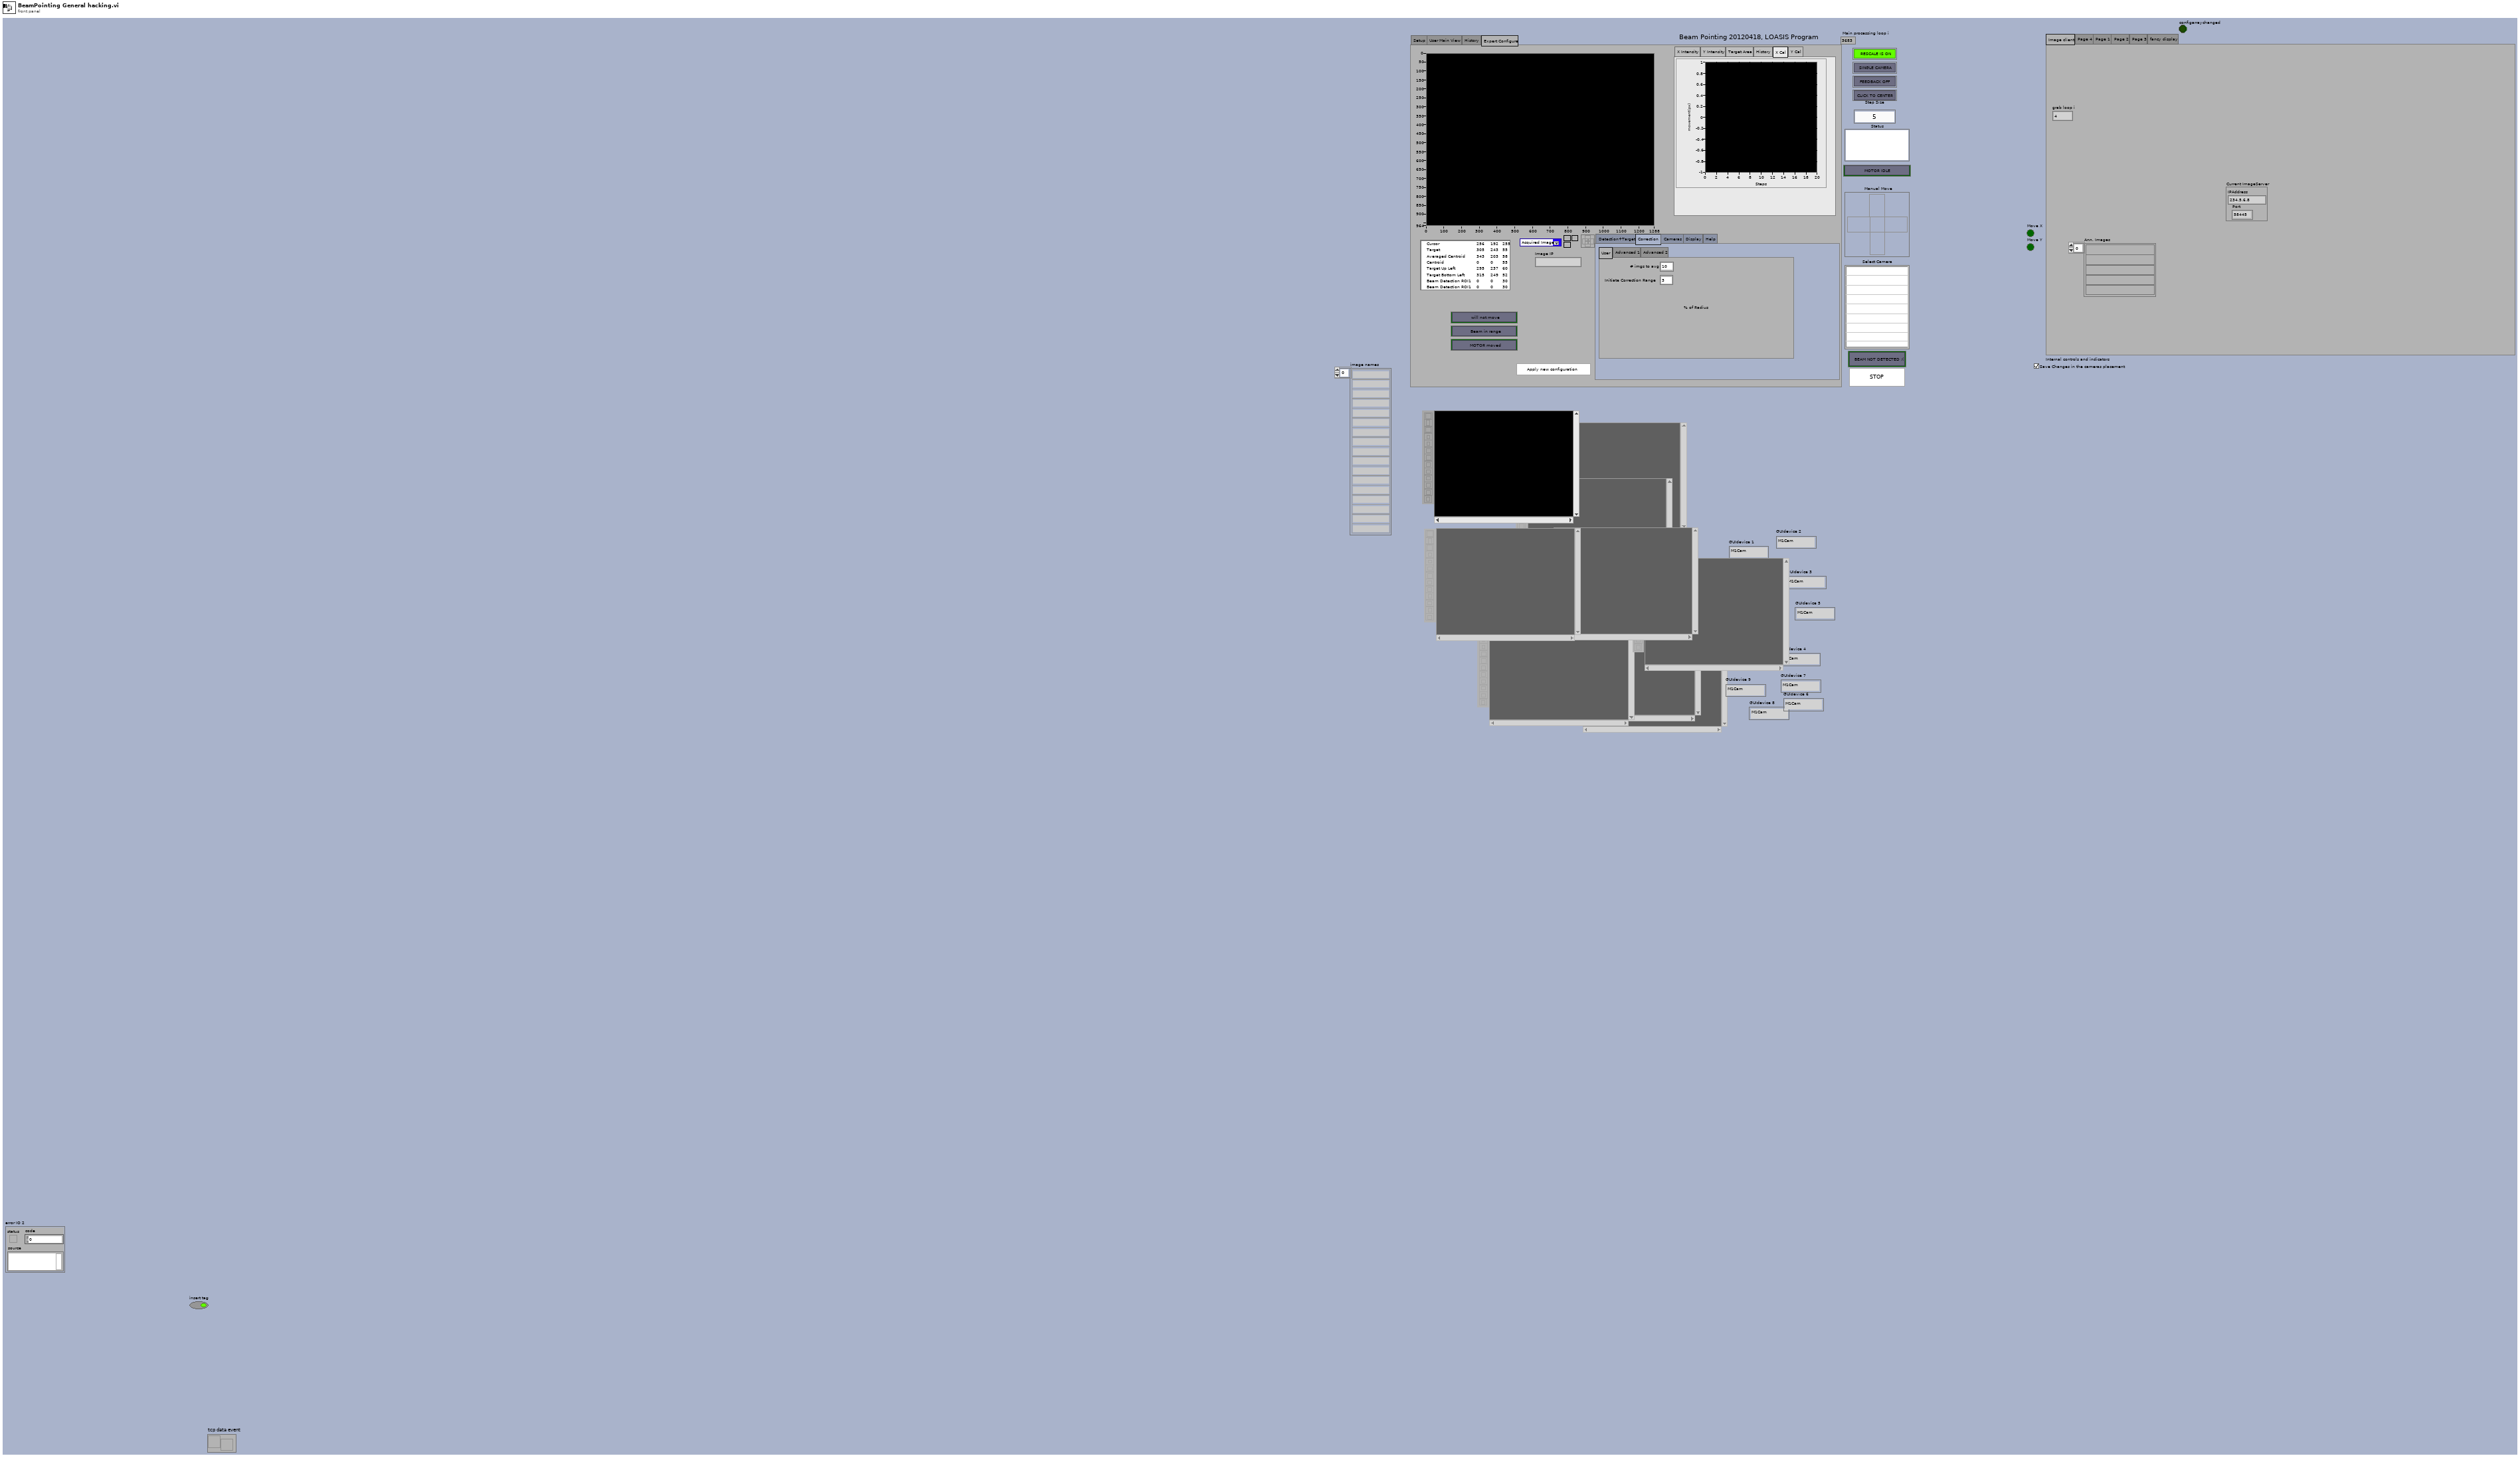
[diagram p1: front panel]
types:
  T1 = typedef "IMAQ Image.ctl" = refnum<image>
  T2 = typedef "tcp_new_data_event.ctl" = refnum<user-event>
  T3 = cluster{"Down":bool, "Up":bool, "Right":bool, "Left":bool, "APulses X":u16, "APulses Y":u16, "StopButton":bool}
  T4 = enum32{"Image client", "Page 4", "Page 1", "Page 2", "Page 3", "fancy display"}
  T5 = cluster{"Down":bool, "Up":bool, "Right":bool, "Left":bool, "APulses X":u16, "APulses Y":u16, "StopButton":bool}[]
  T6 = typedef "IMAQdx.ctl" = refnum<k21>
  T7 = cluster{"IPaddress":string, "Port":i32, "connection ID":refnum<k5>, "TCP error":errorcluster}[]
  T8 = cluster{"Add?":bool, "Channel":i32, "Device Name":string}
  T9 = cluster{"ID":dbl, "Name":string, "DeviceID":cluster{"Slot Connector":i32, "IP Adress":string, "Port":i32, "Type":string}, "CorrectConfig Cluster":cluster{"Detection Parameters":cluster{"Contrast":i32, "Treshold":u8, "Max Intensity":i32, "Max Intensity%":u8, "Rx":i32, "Ry":i32, "R%":sgl}, "Reverse":cluster{"Reverse X":bool, "Reverse Y":bool}, "Target":cluster{"X Target":sgl, "Y Target":sgl}, "Region of Interest":i32[], "Correction Parameters":cluster{"X":sgl, "Y":sgl, "Movement Type":u16}, "Acquisition Parameters":cluster{"Brightness":dbl, "Contrast":dbl, "Saturation":dbl, "White level":dbl}, "Background Path":path, "Reference Path":path, "XCalibration":cluster{dbl, dbl}[], "YCalibration":cluster{dbl, dbl}[]}, "Ontrak Channel":i16, "IMAQdx Session 2":T6, "ImageServer":cluster{"IPAddress":string, "Port":i32}}[]
  T10 = cluster{"Center":cluster{"X":sgl, "Y":sgl}, "Major Axis":cluster{"Point 1":cluster{"X":sgl, "Y":sgl}, "Point 2":cluster{"X":sgl, "Y":sgl}}, "Minor Axis":cluster{"Point 1":cluster{"X":sgl, "Y":sgl}, "Point 2":cluster{"X":sgl, "Y":sgl}}}
  T11 = cluster{"Parameter1":i32, "Parameter2":dbl, "Parameter3":dbl, "Parameter4":dbl}
  T12 = cluster{"PreviousCenter":cluster{"X":dbl, "Y":dbl}, "CurrentCenter":cluster{"X":dbl, "Y":dbl}}
  T13 = typedef "IMAQ Rectangle" = cluster{"Left":i32, "Top":i32, "Right":i32, "Bottom":i32, "Rotation":dbl}
  T14 = cluster{"seconds since 1Jan1904":timestamp, "number: 0 to 1":dbl, "number: 0 to 1":dbl}[][]
  T15 = cluster{"X Intensity":u8[], "Y Intensity":u8[], "Max Intensity":sgl, "Center":cluster{"X":sgl, "Y":sgl}, "Radius":cluster{"Rx":sgl, "Ry":sgl}}[]
  T16 = cluster{"ID":dbl, "Name":string, "DeviceID":cluster{"Slot Connector":i32, "IP Adress":string, "Port":i32, "Type":string}, "Detection Parameters":cluster{"Contrast":i32, "Treshold":u8, "Max Intensity":i32, "Max Intensity%":u8, "Rx":i32, "Ry":i32, "R%":sgl}, "Reverse":cluster{"Reverse X":bool, "Reverse Y":bool}, "Target":cluster{"X Target":sgl, "Y Target":sgl}, "Region of Interest":i32[], "Correction Parameters":cluster{"X":sgl, "Y":sgl, "Movement Type":u16}, "Acquisition Parameters":cluster{"Brightness":dbl, "Contrast":dbl, "Saturation":dbl, "White level":dbl}, "Background Path":path, "Reference Path":path, "XCalibration":cluster{dbl, dbl}[], "YCalibration":cluster{dbl, dbl}[], "ImageServer":cluster{"IPAddress":string, "Port":i32}}[]
  T17 = cluster{"seconds since 1Jan1904":timestamp, "number: 0 to 1":dbl, "number: 0 to 1":dbl}[]
  T18 = enum32{"Setup", "User Main View", "History", "Expert Configure"}
  T19 = enum32{"Detection+Target", "Correction", "Cameras", "Display", "Help"}
  T20 = cluster{"X Size":i32, "Y Size":i32, "% Tolerance":i32}
  T21 = cluster{"Contrast":i32, "Treshold":u8, "Max Intensity":i32, "Max Intensity%":u8, "Rx":i32, "Ry":i32, "R%":sgl}
  T22 = cluster{"Centroid":cluster{"X":sgl, "Y":sgl}, "Max Intensity":sgl, "Radius":cluster{"Rx":sgl, "Ry":sgl}}
  T23 = cluster{"Centroid Avg":cluster{"X":sgl, "Y":sgl}, "Max Intensity Avg":sgl, "Radius Avg":cluster{"Rx":sgl, "Ry":sgl}}
  T24 = cluster{"Use fancy display":bool, "Show Edges":bool, "Show Full Ellipse":bool, "Show Ellipses points":bool, "show acquired image":bool}
  T25 = cluster{"Show Variance":bool, "Show Target Reached":bool, "Show Init Correction":bool}
  T26 = cluster{"Show Best Rect":bool, "Show Centroid":bool, "Show Avg Centroid":bool, "Show Target":bool, "Show Target Area":bool}
  T27 = cluster{"Brightness":dbl, "Contrast":dbl, "Saturation":dbl, "White level":dbl}
  T28 = enum32{"X Intensity", "Y Intensity", "Target Area", "History", "X Cal", "Y Cal"}
  T29 = typedef "Image Type" = u32
  T30 = enum16{"open", "replace", "create", "open or create", "replace or create", "replace or create with confirmation"}
  T31 = cluster{"X Intensity":u8[], "Y Intensity":u8[], "Max Intensity":i32, "Center":cluster{"X":i32, "Y":i32}, "Radius":cluster{"Rx":i32, "Ry":i32}}
  T32 = cluster{"Slot Connector":i32, "IP Adress":string, "Port":i32, "Type":string}
  T33 = cluster{"left":i16, "top":i16, "right":i16, "bottom":i16}
  T34 = cluster{"Width":i16, "Style":enum32{"Solid", "Dash", "Dot", "DashDot", "DashDotDot"}}
  T35 = cluster{"Width":u16, "Style":enum32{"Solid", "Dash", "Dot", "DashDot", "DashDotDot"}}
  T36 = cluster{"ID":dbl, "Name":string, "DeviceID":cluster{"Slot Connector":i32, "IP Adress":string, "Port":i32, "Type":string}, "CorrectConfig Cluster":cluster{"Detection Parameters":cluster{"Contrast":i32, "Treshold":u8, "Max Intensity":i32, "Max Intensity%":u8, "Rx":i32, "Ry":i32, "R%":sgl}, "Reverse":cluster{"Reverse X":bool, "Reverse Y":bool}, "Target":cluster{"X Target":sgl, "Y Target":sgl}, "Region of Interest":i32[], "Correction Parameters":cluster{"X":sgl, "Y":sgl, "Movement Type":u16}, "Acquisition Parameters":cluster{"Brightness":dbl, "Contrast":dbl, "Saturation":dbl, "White level":dbl}, "Background Path":path, "Reference Path":path, "XCalibration":cluster{dbl, dbl}[], "YCalibration":cluster{dbl, dbl}[]}, "Ontrak Channel":i16, "IMAQdx Session 2":T6, "ImageServer":cluster{"IPAddress":string, "Port":i32}}
  T37 = cluster{"X Intensity":u8[], "Y Intensity":u8[], "Max Intensity":i32, "Center":cluster{"X":i32, "Y":i32}, "Radius":cluster{"Rx":i32, "Ry":i32}}[]
  T38 = cluster{"Down":bool, "Up":bool, "Right":bool, "Left":bool, "APulses X":i32, "APulses Y":i32, "Stop":bool}
  T39 = cluster{"Down":bool, "Up":bool, "Right":bool, "Left":bool, "APulses X":i32, "APulses Y":i32, "Stop":bool}[]
  T40 = typedef "LVPointDoubleTypeDef.ctl" = cluster{"Cursor X":dbl, "Cursor Y":dbl}
  T41 = cluster{"Show Best Rect":bool, "Show Centroid":bool}
  T42 = cluster{"X Intensity":u8[], "Y Intensity":u8[], "Max Intensity":u8, "Centroid":cluster{"X":i32, "Y":i32}, "Radius":cluster{"Rx":i32, "Ry":i32}}
  T43 = cluster{"X Intensity":u8[], "Y Intensity":u8[], "Max Intensity":sgl, "Center":cluster{"X":sgl, "Y":sgl}, "Radius":cluster{"Rx":sgl, "Ry":sgl}}
  T44 = typedef "imagedata.ctl" = cluster{"image type":i32, "image depth":i32, "image":u8[], "mask":u8[], "colors":u32[], "Rectangle":cluster{"left":i16, "top":i16, "right":i16, "bottom":i16}}
  T45 = cluster{"Left":i32, "Top":i32, "Right":i32, "Bottom":i32}
  T46 = typedef "tcp new data cluster.ctl" = cluster{"EventEnum":enum16{"new data", "connection status update"}, "Device name":string}
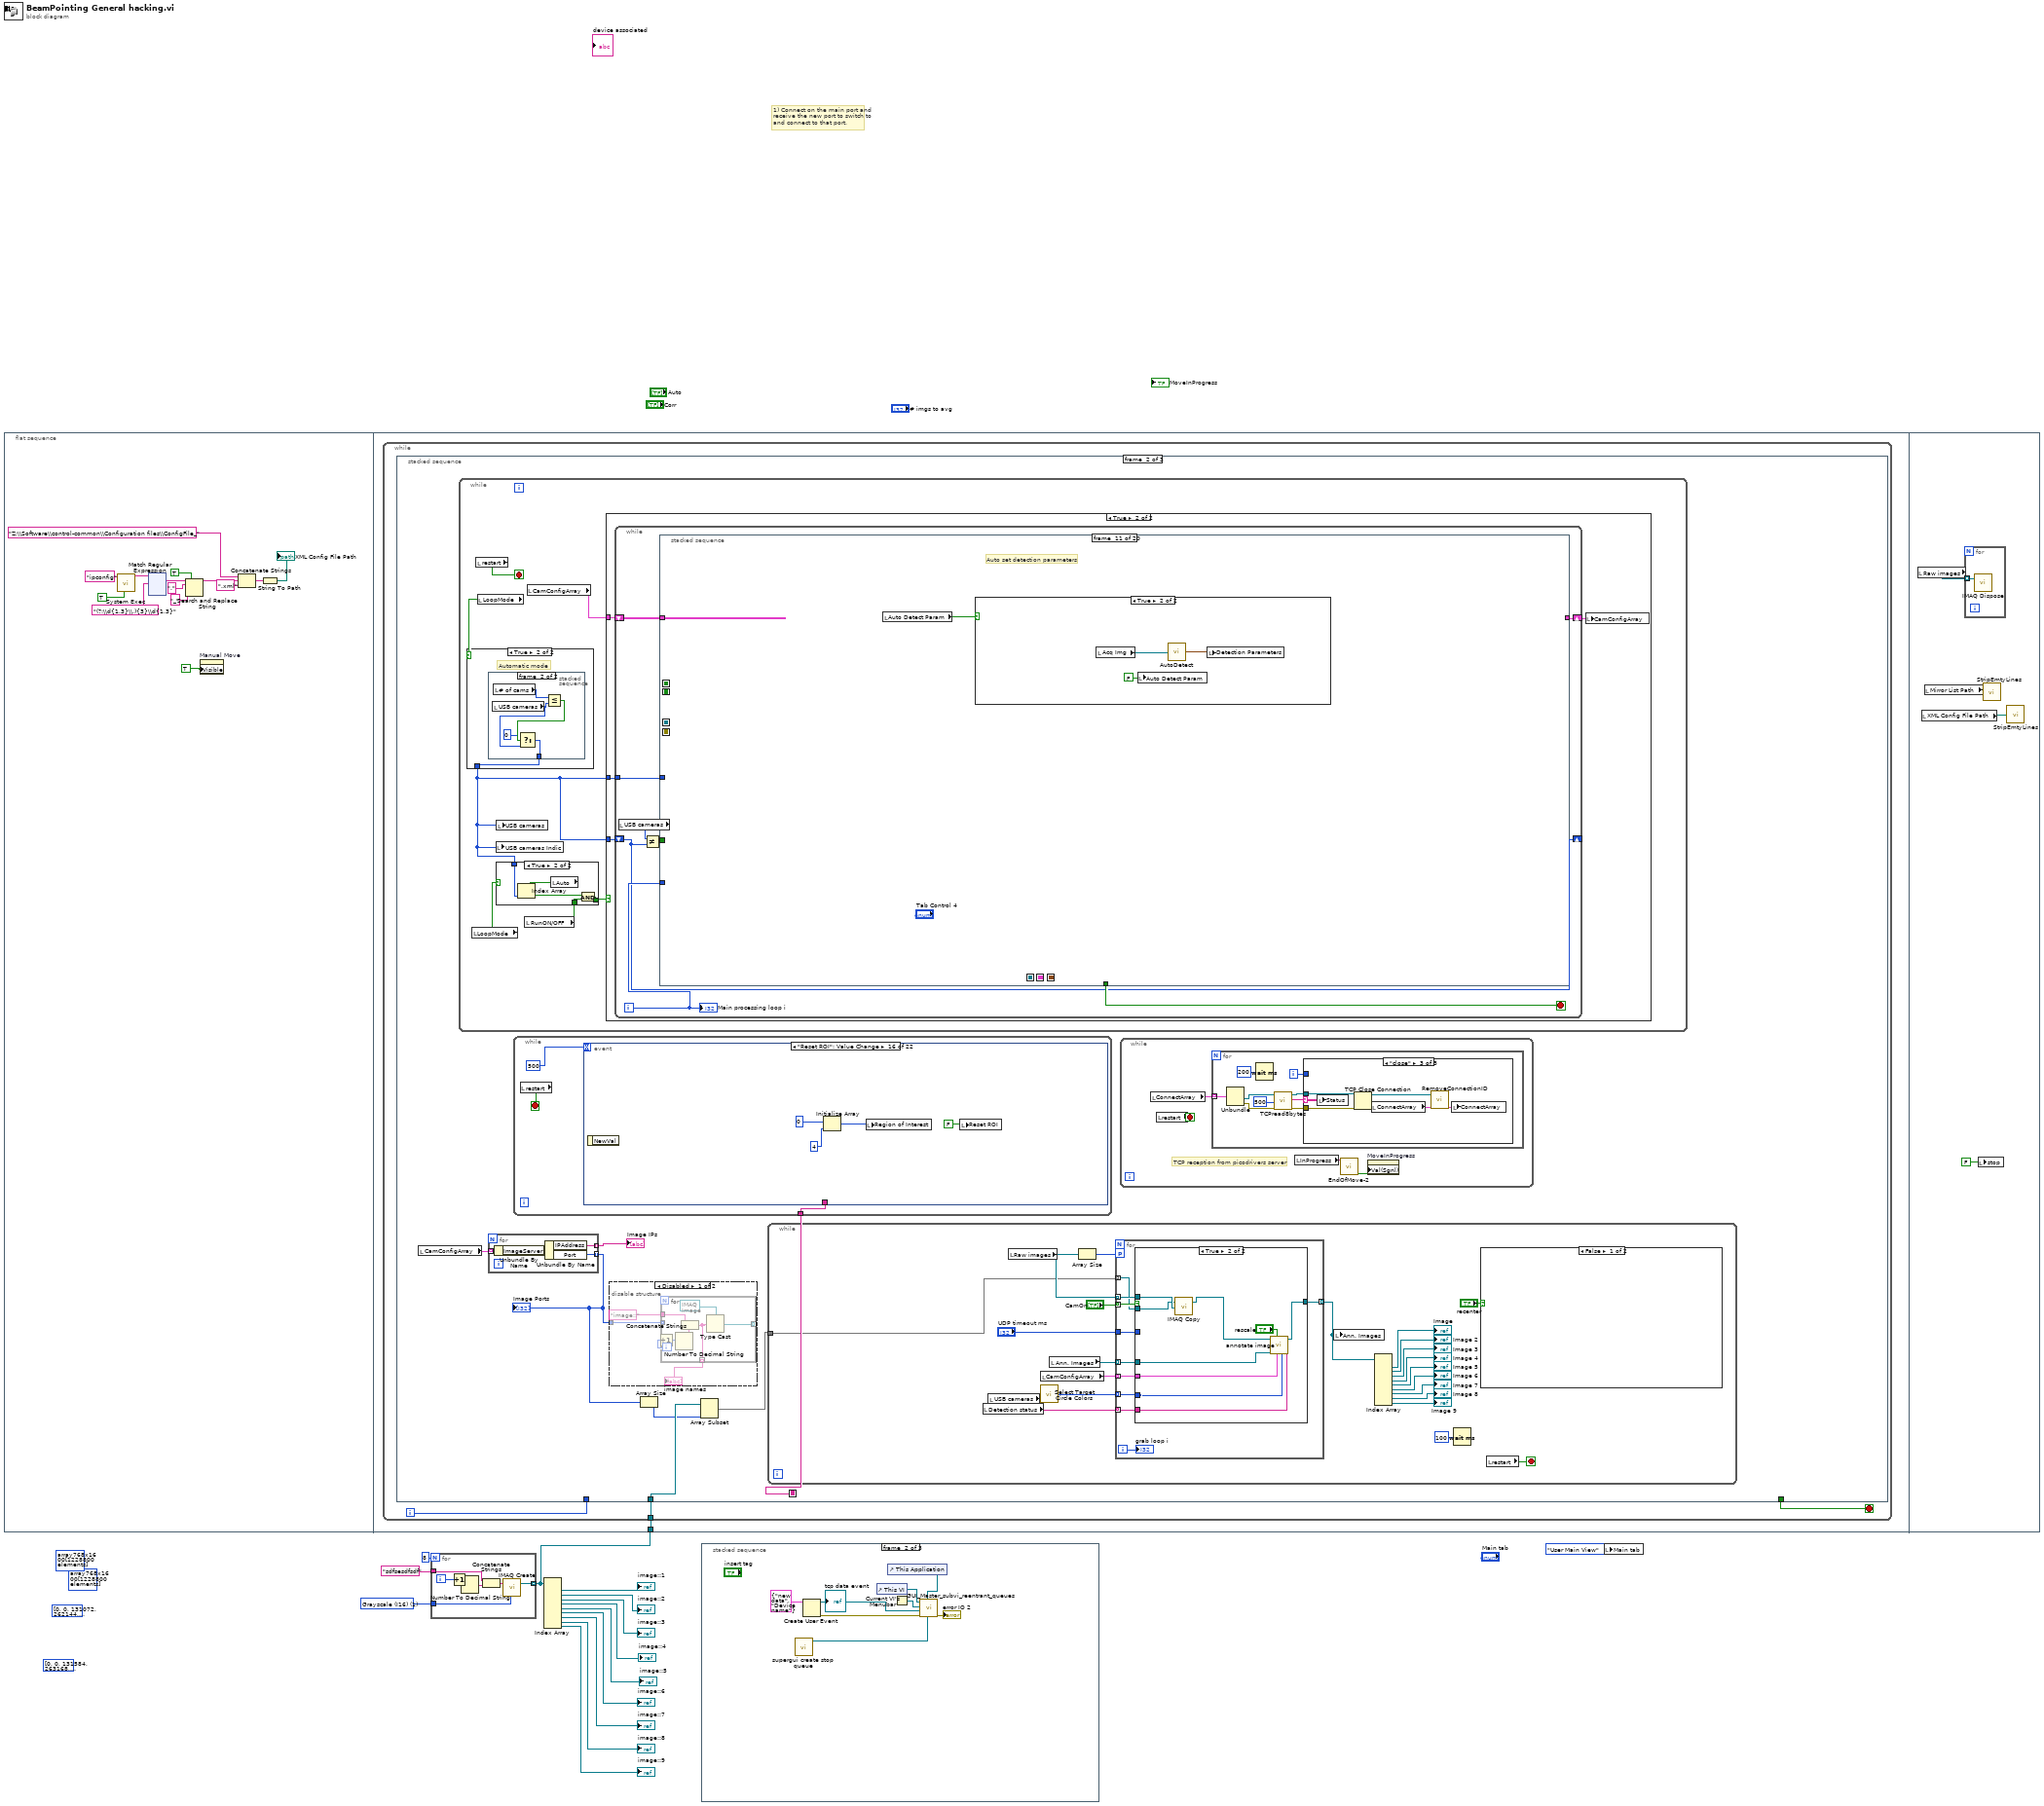
[diagram p0: block diagram]
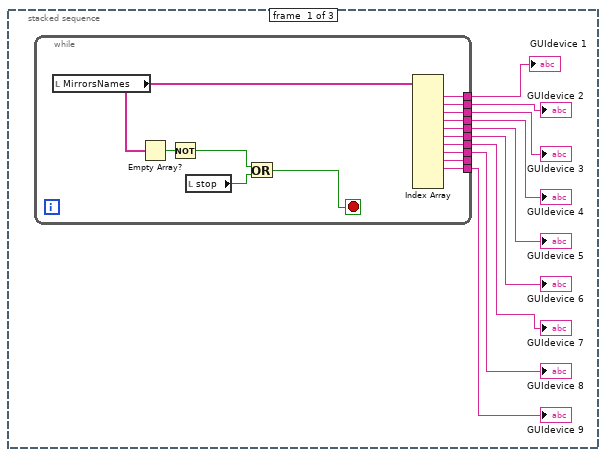
[diagram p2: hidden frame]
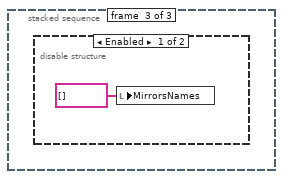
[diagram p3: hidden frame]
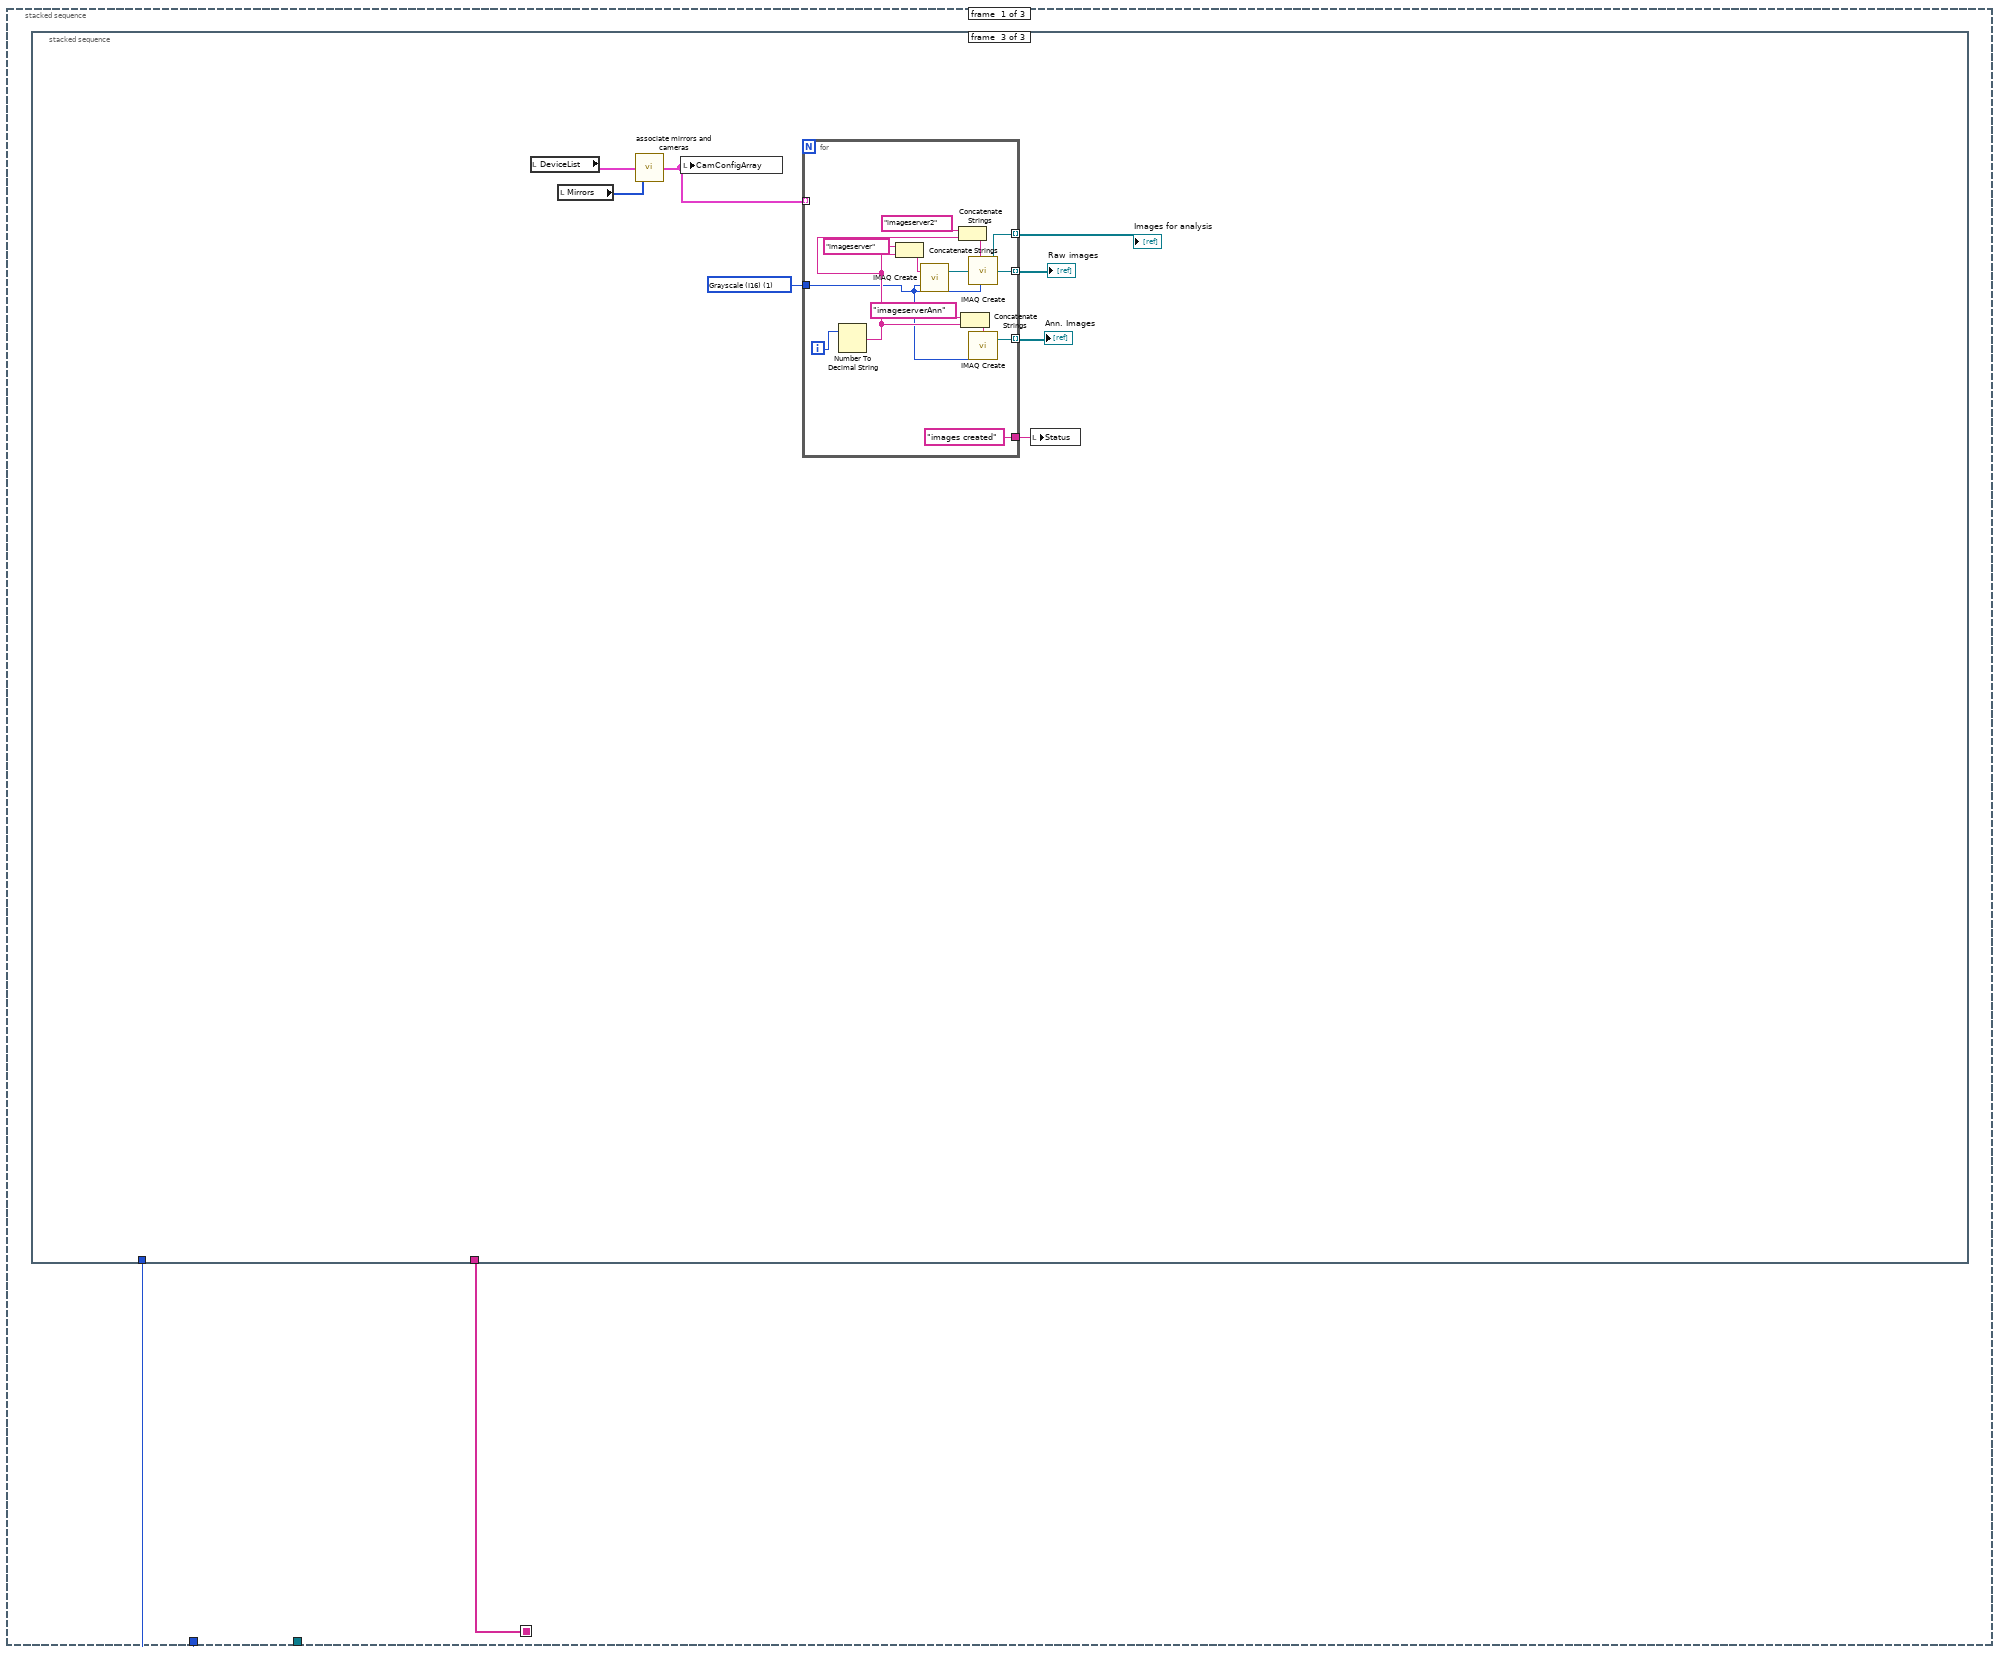
[diagram p5: hidden frame]
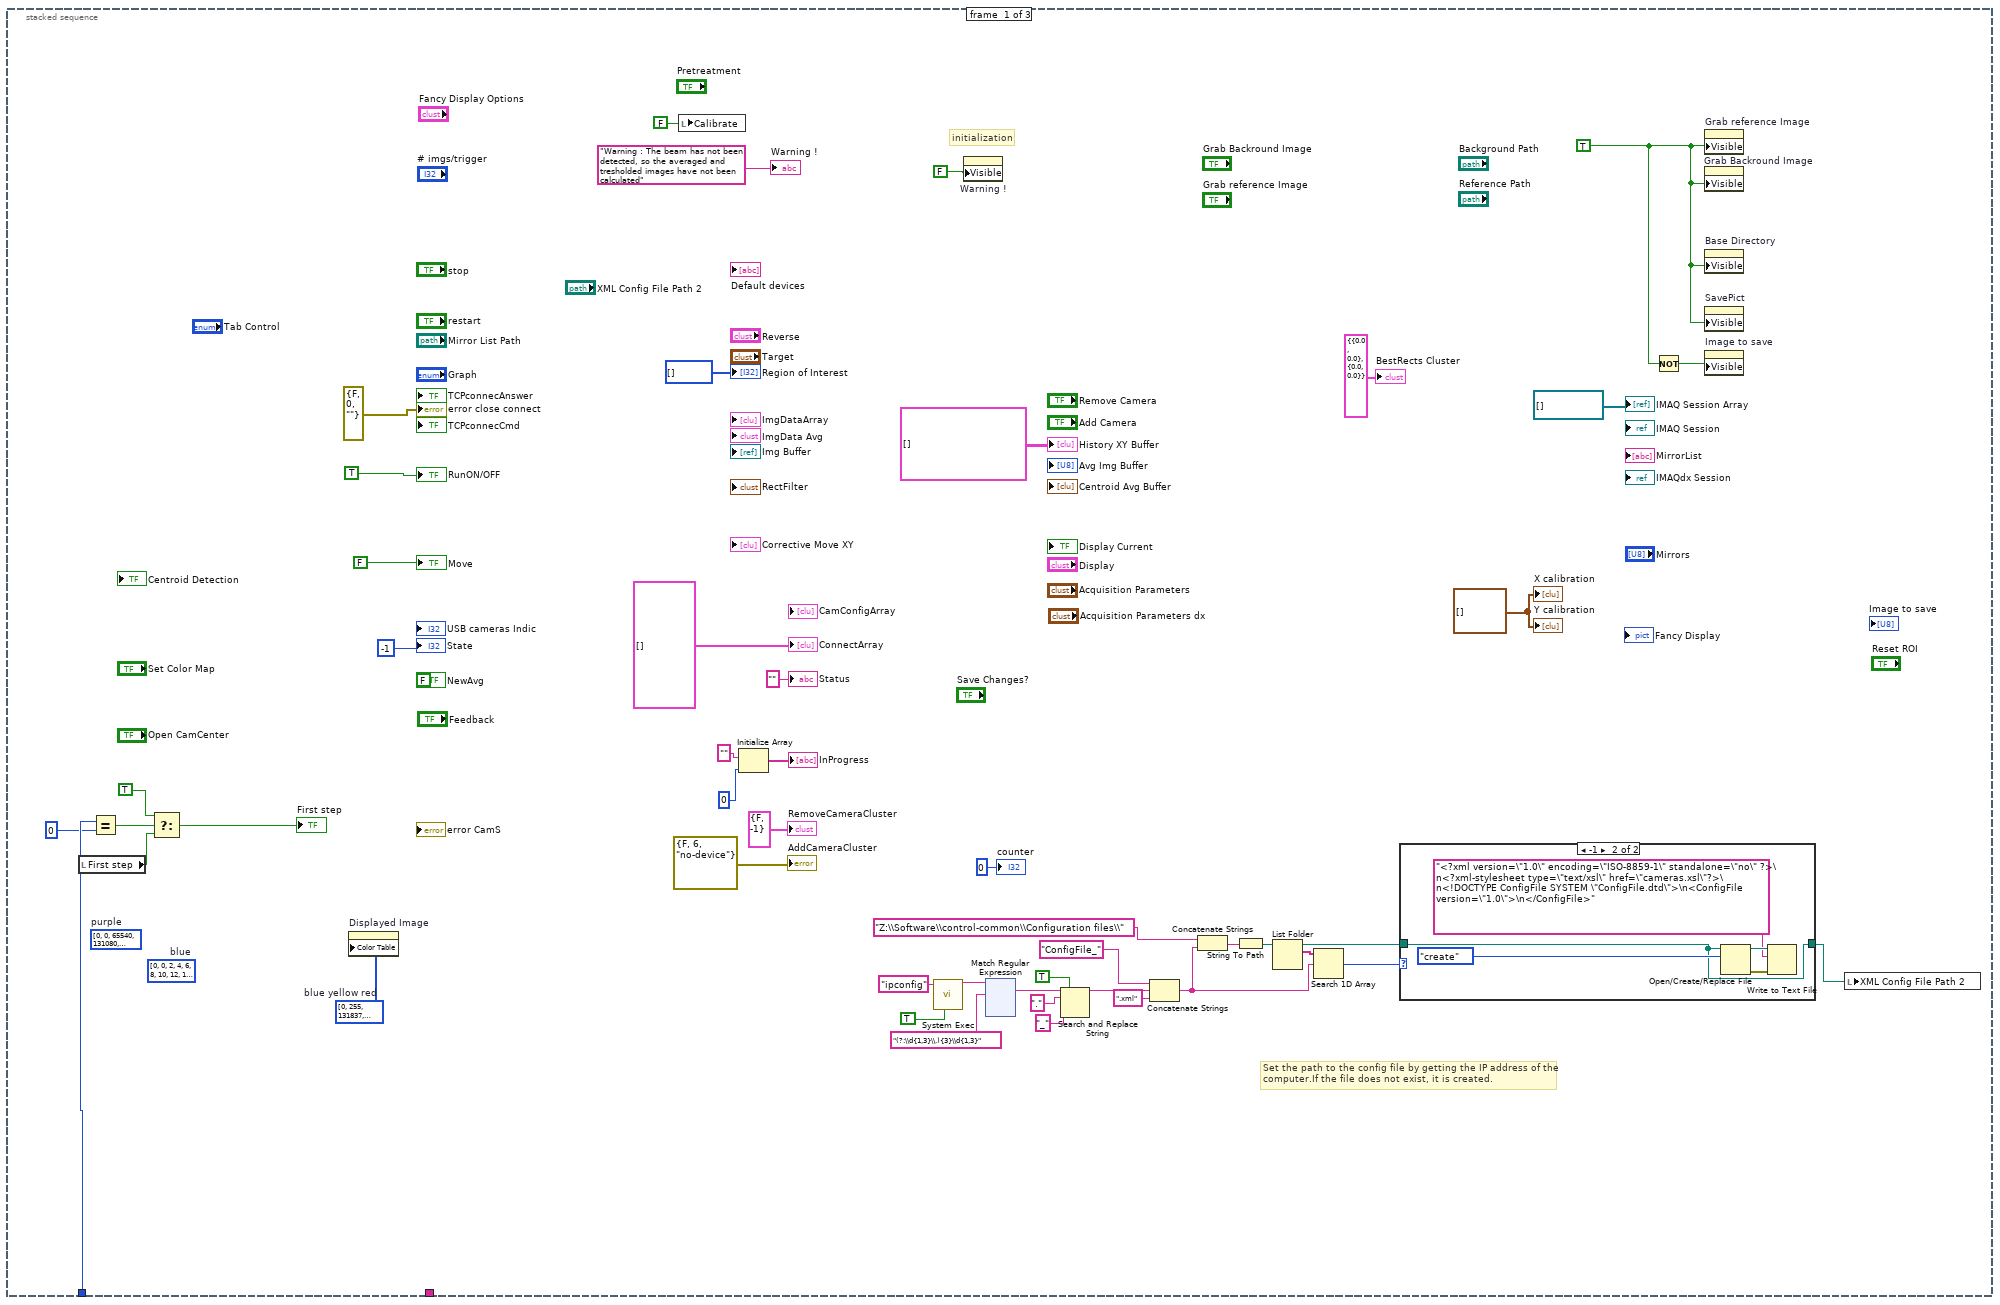
[diagram p6: hidden frame]
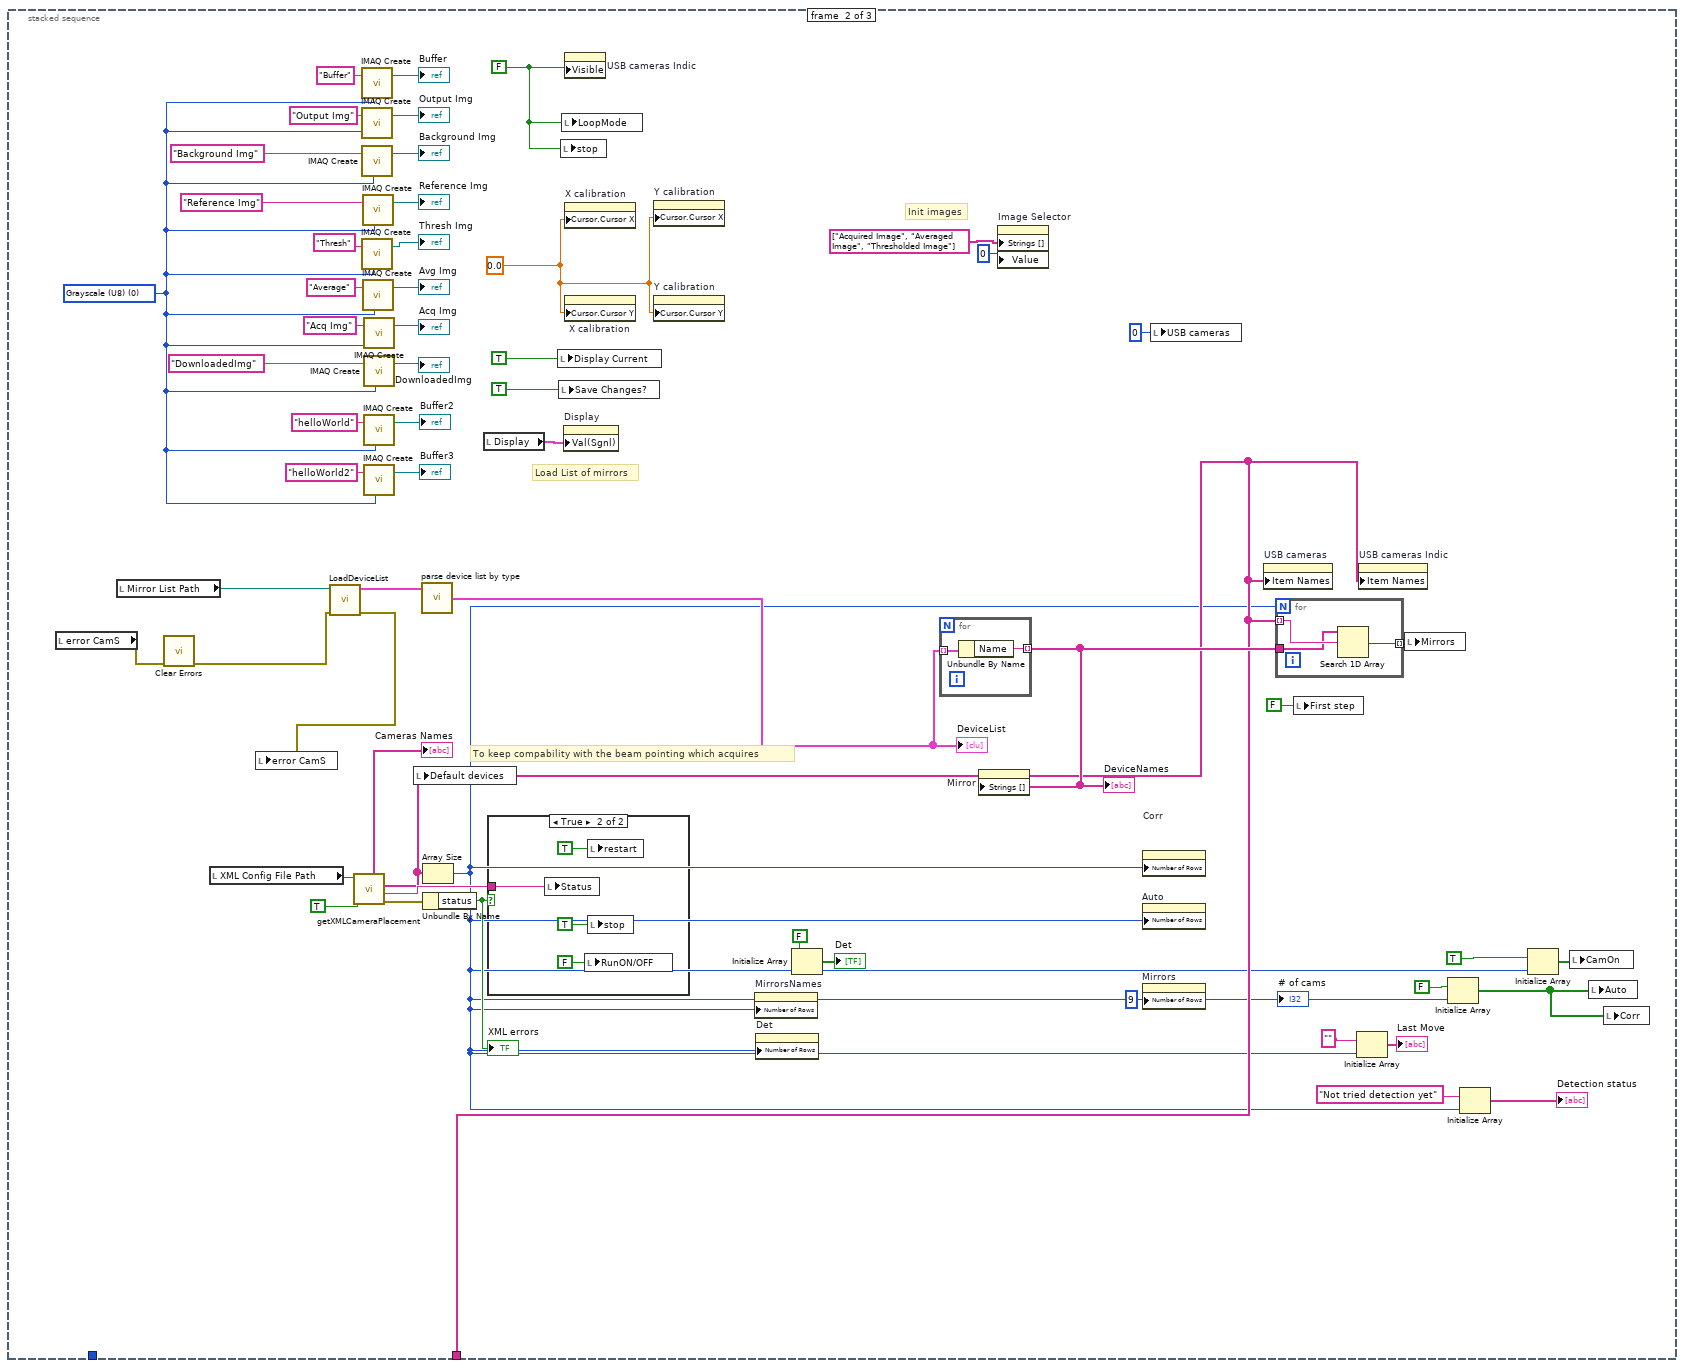
[diagram p8: hidden frame]
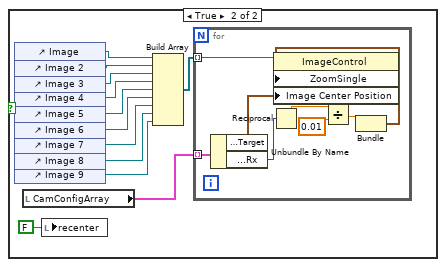
[diagram p11: hidden frame]
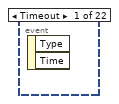
[diagram p13: hidden frame]
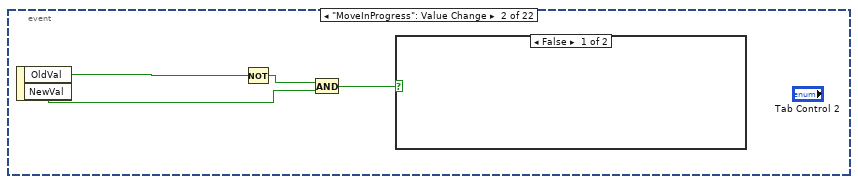
[diagram p14: hidden frame]
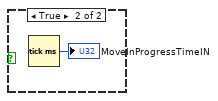
[diagram p15: hidden frame]
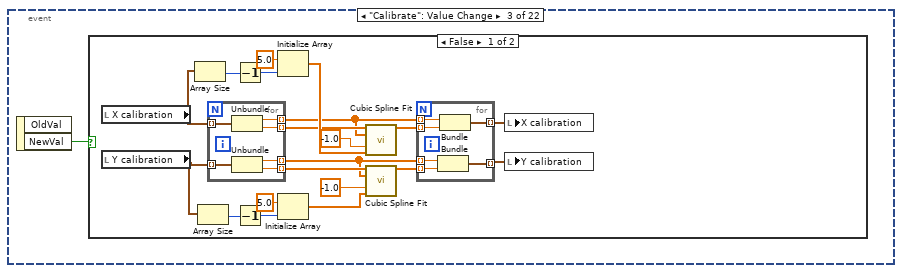
[diagram p16: hidden frame]
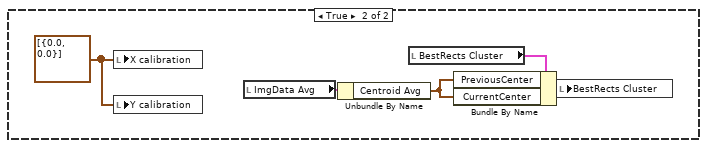
[diagram p17: hidden frame]
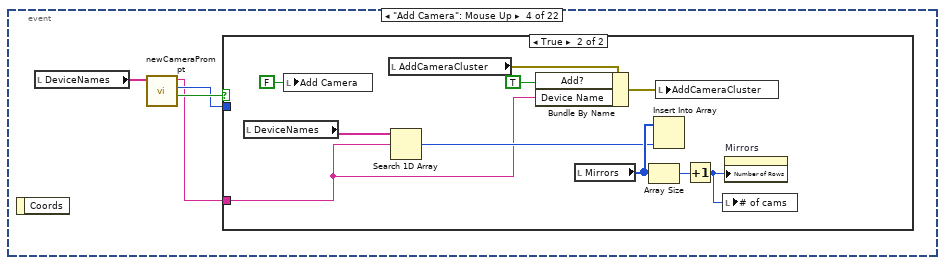
[diagram p18: hidden frame]
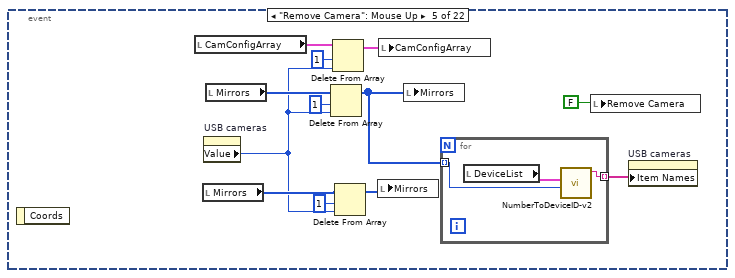
[diagram p20: hidden frame]
diagram:
  w11 = T29 1 items=["Grayscale (U8)", "Grayscale (I16)", "Grayscale (SGL)", "Complex (CSG)", "RGB (U32)", "HSL (U32)", "RGB (U64)", "Grayscale (U16)"] ("Image Type")
  (unwired) u32[] [0, 0, 131584, 263168, 394752, 592128, 723712, 855296, 986880, 1118464, 1250048, 1381632, 1579008, 1710592, 1842176, 1973760, 2105345, 2236929, 2368513, 2565889, 2697473, 2829057, 2960641, 3092225, 3223809, 3355393, 3552769, 3684353, 3815937, 3947521, 4079105, 4210689, 4342273, 4539649, 4671233, 4802817, 4934401, 5065985, 5197569, 5329153, 5526529, 5658113, 5789697, 5921281, 6052865, 6184450, 6316034, 6513410, 6644994, 6776578, 6908162, 7039746, 7171330, 7302914, 7500290, 7631874, 7763458, 7895042, 8026626, 8158210, 8289794, 8487170, 8618754, 8750338, 8881922, 9013506, 9145090, 9276674, 9474050, 9605634, 9737218, 9868802, 10000386, 10131970, 10263555, 10460931, 10592515, 10724099, 10855683, 10987267, 11118851, 11250435, 11447811, 11579395, 11710979, 11842563, 11974147, 12105731, 12237315, 12434691, 12566275, 12697859, 12829443, 12961027, 13092611, 13224195, 13421571, 13553155, 13684739, 13816323, 13947907, 14079491, 14211075, 14408452, 14540036, 14671620, 14803204, 14934788, 15066372, 15197956, 15395332, 15526916, 15658500, 15790084, 15921668, 16053252, 16184836, 16382212, 16513796, 16645380, 16776964, 16776452, 16775940, 16775428, 16775172, 16774660, 16774148, 16773636, 16773124, 16772612, 16772356, 16771844, 16771332, 16770820, 16770308, 16769796, 16769540, 16769028, 16768516, 16768004, 16767492, 16766980, 16766468, 16766212, 16765700, 16765188, 16764676, 16764164, 16763652, 16763396, 16762884, 16762372, 16761859, 16761347, 16760835, 16760323, 16760067, 16759555, 16759043, 16758531, 16758019, 16757507, 16757251, 16756739, 16756227, 16755715, 16755203, 16754691, 16754435, 16753923, 16753411, 16752899, 16752387, 16751875, 16751363, 16751107, 16750595, 16750083, 16749571, 16749059, 16748547, 16748291, 16747779, 16747267, 16746755, 16746243, 16745731, 16745475, 16744963, 16744451, 16743939, 16743427, 16742915, 16742403, 16742147, 16741635, 16741123, 16740611, 16740099, 16739587, 16739331, 16738819, 16738307, 16737795, 16737283, 16736771, 16736259, 16736003, 16735491, 16734979, 16734467, 16733955, 16733443, 16733187, 16732675, 16732163, 16731651, 16731139, 16730627, 16730371, 16729858, 16729346, 16728834, 16728322, 16727810, 16727298, 16727042, 16726530, 16726018, 16725506, 16724994, 16724482, 16724226, 16723714, 16723202, 16722690, 16722178, 16721666, 16721154, 16720898, 16720386, 16719874, 16719362, 16718850, 16718338, 16718082, 16717570, 16717058, 16716546, 16716034, 16715522, 16715266, 16714754, 16714242, 16713730, 16448250]
  (unwired) i16[][] array768x1600[1228800 elements] ("Raw image")
  (unwired) i16[][] array768x1600[1228800 elements] ("Raw image")
  (unwired) u32[] [0, 0, 131072, 262144, 393216, 589824, 720896, 851968, 983040, 1114112, 1245184, 1376256, 1572864, 1703936, 1835008, 1966080, 2097152, 2228224, 2359296, 2555904, 2686976, 2818048, 2949120, 3080192, 3211264, 3342336, 3538944, 3670016, 3801088, 3932160, 4063232, 4194304, 4325376, 4521984, 4653056, 4784128, 4915200, 5046272, 5177344, 5308416, 5505024, 5636096, 5767168, 5898240, 6029312, 6160384, 6291456, 6488064, 6619136, 6750208, 6881280, 7012352, 7143424, 7274496, 7471104, 7602176, 7733248, 7864320, 7995392, 8126464, 8257536, 8454144, 8585216, 8716288, 8847360, 8978432, 9109504, 9240576, 9437184, 9568256, 9699328, 9830400, 9961472, 10092544, 10223616, 10420224, 10551296, 10682368, 10813440, 10944512, 11075584, 11206656, 11403264, 11534336, 11665408, 11796480, 11927552, 12058624, 12189696, 12386304, 12517376, 12648448, 12779520, 12910592, 13041664, 13172736, 13369344, 13500416, 13631488, 13762560, 13893632, 14024704, 14155776, 14352384, 14483456, 14614528, 14745600, 14876672, 15007744, 15138816, 15335424, 15466496, 15597568, 15728640, 15859712, 15990784, 16121856, 16318464, 16449536, 16580608, 16711680, 16712192, 16712704, 16713216, 16713728, 16714240, 16714496, 16715008, 16715520, 16716032, 16716544, 16717056, 16717568, 16718080, 16718592, 16719104, 16719360, 16719872, 16720384, 16720896, 16721408, 16721920, 16722432, 16722944, 16723456, 16723968, 16724224, 16724736, 16725248, 16725760, 16726272, 16726784, 16727296, 16727808, 16728320, 16728832, 16729344, 16729600, 16730112, 16730624, 16731136, 16731648, 16732160, 16732672, 16733184, 16733696, 16734208, 16734464, 16734976, 16735488, 16736000, 16736512, 16737024, 16737536, 16738048, 16738560, 16739072, 16739328, 16739840, 16740352, 16740864, 16741376, 16741888, 16742400, 16742912, 16743424, 16743936, 16744448, 16744704, 16745216, 16745728, 16746240, 16746752, 16747264, 16747776, 16748288, 16748800, 16749312, 16749568, 16750080, 16750592, 16751104, 16751616, 16752128, 16752640, 16753152, 16753664, 16754176, 16754432, 16754944, 16755456, 16755968, 16756480, 16756992, 16757504, 16758016, 16758528, 16759040, 16759296, 16759808, 16760320, 16760832, 16761344, 16761856, 16762368, 16762880, 16763392, 16763904, 16764416, 16764672, 16765184, 16765696, 16766208, 16766720, 16767232, 16767744, 16768256, 16768768, 16769280, 16769536, 16770048, 16770560, 16771072, 16771584, 16772096, 16772608, 16773120, 16773632, 16774144, 16774400, 16774912, 16775424, 16775936, 16776448, 16776960, 16448250]
  # "1) Connect on the main port and receive the new port to switch to and connect to that port."
  n1 = flat-sequence {
    tunnel: w4 -> [w140]
    frame #0 {
      n2 = call <vilib>:"System Exec.vi"("run minimized? (F)"=TRUE, "command line"="ipconfig") -> ("standard output"=w26:string)  [unwired: 6 in, 3 out]
      n3 = xnode "Match Regular Expression"("input string"=w26, "regular expression"="(?:\\d{1,3}\\.){3}\\d{1,3}") -> ("whole match"=w24:string)  [unwired: 4 in, 4 out]
      n4 = Search and Replace String(replace all?=TRUE ("replace all? (F)"), input string=w24, search string=".", replace string="_" ("replace string (\"\")")) -> (result string=w20:string)  [unwired: 4 in, 3 out]
      n5 = property on="Manual Move" class="Clust"("Visible"=TRUE) -> ()  [unwired: 2 in, 2 out]
      n6 = Concatenate Strings("Z:\\Software\\control-common\\Configuration files\\ConfigFile_" ("replace string (\"\")"), w20, ".xml" ("string")) -> (w18:string)
      n7 = String To Path(string=w18) -> (path=→"XML Config File Path":path)
    }
    frame #1 {
      n8 = while {
        tunnel: w140 -> [w141]
        i -> [w142]
        stop <- w143 stop-if-true
        n9 = stacked-sequence {
          seq-local: [w145 _ _] -> [_ w405 _]
          tunnel: [_ _ w1709] -> w143
          tunnel: w142 -> [w144 _ _]
          tunnel: w141 -> [_ w401 _]
          frame #0 {
            n10 = stacked-sequence {
              tunnel: [_ w329 _] -> w145
              tunnel: w144 -> [w181 _ _]
              frame #0 {
                w146 = u32[] [0, 255, 131837, 263419, 395001, 526583, 658165, 789747, 921329, 1052911, 1184493, 1316075, 1447657, 1579239, 1710820, 1842402, 1973984, 2105566, 2237148, 2368730, 2500312, 2631894, 2828756, 2960338, 3091920, 3223502, 3355084, 3486666, 3618248, 3749830, 3881412, 4012994, 4144576, 4276158, 4407740, 4539322, 4670904, 4802486, 4934068, 5065649, 5197231, 5328813, 5460395, 5591977, 5723559, 5855141, 5986723, 6118305, 6249887, 6381469, 6513051, 6644633, 6776215, 6907797, 7039379, 7170961, 7302543, 7434125, 7565707, 7697289, 7828871, 7960453, 8092035, 8223617, 8355198, 8552060, 8683642, 8815224, 8946806, 9078388, 9209970, 9341552, 9473134, 9604716, 9736298, 9867880, 9999462, 10131044, 10262626, 10394208, 10525790, 10657372, 10788954, 10920536, 11052118, 11183700, 11315282, 11446864, 11578445, 11710027, 11841609, 11973191, 12104773, 12236355, 12367937, 12499519, 12631101, 12762683, 12894265, 13025847, 13157429, 13289011, 13420593, 13552175, 13683757, 13815339, 13946921, 14143783, 14275365, 14406947, 14538529, 14670111, 14801693, 14933274, 15064856, 15196438, 15328020, 15459602, 15591184, 15722766, 15854348, 15985930, 16117512, 16249094, 16380676, 16512258, 16643842, 16775426, 16774914, 16774402, 16773890, 16773378, 16772866, 16772354, 16771842, 16771330, 16770818, 16770306, 16769794, 16769282, 16769026, 16768514, 16768002, 16767490, 16766978, 16766466, 16765954, 16765442, 16764930, 16764418, 16763906, 16763394, 16762882, 16762370, 16761858, 16761346, 16760834, 16760322, 16759809, 16759297, 16758785, 16758273, 16757761, 16757249, 16756737, 16756225, 16755969, 16755457, 16754945, 16754433, 16753921, 16753409, 16752897, 16752385, 16751873, 16751361, 16750849, 16750337, 16749825, 16749313, 16748801, 16748289, 16747777, 16747265, 16746753, 16746241, 16745729, 16745217, 16744705, 16744193, 16743681, 16743425, 16742913, 16742401, 16741889, 16741377, 16740865, 16740353, 16739841, 16739329, 16738817, 16738305, 16737793, 16737281, 16736769, 16736257, 16735745, 16735233, 16734721, 16734209, 16733697, 16733185, 16732673, 16732161, 16731649, 16731137, 16730881, 16730369, 16729857, 16729345, 16728833, 16728321, 16727808, 16727296, 16726784, 16726272, 16725760, 16725248, 16724736, 16724224, 16723712, 16723200, 16722688, 16722176, 16721664, 16721152, 16720640, 16720128, 16719616, 16719104, 16718592, 16718080, 16717824, 16717312, 16716800, 16716288, 16715776, 16715264, 16714752, 16714240, 16713728, 16713216, 16712704, 16712192, 16711680, 16711680]  # blue yellow red
                (unwired) u32[] [0, 0, 65540, 131080, 196620, 262160, 327700, 393240, 458780, 524320, 589860, 589864, 655404, 720944, 786484, 852024, 917564, 983104, 1048644, 1114184, 1179724, 1245264, 1310804, 1376344, 1441884, 1507424, 1572964, 1638504, 1704044, 1704048, 1769588, 1835128, 1900668, 1966208, 2031747, 2097287, 2162827, 2228367, 2293907, 2359447, 2424987, 2490527, 2556067, 2621607, 2687147, 2752687, 2818227, 2883767, 2883771, 2949311, 3014851, 3080391, 3145931, 3211471, 3277011, 3342551, 3408091, 3473631, 3539171, 3604711, 3670251, 3735791, 3801331, 3866871, 3932411, 3997951, 3997951, 4063487, 4129023, 4194559, 4260095, 4325631, 4391167, 4456703, 4522239, 4587775, 4653311, 4718847, 4784383, 4849919, 4915455, 4980991, 5046527, 5112063, 5112063, 5177599, 5243135, 5308671, 5374207, 5439743, 5505279, 5570815, 5636351, 5701887, 5767423, 5832959, 5898495, 5964031, 6029567, 6095103, 6160639, 6226175, 6291711, 6291711, 6357247, 6422783, 6488319, 6553855, 6619391, 6684927, 6750463, 6815999, 6881535, 6947071, 7012607, 7078143, 7143679, 7209215, 7274751, 7340287, 7405823, 7405823, 7471359, 7536895, 7602431, 7667967, 7733503, 7799039, 7864575, 7930111, 7995647, 8061183, 8126719, 8192255, 8257791, 8323327, 8388863, 8519935, 8585471, 8651007, 8716543, 8782079, 8847615, 8913151, 8978687, 9044223, 9109759, 9175295, 9240831, 9306367, 9371903, 9502975, 9568511, 9634047, 9699583, 9765119, 9830655, 9896191, 9961727, 10027263, 10092799, 10158335, 10223871, 10289407, 10354943, 10486015, 10551551, 10617087, 10682623, 10748159, 10813695, 10879231, 10944767, 11010303, 11075839, 11141375, 11206911, 11272447, 11337983, 11469055, 11534591, 11600895, 11667455, 11733759, 11800319, 11866623, 11933183, 11999487, 12066047, 12132351, 12198655, 12265215, 12331519, 12463615, 12529919, 12596479, 12662783, 12729343, 12795647, 12861951, 12928511, 12994815, 13061375, 13127679, 13194239, 13260543, 13392639, 13458943, 13525247, 13591807, 13658111, 13724671, 13790975, 13857535, 13923839, 13990399, 14056703, 14123263, 14189567, 14255871, 14387967, 14454271, 14520831, 14587135, 14653695, 14719999, 14786559, 14852863, 14919167, 14985727, 15052031, 15118591, 15184895, 15251455, 15383295, 15449855, 15516159, 15582463, 15649023, 15715327, 15781887, 15848191, 15914751, 15981055, 16047615, 16113919, 16180223, 16246783, 16378623, 16445183, 16511487, 16578047, 16644351, 16710911, 16777215, 16448250]  # purple
                (unwired) u32[] [0, 0, 2, 4, 6, 8, 10, 12, 14, 16, 18, 20, 22, 24, 26, 28, 30, 32, 34, 36, 38, 40, 42, 44, 46, 48, 50, 52, 54, 56, 58, 60, 62, 64, 66, 68, 70, 72, 74, 76, 78, 80, 82, 84, 86, 88, 90, 92, 94, 96, 98, 100, 102, 104, 106, 108, 110, 112, 114, 116, 118, 120, 122, 124, 126, 128, 130, 132, 134, 136, 138, 140, 142, 144, 146, 148, 150, 152, 154, 156, 158, 160, 162, 164, 166, 168, 170, 172, 174, 176, 178, 180, 182, 184, 186, 188, 190, 192, 194, 196, 198, 200, 202, 204, 206, 208, 210, 212, 214, 216, 218, 220, 222, 224, 226, 228, 230, 232, 234, 236, 238, 240, 242, 244, 246, 248, 250, 252, 255, 131839, 263423, 395007, 526591, 658175, 789759, 921343, 1052927, 1184511, 1316095, 1447679, 1579263, 1710847, 1842431, 1974015, 2105599, 2237183, 2368767, 2500351, 2631935, 2763519, 2895103, 3026687, 3158271, 3289855, 3421439, 3553023, 3684607, 3816191, 3947775, 4079359, 4210943, 4342527, 4474111, 4605695, 4737279, 4868863, 5000447, 5132031, 5263615, 5395199, 5526783, 5658367, 5789951, 5921535, 6053119, 6184703, 6316287, 6447871, 6579455, 6711039, 6842623, 6974207, 7105791, 7237375, 7368959, 7500543, 7632127, 7763711, 7895295, 8026879, 8158463, 8290047, 8421631, 8553215, 8684799, 8816383, 8947967, 9079551, 9211135, 9342719, 9474303, 9605887, 9737471, 9869055, 10000639, 10132223, 10263807, 10395391, 10526975, 10658559, 10790143, 10921727, 11053311, 11184895, 11316479, 11448063, 11579647, 11711231, 11842815, 11974399, 12105983, 12237567, 12369151, 12500735, 12632319, 12763903, 12895487, 13027071, 13158655, 13290239, 13421823, 13553407, 13684991, 13816575, 13948159, 14079743, 14211327, 14342911, 14474495, 14606079, 14737663, 14869247, 15000831, 15132415, 15263999, 15395583, 15527167, 15658751, 15790335, 15921919, 16053503, 16185087, 16316671, 16448255, 16579839, 16777215]  # blue
                w167 = cluster{dbl, dbl}[] [] ("XY Graph")
                w170 = TRUE ("Visible")
                # "Set the path to the config file by getting the IP address of the computer.If the file does not exist, it is created."
                # "initialization"
                n11 = local read "First step"() -> (w177:bool)
                n12 = Equal?(x=w181, y=0) -> (x = y?=w179:bool)
                n13 = Select(t=TRUE, s=w179, f=w177) -> (s? t:f=→"First step":bool)
                n14 = property on="Displayed Image" class="IntGraph (strict)"("Color Table"=w146) -> ()  [unwired: 2 in, 2 out]
                n15 = local write "Calibrate"(FALSE ("Calibrate")) -> ()
                n16 = Initialize Array("", 0 ("dimension size")) -> (→"InProgress":string[])
                n17 = call <vilib>:"System Exec.vi"("run minimized? (F)"=TRUE, "command line"="ipconfig") -> ("standard output"=w163:string)  [unwired: 6 in, 3 out]
                n18 = property on="Warning !" class="Str"("Visible"=FALSE) -> ()  [unwired: 2 in, 2 out]
                n19 = xnode "Match Regular Expression"("input string"=w163, "regular expression"="(?:\\d{1,3}\\.){3}\\d{1,3}") -> ("whole match"=w161:string)  [unwired: 4 in, 4 out]
                n20 = Search and Replace String(replace all?=TRUE ("replace all? (F)"), input string=w161, search string=".", replace string="_" ("replace string (\"\")")) -> (result string=w157:string)  [unwired: 4 in, 3 out]
                n21 = Concatenate Strings("ConfigFile_" ("replace string (\"\")"), w157, ".xml" ("string")) -> (w150:string)
                n22 = Concatenate Strings("Z:\\Software\\control-common\\Configuration files\\" ("replace string (\"\")"), w150) -> (w151:string)
                n23 = String To Path(string=w151) -> (path=w154:path)
                n24 = List Folder(path=w154) -> (path out=w148:path, filenames=w153:string[])  [unwired: 3 in, 2 out]
                n25 = Search 1D Array(1D array=w153, element=w150) -> (index of element=w149:i32)  [unwired: 1 in]
                n26 = case shown="-1" w149 {
                  tunnel: w148 -> [w195 w199]
                  tunnel: [w195 w199] -> w147
                  frame 0, Default {
                  }
                  frame -1 {
                    n27 = Open/Create/Replace File(file path (use dialog)=w199, operation (0:open)=T30."create") -> (refnum out=w197:refnum<file>, error out=w198:errorcluster)  [unwired: 4 in, 1 out]
                    n28 = Write to Text File(file (use dialog)=w197, text="<?xml version=\"1.0\" encoding=\"ISO-8859-1\" standalone=\"no\" ?>\n<?xml-stylesheet type=\"text/xsl\" href=\"cameras.xsl\"?>\n<!DOCTYPE ConfigFile SYSTEM \"ConfigFile.dtd\">\n<ConfigFile version=\"1.0\">\n</ConfigFile>", error in=w198) -> ()  [unwired: 1 in, 3 out]
                  }
                }
                n29 = Not(x=w170) -> (.not. x?=w169:bool)
                n30 = property on="Grab reference Image" class="Bool (strict)"("Visible"=w170) -> ()  [unwired: 2 in, 2 out]
                n31 = property on="Grab Backround Image" class="Bool (strict)"("Visible"=w170) -> ()  [unwired: 2 in, 2 out]
                n32 = property on="Base Directory" class="Path"("Visible"=w170) -> ()  [unwired: 2 in, 2 out]
                n33 = property on="SavePict" class="Bool (strict)"("Visible"=w170) -> ()  [unwired: 2 in, 2 out]
                n34 = property on="Image to save" class="IntGraph (strict)"("Visible"=w169) -> ()  [unwired: 2 in, 2 out]
                n35 = local write "XML Config File Path 2"(w147) -> ()
                "Status" <- "" ("status")
                "ConnectArray" <- T7 [] ("ConnectArray")
                "RunON/OFF" <- TRUE ("RunON/OFF")
                "State" <- -1 ("State")
                "error close connect" <- errorcluster {"status"=FALSE, "code"=0, "source"=""} ("error close connect")
                "Move" <- FALSE ("Feedback")
                "NewAvg" <- FALSE ("Feedback")
                "Region of Interest" <- i32[] []
                "History XY Buffer" <- T14 [] ("History XY Buffer")
                "IMAQ Session Array" <- refnum<k11>[] [] ("IMAQ Session Array")
                "Warning !" <- "Warning : The beam has not been detected, so the averaged and tresholded images have not been calculated" ("Warning !")
                "counter" <- 0 ("counter")
                "RemoveCameraCluster" <- cluster{"Remove?":bool, "number":i32} {"Remove?"=FALSE, "number"=-1} ("RemoveCamera")
                "AddCameraCluster" <- T8 {"Add?"=FALSE, "Channel"=6, "Device Name"="no-device"} ("AddCameraCluster")
                "BestRects Cluster" <- T12 {"PreviousCenter"={"X"=0.0, "Y"=0.0}, "CurrentCenter"={"X"=0.0, "Y"=0.0}} ("BestRects Cluster")
                "X calibration" <- w167
                "Y calibration" <- w167
              }
              frame #1 {
                w349 = 0.0 ("Cursor.Cursor Position:Cursor X")
                w313 = T29 0 items=["Grayscale (U8)", "Grayscale (I16)", "Grayscale (SGL)", "Complex (CSG)", "RGB (U32)", "HSL (U32)", "RGB (U64)"] ("Image Type")
                w363 = FALSE ("Enable Feedback")
                # "To keep compability with the beam pointing which acquires"
                # "Load List of mirrors"
                # "Init images"
                n36 = local read "error CamS"() -> (w335:errorcluster)
                n37 = local read "Mirror List Path"() -> (w348:path)
                n38 = call <vilib>:"Clear Errors.vi"("error in (no error)"=w335) -> ("error out"=w334:errorcluster)  [unwired: 6 in]
                n39 = local read "XML Config File Path"() -> (w339:path)
                n40 = call "LoadDeviceList.vi"("error in"=w334, "path to XML document"=w348) -> ("error out"=w347:errorcluster, "DeviceList"=w346:T16)  [unwired: 7 in, 1 out]
                n41 = local write "error CamS"(w347) -> ()
                n42 = call "getXMLCameraPlacement.vi"("usb/watec"=TRUE, "path to XML document"=w339) -> ("error out"=w340:errorcluster, "parse errors"=w341:string, "Default devices"=w329:string[], "Default Cameras Names"=→"Cameras Names":string[])  [unwired: 5 in, 1 out]
                n43 = call "IMAQ Create"("Image Name"="Buffer", "Image Type"=w313) -> ("New Image"=→"Buffer":T1)  [unwired: 2 in, 2 out]
                n44 = call "IMAQ Create"("Image Name"="Output Img", "Image Type"=w313) -> ("New Image"=→"Output Img":T1)  [unwired: 2 in, 2 out]
                n45 = call "IMAQ Create"("Image Name"="Background Img", "Image Type"=w313) -> ("New Image"=→"Background Img":T1)  [unwired: 2 in, 2 out]
                n46 = call "IMAQ Create"("Image Name"="Thresh", "Image Type"=w313) -> ("New Image"=→"Thresh Img":T1)  [unwired: 2 in, 2 out]
                n47 = call "IMAQ Create"("Image Name"="Reference Img", "Image Type"=w313) -> ("New Image"=→"Reference Img":T1)  [unwired: 2 in, 2 out]
                n48 = call "IMAQ Create"("Image Name"="Average", "Image Type"=w313) -> ("New Image"=→"Avg Img":T1)  [unwired: 2 in, 2 out]
                n49 = call "IMAQ Create"("Image Name"="Acq Img", "Image Type"=w313) -> ("New Image"=→"Acq Img":T1)  [unwired: 2 in, 2 out]
                n50 = call "IMAQ Create"("Image Name"="DownloadedImg", "Image Type"=w313) -> ("New Image"=→"DownloadedImg":T1)  [unwired: 2 in, 2 out]
                n51 = call "IMAQ Create"("Image Name"="helloWorld", "Image Type"=w313) -> ("New Image"=→"Buffer2":T1)  [unwired: 2 in, 2 out]
                n52 = call "IMAQ Create"("Image Name"="helloWorld2", "Image Type"=w313) -> ("New Image"=→"Buffer3":T1)  [unwired: 2 in, 2 out]
                n53 = local write "Default devices"(w329) -> ()
                n54 = call "parse device list by type.vi"("DeviceListin"=w346) -> ("DeviceListout"=w345:T16)  [unwired: 1 in]
                "DeviceList" <- w345
                n55 = Array Size(array=w329) -> (size(s)=w317:i32)
                "# of cams" <- w317
                n56 = Unbundle By Name(w340) -> ("status"=w342:bool)
                "XML errors" <- w342
                n57 = local read "Display"() -> (w360:T26)
                n58 = case shown="True" w342 {
                  tunnel: w341 -> [_ w375]
                  frame False {
                  }
                  frame True {
                    n59 = local write "Status"(w375) -> ()
                    n60 = local write "RunON/OFF"(FALSE ("restart")) -> ()
                    n61 = local write "restart"(TRUE ("restart")) -> ()
                    n62 = local write "stop"(TRUE ("restart")) -> ()
                  }
                }
                n63 = local write "Display Current"(TRUE ("Display Current")) -> ()
                n64 = local write "Save Changes?"(TRUE ("Save Changes")) -> ()
                n65 = local write "stop"(w363) -> ()
                n66 = local write "LoopMode"(w363) -> ()
                n67 = property on="Display" class="Clust (strict)"("Val(Sgnl)"=w360) -> ()  [unwired: 2 in, 2 out]
                n68 = property on="USB cameras Indic" class="LstBox (strict)"("Visible"=w363) -> ()  [unwired: 2 in, 2 out]
                n69 = property on="X calibration" class="XYGraph (strict)"("Cursor.Cursor X"=w349) -> ()  [unwired: 2 in, 2 out]
                n70 = property on="X calibration" class="XYGraph (strict)"("Cursor.Cursor Y"=w349) -> ()  [unwired: 2 in, 2 out]
                n71 = property on="Y calibration" class="XYGraph (strict)"("Cursor.Cursor X"=w349) -> ()  [unwired: 2 in, 2 out]
                n72 = property on="Y calibration" class="XYGraph (strict)"("Cursor.Cursor Y"=w349) -> ()  [unwired: 2 in, 2 out]
                n73 = property on="MirrorsNames" class="Arr (strict)"("Number of Rows"=w317) -> ()  [unwired: 2 in, 2 out]
                n74 = property on="Det" class="Arr (strict)"("Number of Rows"=w317) -> ()  [unwired: 2 in, 2 out]
                n75 = Initialize Array(FALSE, w317) -> (→"Det":bool[])
                n76 = for {
                  tunnel: w345 -> [w377] mode=indexing
                  tunnel: [w376] -> w344 mode=indexing
                  n77 = Unbundle By Name(w377) -> ("Name"=w376:string)
                }
                "DeviceNames" <- w344
                n78 = property on="Mirror" class="Ring (strict)"("Strings []"=w344) -> ()  [unwired: 2 in, 2 out]
                n79 = property on="Image Selector" class="Ring (strict)"("Strings []"=string[] ["Acquired Image", "Averaged Image", "Thresholded Image"], "Value"=0) -> ()  [unwired: 2 in, 2 out]
                n80 = property on="Corr" class="Arr (strict)"("Number of Rows"=w317) -> ()  [unwired: 2 in, 2 out]
                n81 = property on="Auto" class="Arr (strict)"("Number of Rows"=w317) -> ()  [unwired: 2 in, 2 out]
                n82 = property on="Mirrors" class="Arr (strict)"("Number of Rows"=u32 9) -> ()  [unwired: 2 in, 2 out]
                n83 = local write "USB cameras"(0 ("USB cameras")) -> ()
                n84 = property on="USB cameras" class="LstBox (strict)"("Item Names"=w329) -> ()  [unwired: 2 in, 2 out]
                n85 = for {
                  N: w317 -> [_]
                  tunnel: [w371] -> w338 mode=indexing
                  tunnel: w329 -> [w370] mode=indexing
                  tunnel: w344 -> [w369]
                  n86 = Search 1D Array(1D array=w369, element=w370) -> (index of element=w371:i32)  [unwired: 1 in]
                }
                n87 = local write "First step"(FALSE ("First step")) -> ()
                n88 = Initialize Array("" ("time string"), w317) -> (→"Last Move":string[])
                n89 = property on="USB cameras Indic" class="LstBox (strict)"("Item Names"=w329) -> ()  [unwired: 2 in, 2 out]
                n90 = local write "Mirrors"(w338) -> ()
                n91 = Initialize Array(FALSE, w317) -> (w324:bool[])
                n92 = Initialize Array("Not tried detection yet" ("time string"), w317) -> (→"Detection status":string[])
                n93 = Initialize Array(TRUE, w317) -> (w322:bool[])
                n94 = local write "CamOn"(w322) -> ()
                n95 = local write "Auto"(w324) -> ()
                n96 = local write "Corr"(w324) -> ()
              }
              frame #2 {
                w383 = T29 1 items=["Grayscale (U8)", "Grayscale (I16)", "Grayscale (SGL)", "Complex (CSG)", "RGB (U32)", "HSL (U32)", "RGB (U64)"] ("Image Type")
                n97 = local read "DeviceList"() -> (w378:T16)
                n98 = local read "Mirrors"() -> (w385:u8[])
                n99 = call "associate mirrors and cameras.vi"("Mirrors"=w385, "DeviceList"=w378) -> ("CamConfigArray"=w384:T9)  [unwired: 1 in]
                n100 = local write "CamConfigArray"(w384) -> ()
                n101 = for {
                  tunnel: w384 -> [_] mode=indexing
                  tunnel: w383 -> [w387]
                  tunnel: [w397] -> w382 mode=indexing
                  tunnel: ["images created" ("status")] -> w381
                  tunnel: [w391] -> w380 mode=indexing
                  tunnel: [w386] -> w379 mode=indexing
                  i -> [w398]
                  n102 = Number To Decimal String(number=w398) -> (decimal integer string=w390:string)  [unwired: 1 in]
                  n103 = Concatenate Strings("imageserver" ("string"), w390) -> (w394:string)
                  n104 = call "IMAQ Create"("Image Name"=w394, "Image Type"=w387) -> ("New Image"=w397:T1)  [unwired: 2 in, 2 out]
                  n105 = Concatenate Strings("imageserver2" ("string"), w390) -> (w392:string)
                  n106 = Concatenate Strings("imageserverAnn" ("string"), w390) -> (w388:string)
                  n107 = call "IMAQ Create"("Image Name"=w392, "Image Type"=w387) -> ("New Image"=w391:T1)  [unwired: 2 in, 2 out]
                  n108 = call "IMAQ Create"("Image Name"=w388, "Image Type"=w387) -> ("New Image"=w386:T1)  [unwired: 2 in, 2 out]
                }
                "Raw images" <- w382
                "Images for analysis" <- w380
                "Ann. Images" <- w379
                n109 = local write "Status"(w381) -> ()
              }
            }
          }
          frame #1 {
            n110 = local read "CamConfigArray"() -> (w404:T9)
            n111 = while {
              stop <- w710 stop-if-true
              n112 = local read "LoopMode"() -> (w704:bool)
              n113 = local read "restart"() -> (w710:bool)
              n114 = local read "LoopMode"() -> (w709:bool)
              n115 = case shown="True" w709 {
                tunnel: ["USB cameras" w718] -> w705
                frame False {
                  # "Manual mode"
                }
                frame True {
                  # "Automatic mode"
                  n116 = stacked-sequence {
                    tunnel: [_ w724] -> w718
                    frame #0 {
                      n117 = local read "USB cameras"() -> (w720:i32)
                      n118 = Increment(x=w720) -> (x+1=w719:i32)
                      n119 = local write "USB cameras"(w719) -> ()
                    }
                    frame #1 {
                      n120 = local read "USB cameras"() -> (w722:i32)
                      n121 = local read "# of cams"() -> (w723:i32)
                      n122 = Less Or Equal?(x=w723, y=w722) -> (x <= y?=w725:bool)
                      n123 = Select(t=0, s=w725, f=w722) -> (s? t:f=w724:i32)
                    }
                  }
                }
              }
              n124 = local write "USB cameras Indic"(w705) -> ()
              n125 = local write "USB cameras"(w705) -> ()
              n126 = local read "RunON/OFF"() -> (w707:bool)
              n127 = case shown="True" w704 {
                tunnel: w707 -> [w711 w715]
                tunnel: [w711 w714] -> w706
                tunnel: w705 -> [_ w712]
                frame False {
                }
                frame True {
                  n128 = local read "Auto"() -> (w716:bool[])
                  n129 = Index Array(array=w716, index=w712) -> (element=w713:bool)
                  n130 = And(x=w713, y=w715) -> (x .and. y?=w714:bool)
                }
              }
              n131 = local read "CamConfigArray"() -> (w708:T9)
              n132 = case shown="True" w706 {
                tunnel: w705 -> [_ w730]
                tunnel: w708 -> [_ w729]
                tunnel: w705 -> [_ w727]
                frame False {
                  n133 = Wait (ms)(milliseconds to wait=u32 200 ("millisecond timer value")) -> ()  [unwired: 1 out]
                }
                frame True {
                  n134 = while {
                    tunnel: w730 -> [w738]
                    shift-right: [w734] -> w728
                    shift-left: w729 -> [w735]
                    shift-right: [w731] -> _
                    shift-left: w727 -> [w731]
                    i -> [w736]
                    stop <- w737 stop-if-true
                    n135 = local read "USB cameras"() -> (w733:i32)
                    n136 = Not Equal?(x=w733, y=w731) -> (x != y?=w732:bool)
                    n137 = stacked-sequence {
                      seq-local: [_ _ _ _ _ w1009 _ _ _ _ _ _ _ _ _ _ _ _ _ _] -> [_ _ _ _ _ _ w1084 _ _ _ _ _ _ _ _ _ _ _ _ _]
                      seq-local: [_ _ _ _ _ w1008 _ _ _ _ _ _ _ _ _ _ _ _ _ _] -> [_ _ _ _ _ _ w1083 _ _ _ _ _ _ _ _ _ _ w1468 _ _]
                      seq-local: [_ _ _ _ _ w1007 _ _ _ _ _ _ _ _ _ _ _ _ _ _] -> [_ _ _ _ _ _ w1073 _ _ _ _ _ _ _ w1365 _ _ _ _ _]
                      seq-local: [_ _ _ _ _ w1000 _ _ _ _ _ _ _ _ _ _ _ _ _ _] -> [_ _ _ _ _ _ w1079 _ _ _ _ _ _ _ _ _ _ _ _ _]
                      seq-local: [_ _ _ _ w939 _ _ _ _ _ _ _ _ _ _ _ _ _ _ _] -> [_ _ _ _ _ w998 _ _ _ _ _ _ _ _ _ _ _ _ _ _]
                      seq-local: [_ _ _ _ w959 _ _ _ _ _ _ _ _ _ _ _ _ _ _ _] -> [_ _ _ _ _ w1005 _ _ _ _ _ _ _ _ _ _ _ _ _ _]
                      seq-local: [_ _ _ _ w958 _ _ _ _ _ _ _ _ _ _ _ _ _ _ _] -> [_ _ _ _ _ w999 _ _ _ _ _ _ _ _ _ _ _ _ _ _]
                      tunnel: w738 -> [w740 w807 _ w901 w942 _ w1064 _ w1159 _ _ _ _ w1305 w1364 w1377 _ _ _ w1627]
                      tunnel: [_ _ _ _ _ _ _ _ _ _ _ _ _ _ _ _ _ _ _ w1624] -> w737
                      tunnel: w736 -> [w741 _ _ _ _ _ _ _ _ _ _ _ _ _ _ _ _ _ _ w1616]
                      tunnel: w735 -> [w739 w808 _ w910 _ _ _ _ _ _ _ _ _ w1309 _ _ _ _ w1547 w1615]
                      tunnel: [_ _ _ _ _ _ _ _ _ _ _ _ _ _ _ _ _ _ _ w1614] -> w734
                      tunnel: w732 -> [_ _ _ _ _ _ _ _ _ _ _ _ _ _ _ _ _ _ _ w1613]
                      frame #0 {
                        n138 = case shown="0" w741 {
                          tunnel: w740 -> [w789 _]
                          tunnel: w739 -> [w787 _]
                          frame 0 {
                            w783 = T29 0 items=["Grayscale (U8)", "Grayscale (I16)", "Grayscale (SGL)", "Complex (CSG)", "RGB (U32)", "HSL (U32)", "RGB (U64)"] ("Image Type")
                            # "create buffer image"
                            n139 = Index Array(array=w787, index=w789) -> (element=w776:T36)
                            n140 = local read "error CamS"() -> (w785:errorcluster)
                            n141 = Unbundle By Name(w776) -> ("CorrectConfig Cluster.Detection Parameters"=w775:T21, "CorrectConfig Cluster.Reverse"=w774:cluster{"Reverse X":bool, "Reverse Y":bool}, "CorrectConfig Cluster.Target"=w773:cluster{"X Target":sgl, "Y Target":sgl}, "CorrectConfig Cluster.Region of Interest"=w772:i32[], "CorrectConfig Cluster.Correction Parameters"=w771:cluster{"X":sgl, "Y":sgl, "Movement Type":u16}, "CorrectConfig Cluster.Reference Path"=w765:path, "CorrectConfig Cluster.Background Path"=w764:path, "CorrectConfig Cluster.Acquisition Parameters"=w770:T27, "CorrectConfig Cluster.XCalibration"=w767:cluster{dbl, dbl}[], "CorrectConfig Cluster.YCalibration"=w766:cluster{dbl, dbl}[], "Name"=→"CurrentName":string, "ImageServer"=→"Current ImageServer":cluster{"IPAddress":string, "Port":i32})
                            n142 = call <vilib>:"Clear Errors.vi"("error in (no error)"=w785) -> ("error out"=w786:errorcluster)  [unwired: 6 in]
                            n143 = local read "# imgs to avg"() -> (w784:i32)
                            n144 = case shown="False" FALSE {
                              tunnel: [w794 w795] -> w790
                              frame False {
                                n145 = local read "Auto"() -> (w794:bool[])
                              }
                              frame True {
                                n146 = local read "Corr"() -> (w795:bool[])
                              }
                            }
                            n147 = call "Create Image Array.vi"("# of imgs"=w784, "Image Array Base Name"="Buffer", "error in (no error)"=w786, "Image Type"=w783) -> ("Img Array"=w781:T1[], "error out"=w780:errorcluster)  [unwired: 1 in, 9 out]
                            n148 = local write "Img Buffer"(w781) -> ()
                            n149 = Index Array(array=w790, index=w789) -> (element=w788:bool)
                            n150 = local write "error CamS"(w780) -> ()
                            n151 = local write "Feedback"(w788) -> ()
                            n152 = local write "Y calibration"(w766) -> ()
                            n153 = local write "X calibration"(w767) -> ()
                            n154 = local write "Acquisition Parameters dx"(w770) -> ()
                            n155 = local read "Mirrors"() -> (w760:u8[])
                            n156 = for {
                              tunnel: w760 -> [w798] mode=indexing
                              tunnel: [w796] -> w743 mode=indexing
                              n157 = local read "DeviceNames"() -> (w797:string[])
                              n158 = Index Array(array=w797, index=w798) -> (element=w796:string)
                            }
                            "MirrorsNames" <- w743
                            n159 = local write "Background Path"(w764) -> ()
                            n160 = local write "Acquisition Parameters"(w770) -> ()
                            n161 = local write "Detection Parameters"(w775) -> ()
                            n162 = local write "Target"(w773) -> ()
                            n163 = local write "Reverse"(w774) -> ()
                            n164 = local write "Reference Path"(w765) -> ()
                            n165 = property on="Region of Interest" class="Arr (strict)"("Val(Sgnl)"=w772) -> ()  [unwired: 2 in, 2 out]
                            n166 = property on="Correction Parameters" class="Clust (strict)"("Val(Sgnl)"=w771) -> ()  [unwired: 2 in, 2 out]
                            n167 = local read "Background Img"() -> (w762:T1)
                            n168 = local read "Reference Img"() -> (w763:T1)
                            n169 = Initialize Array(T31 {"X Intensity"=[], "Y Intensity"=[], "Max Intensity"=0, "Center"={"X"=0, "Y"=0}, "Radius"={"Rx"=0, "Ry"=0}} ("ImgData"), 0 ("dimension size")) -> (w793:T37)
                            n170 = call "LoadImages.vi"("usb"=FALSE, "Background Img"=w762, "Background Path"=w764, "Reference Img"=w763, "Reference Path"=w765) -> ()  [unwired: 7 in]
                            n171 = local write "ImgDataArray"(w793) -> ()
                            n172 = Initialize Array("no cam", 9 ("dimension size")) -> (w756:string[])
                            n173 = local read "Switch in"() -> (w779:u32)
                            n174 = Replace Array Subset(array=w756, new element=w743, index=0) -> (w754:string[])
                            n175 = Tick Count (ms)() -> (millisecond timer value=w777:u32)
                            "OpenTime" <- w777
                            n176 = Index Array(array=w754) -> (element #1=w753:string, element #2=w752:string, element #3=w751:string, element #4=w750:string, element #5=w749:string, element #6=w748:string, element #7=w745:string, element #8=w747:string, element #9=w746:string)  [unwired: 9 in]
                            n177 = Subtract(x=w777, y=w779) -> (x-y=→"Switch Time":u32)
                            n178 = local write "Onward"(TRUE ("Onward")) -> ()
                            n179 = property on="Image" class="ImageControl"("Caption.Text"=w753) -> ()  [unwired: 2 in, 2 out]
                            n180 = property on="Image 2" class="ImageControl"("Caption.Text"=w752) -> ()  [unwired: 2 in, 2 out]
                            n181 = property on="Image 3" class="ImageControl"("Caption.Text"=w751) -> ()  [unwired: 2 in, 2 out]
                            n182 = property on="Image 4" class="ImageControl"("Caption.Text"=w750) -> ()  [unwired: 2 in, 2 out]
                            n183 = property on="Image 5" class="ImageControl"("Caption.Text"=w749) -> ()  [unwired: 2 in, 2 out]
                            n184 = property on="Image 6" class="ImageControl"("Caption.Text"=w748) -> ()  [unwired: 2 in, 2 out]
                            n185 = property on="Image 7" class="ImageControl"("Caption.Text"=w745) -> ()  [unwired: 2 in, 2 out]
                            n186 = property on="Image 8" class="ImageControl"("Caption.Text"=w747) -> ()  [unwired: 2 in, 2 out]
                            n187 = property on="Image 9" class="ImageControl"("Caption.Text"=w746) -> ()  [unwired: 2 in, 2 out]
                            "Iteration" <- u32 0 ("Iteration")
                          }
                          frame 1, Default {
                          }
                        }
                      }
                      frame #1 {
                        n188 = local read "Min time between moves (s)"() -> (w806:u32)
                        n189 = local read "MoveInProgress"() -> (w804:bool)
                        n190 = local read "last move time"() -> (w811:u32)
                        n191 = local read "NewAvg"() -> (w800:bool)
                        n192 = Tick Count (ms)() -> (millisecond timer value=w812:u32)
                        n193 = local read "Beam Detected"() -> (w805:bool)
                        n194 = expression code="x*1000" "[ms/s]"(w806) -> (w809:u32)
                        n195 = Subtract(x=w812, y=w811) -> (x-y=w810:u32)
                        n196 = Not(x=w804) -> (.not. x?=w801:bool)
                        n197 = Greater?(x=w810, y=w809) -> (0:w803:bool)
                        n198 = Compound Arithmetic op=AND(w803, "Calibrate", w801, w800) -> (w799:bool)
                        n199 = case shown="True" w799 {
                          tunnel: w808 -> [_ w815]
                          tunnel: w807 -> [_ w814]
                          tunnel: w805 -> [_ w813]
                          frame False {
                            n200 = call "Send Move Command.vi"() -> ()  [unwired: 4 in, 3 out]
                          }
                          frame True {
                            n201 = case shown="True" w813 {
                              tunnel: w815 -> [_ w846]
                              tunnel: w814 -> [_ w845]
                              frame False {
                                n202 = local write "Calibrate"(FALSE ("Calibrate")) -> ()
                              }
                              frame True {
                                w831 = 0.0 ("y")
                                w840 = T38 {"Down"=FALSE, "Up"=FALSE, "Right"=FALSE, "Left"=FALSE, "APulses X"=0, "APulses Y"=0, "Stop"=FALSE} ("Corrective Move")
                                # "picomotor goes onwards and then backwards. And starts this cycle again while going further. All for the purpose of calibrating the motors"
                                n203 = local read "Correction Parameters"() -> (w844:cluster{"X":sgl, "Y":sgl, "Movement Type":u16})
                                n204 = Tick Count (ms)() -> (millisecond timer value=w843:u32)
                                n205 = Index Array(array=w846, index=w845) -> (element=w828:T36)
                                n206 = local write "last move time"(w843) -> ()
                                n207 = local read "Iteration"() -> (w822:u32)
                                n208 = Unbundle By Name(w844) -> ("X"=w842:sgl, "Y"=w841:sgl)
                                n209 = Increment(x=w822) -> (x+1=w817:u32)
                                n210 = Multiply(x=w841, y=w817) -> (x*y=w830:sgl)
                                n211 = Not(x="Onward") -> (.not. x?=w824:bool)
                                n212 = Greater?(x=w817, y=u32 0) -> (0:w826:bool)
                                n213 = Multiply(x=w842, y=w817) -> (x*y=w829:sgl)
                                n214 = Not(x="Onward") -> (.not. x?=w838:bool)
                                n215 = case shown="False" w824 {
                                tunnel: w817 -> [_ w887]
                                frame False {
                                }
                                frame True {
                                n216 = local write "Iteration"(w887) -> ()
                                }
                                }
                                n217 = Bundle By Name(cluster=w840, "Right"="Onward", "Left"=w838, "APulses X"=w829) -> (w837:T38)
                                n218 = local write "Onward"(w824) -> ()
                                n219 = Or(x=w826, y=w824) -> (x .or. y?=w825:bool)
                                n220 = Bundle By Name(cluster=w840, "Up"="Onward", "Down"=w838, "APulses Y"=w830) -> (w836:T38)
                                n221 = local read "ConnectArray"() -> (w848:T7)
                                n222 = local read "Correction Parameters"() -> (w823:cluster{"X":sgl, "Y":sgl, "Movement Type":u16})
                                n223 = Build Array(w837, w836) -> (w835:T39)
                                n224 = Not Equal?(x=w830, y=w831) -> (x != y?=w834:bool)
                                n225 = Not Equal?(x=w829, y=w831) -> (x != y?=w833:bool)
                                n226 = Or(x=w834, y=w833) -> (x .or. y?=w832:bool)
                                n227 = Unbundle By Name(w823) -> ("X"=w821:sgl, "Y"=w820:sgl)
                                n228 = case shown="True" w832 {
                                tunnel: w848 -> [_ w886]
                                tunnel: "webcam" ("client name") -> [_ w883]
                                tunnel: w828 -> [_ w882]
                                tunnel: w835 -> [_ w880]
                                frame False {
                                }
                                frame True {
                                # "Change the direction of the move"
                                n229 = call "Send Move Command.vi"("ConnectArray IN"=w886, "client name"=w883, "CamConfig"=w882, "Move XY"=w880) -> ("ConnectArray Out"=w881:T7, "TCPconnecCmd"=w884:bool, "status"=w885:string)
                                n230 = local write "Status"(w885) -> ()
                                n231 = local write "TCPconnecCmd"(w884) -> ()
                                n232 = local write "ConnectArray"(w881) -> ()
                                }
                                }
                                n233 = Multiply(x=w820, y=w817) -> (x*y=w818:sgl)
                                n234 = Multiply(x=w817, y=w821) -> (x*y=w819:sgl)
                                n235 = case shown="True" w825 {
                                tunnel: w824 -> [_ w854]
                                tunnel: w818 -> [_ w853]
                                tunnel: w819 -> [_ w852]
                                frame False {
                                }
                                frame True {
                                n236 = local read "BestRects Cluster"() -> (w858:T12)
                                n237 = Unbundle By Name(w858) -> ("PreviousCenter"=w856:cluster{"X":dbl, "Y":dbl}, "CurrentCenter"=w855:cluster{"X":dbl, "Y":dbl})
                                n238 = Bundle By Name(cluster=w858, "PreviousCenter"=w855) -> (w857:T12)
                                n239 = Subtract(x=w856, y=w855) -> (x-y=w849:cluster{"X":dbl, "Y":dbl})
                                n240 = local write "BestRects Cluster"(w857) -> ()
                                n241 = Unbundle By Name(w849) -> ("X"=w851:dbl, "Y"=w850:dbl)
                                n242 = case shown="True" w854 {
                                tunnel: w852 -> [w862 w878]
                                tunnel: w853 -> [w861 _]
                                tunnel: w851 -> [w860 w870]
                                tunnel: w850 -> [w859 w869]
                                frame False {
                                n243 = local read "X calibration"() -> (w866:cluster{dbl, dbl}[])
                                n244 = local read "Y calibration"() -> (w863:cluster{dbl, dbl}[])
                                n245 = Bundle(w862, "X"=w860) -> (w865:cluster{sgl, "X":dbl})  [unwired: 1 in]
                                n246 = Bundle(w861, "Y"=w859) -> (w864:cluster{sgl, "Y":dbl})  [unwired: 1 in]
                                n247 = Build Array (concatenate)(w866, w865) -> (w868:cluster{dbl, "X":dbl}[])
                                n248 = Build Array (concatenate)(w863, w864) -> (w867:cluster{dbl, "Y":dbl}[])
                                n249 = local write "X calibration"(w868) -> ()
                                n250 = local write "Y calibration"(w867) -> ()
                                }
                                frame True {
                                n251 = Negate(x=w878) -> (-x=w877:sgl)
                                n252 = Negate(x=w878) -> (-x=w879:sgl)
                                n253 = local read "X calibration"() -> (w875:cluster{dbl, dbl}[])
                                n254 = local read "Y calibration"() -> (w872:cluster{dbl, dbl}[])
                                n255 = Bundle(w877, "X"=w870) -> (w876:cluster{sgl, "X":dbl})  [unwired: 1 in]
                                n256 = Bundle(w879, "Y"=w869) -> (w871:cluster{sgl, "Y":dbl})  [unwired: 1 in]
                                n257 = Build Array (concatenate)(w876, w875) -> (w874:cluster{dbl, "X":dbl}[])
                                n258 = Build Array (concatenate)(w871, w872) -> (w873:cluster{dbl, "Y":dbl}[])
                                n259 = local write "X calibration"(w874) -> ()
                                n260 = local write "Y calibration"(w873) -> ()
                                }
                                }
                                }
                                }
                              }
                            }
                          }
                        }
                      }
                      frame #2 {
                        w893 = FALSE ("Move X?")
                        n261 = local write "Move X"(w893) -> ()
                        n262 = local write "Move Y"(w893) -> ()
                        n263 = case shown="True" "Set Target (Cursor)" {
                          frame False {
                          }
                          frame True {
                            n264 = property on="Displayed Image" class="IntGraph (strict)"("Active Cursor"=u32 0) -> ("Cursor.Cursor Position"=w900:T40)  [unwired: 2 in, 2 out]
                            n265 = local write "Target"(w900) -> ()
                          }
                        }
                        n266 = local write "NewAvg"(FALSE ("NewAvg")) -> ()
                        n267 = Tick Count (ms)() -> (millisecond timer value=→"start":u32)
                        n268 = local write "State"(0) -> ()
                        n269 = Initialize Array(T3 {"Down"=FALSE, "Up"=FALSE, "Right"=FALSE, "Left"=FALSE, "APulses X"=0, "APulses Y"=0, "StopButton"=FALSE} ("Corrective Move"), 2 ("dimension size")) -> (w888:T5)
                        n270 = case shown="False" "Set Centroid as Target" {
                          frame False {
                          }
                          frame True {
                            n271 = local read "ImgData Avg"() -> (w898:T23)
                            n272 = Unbundle By Name(w898) -> ("Centroid Avg"=w897:cluster{"X":sgl, "Y":sgl})
                            n273 = local write "Target"(w897) -> ()
                          }
                        }
                        n274 = local write "Corrective Move XY"(w888) -> ()
                      }
                      frame #3 {
                        # "Send Manual Command"
                        n275 = Index Array(array=w910, index=w901) -> (element=w905:T36)
                        n276 = Bundle By Name(cluster="Manual Move", "APulses X"="Step Size", "APulses Y"="Step Size") -> (w902:T3)
                        n277 = Unbundle By Name(w902) -> ("StopButton"=w911:bool, "Right"=w915:bool, "Left"=w914:bool, "Up"=w913:bool, "Down"=w912:bool)
                        n278 = local read "Calibrate"() -> (w907:bool)
                        n279 = Compound Arithmetic op=OR(w911, w915, w914, w913, w912) -> (w909:bool)
                        n280 = Not(x=w907) -> (.not. x?=w908:bool)
                        n281 = And(x=w909, y=w908) -> (x .and. y?=w906:bool)
                        n282 = case shown="True" w906 {
                          tunnel: w905 -> [_ w932]
                          tunnel: w902 -> [_ w931]
                          tunnel: w901 -> [_ w918]
                          frame False {
                          }
                          frame True {
                            n283 = local read "ConnectArray"() -> (w928:T7)
                            n284 = Initialize Array(w931, 1 ("dimension size")) -> (w930:T5)
                            n285 = Get Date/Time In Seconds() -> (seconds since 1Jan1904=w923:timestamp)
                            n286 = call "Send Move Command.vi"("ConnectArray IN"=w928, "client name"="webcam", "CamConfig"=w932, "Move XY"=w930) -> ("ConnectArray Out"=w927:T7, "TCPconnecCmd"=w925:bool, "status"=w926:string)
                            n287 = local read "Last Move"() -> (w921:string[])
                            n288 = Get Date/Time String(seconds (now)=w923, want seconds? (F)=TRUE) -> (time string=w920:string)  [unwired: 1 in, 1 out]
                            n289 = Replace Array Subset(array=w921, new element=w920, index=w918) -> (w919:string[])
                            n290 = local write "TCPconnecCmd"(w925) -> ()
                            n291 = local write "ConnectArray"(w927) -> ()
                            n292 = local write "Status"(w926) -> ()
                            n293 = local write "Last Move"(w919) -> ()
                          }
                        }
                        n294 = local write "State"(1) -> ()
                        n295 = disable-structure shown="Disabled" {
                          frame Disabled {
                            n296 = Bundle By Name("DeviceID"=T32 {"Slot Connector"=0, "IP Adress"="127.0.0.1", "Port"=63410, "Type"="picodriver"}) -> ()  [unwired: 1 in, 1 out]
                          }
                          frame Enabled {
                          }
                        }
                      }
                      frame #4 {
                        # "get image"
                        n297 = local read "Buffer3"() -> (w937:T1)
                        n298 = local read "USB cameras"() -> (w934:i32)
                        n299 = local read "Image IPs"() -> (w935:string[])
                        n300 = while {
                          shift-right: [w988] -> w938
                          shift-left: w937 -> [w984]
                          tunnel: w942 -> [w972]
                          i -> [w985]
                          stop <- w987 stop-if-true
                          n301 = local read "USB cameras"() -> (w983:i32)
                          n302 = local read "DownloadedImg"() -> (w977:T1)
                          n303 = Equal?(x=w972, y=w983) -> (x = y?=w982:bool)
                          n304 = local read "RunON/OFF"() -> (w979:bool)
                          n305 = local read "restart"() -> (w980:bool)
                          n306 = local read "Raw images"() -> (w973:T1[])
                          n307 = local read "stop"() -> (w981:bool)
                          n308 = Not(x=w982) -> (.not. x?=w975:bool)
                          n309 = local read "Buffer2"() -> (w974:T1)
                          n310 = call "Update image if new.vi"("Raw images"=w973, "Image Dst"=w984, "DownloadedImg"=w977, "USB cameras"=w972, "Buffer2"=w974) -> ("Image Dst Out"=w988:T1, "Image ok"=w976:bool)
                          n311 = Not(x=w979) -> (.not. x?=w978:bool)
                          n312 = Compound Arithmetic op=OR(w976, w981, w980, w978, w975) -> (w987:bool)
                          n313 = Wait (ms)(milliseconds to wait=u32 250) -> ()  [unwired: 1 out]
                          "#loops waiting for new image" <- w985
                        }
                        n314 = Index Array(array=w935, index=w934) -> (element=→"Image IP":string)
                        n315 = local read "Acq Img"() -> (w936:T1)
                        n316 = case shown="True" "smooth" {
                          tunnel: w938 -> [w966 w970]
                          tunnel: [w964 w969] -> w941
                          tunnel: w936 -> [w965 w967]
                          frame False {
                            n317 = call "IMAQ Copy"("Image Dst"=w965, "Image Src"=w966) -> ("Image Dst Out"=w964:T1)  [unwired: 4 in, 1 out]
                          }
                          frame True {
                            n318 = call "IMAQ LowPass"("Image Src"=w970, "Size & Tolerance"="Size & Tolerance", "Image Dst"=w967) -> ("Image Dst Out"=w969:T1, "error out"=→"error out":errorcluster)  [unwired: 4 in]
                          }
                        }
                        n319 = local read "Region of Interest"() -> (w943:i32[])
                        n320 = property class="IMAQImage"(reference=w941) -> (reference out=w957:T1, error out=w956:errorcluster, "ImageSize"=w955:cluster{"x":i32, "y":i32})  [unwired: 1 in]
                        n321 = Equal?(x=i32[] [0, 0, 0, 0] ("Region of Interest"), y=w943) -> (x = y?=w962:bool)
                        n322 = case shown="False" w962 {
                          tunnel: w956 -> [w990 w994]
                          tunnel: [w991 w994] -> w960
                          tunnel: w957 -> [w993 w995]
                          tunnel: [w992 w995] -> w939
                          tunnel: w943 -> [w989 _]
                          frame False {
                            # "Apply ROI"
                            n323 = call "IMAQ Extract"("Optional Rectangle"=w989, "error in (no error)"=w990, "Image Src"=w993) -> ("error out"=w991:errorcluster, "Image Dst Out"=w992:T1)  [unwired: 7 in]
                          }
                          frame True {
                          }
                        }
                        n324 = Unbundle By Name(w955) -> ("x"=w949:i32, "y"=w951:i32)
                        n325 = Replace Array Subset(array=i32[] [0, 0, 0, 0] ("Region of Interest"), new element #1=w949, index #1=2 ("index"), new element #2=w951, index #2=3 ("index")) -> (→"Img Size":i32[])
                        n326 = local read "Reference Img"() -> (w947:T1)
                        n327 = local read "Background Img"() -> (w944:T1)
                        n328 = local read "Output Img"() -> (w945:T1)
                        n329 = call "Substract Background.vi"("Background"=w944, "Substract"="Substract", "error in (no error)"=w960, "Reference"=w947, "Dest Img"=w945, "Region of Interest"=w943, "Image Src"=w939) -> ("error out"=w959:errorcluster, "Img Out"=w946:T1)  [unwired: 2 in]
                        n330 = local write "Output Img"(w946) -> ()
                        n331 = Unbundle By Name(w959) -> ("status"=w961:bool)
                        "IMAQ status" <- w961
                        n332 = Not(x=w961) -> (.not. x?=w958:bool)
                      }
                      frame #5 {
                        # "decide wether or not to do the beam detection"
                        n333 = call "Run Centroid Detection.vi"("Detection Parameters"="Detection Parameters") -> ("Run Detection"=w1003:bool)
                        n334 = Or(x="Auto Detect Param", y=w1003) -> (x .or. y?=w1001:bool)
                        n335 = Not(x="Select ROI") -> (.not. x?=w1002:bool)
                        n336 = local write "Centroid Detection"(w1001) -> ()
                        n337 = And(x=w1001, y=w1002) -> (x .and. y?=w1000:bool)
                        n338 = And(x=w1000, y=w999) -> (x .and. y?=w1006:bool)
                        n339 = case shown="True" w1006 {
                          tunnel: w998 -> [w1016 w1028]
                          tunnel: [w1015 w1037] -> w1009
                          tunnel: [_ w1036] -> w1008
                          tunnel: [_ w1031] -> w1007
                          tunnel: w1005 -> [w1014 w1035]
                          tunnel: "Detection Parameters" -> [_ w1018]
                          frame False {
                            w1017 = T29 0 items=["Grayscale (U8)", "Grayscale (I16)", "Grayscale (SGL)", "Complex (CSG)", "RGB (U32)", "HSL (U32)", "RGB (U64)", "Grayscale (U16)"] ("Image Type")
                            n340 = local write "ImgDataArray"(T15 [] ("ImgDataArray")) -> ()
                            n341 = call "IMAQ Cast Image"("Image Type"=w1017, "error in (no error)"=w1014, "Image Src"=w1016) -> ("error out"=w1013:errorcluster, "Image Dst Out"=w1015:T1)  [unwired: 3 in, 4 out]
                            n342 = local write "error CamS"(w1013) -> ()
                            "Beam Detected" <- FALSE ("Beam Detected")
                          }
                          frame True {
                            # "beam detection"
                            n343 = local read "Display"() -> (w1030:T26)
                            n344 = Unbundle By Name(w1030) -> ("Show Best Rect"=w1039:bool, "Show Centroid"=w1038:bool)
                            n345 = local read "Pretreatment"() -> (w1019:bool)
                            n346 = Bundle("Show Best Rect"=w1039, "Show Centroid"=w1038) -> (w1040:T41)  [unwired: 1 out]
                            n347 = call "Beam Detection-v6.vi"("Image Src"=w1028, "Pretreatment"=w1019, "DetectionParameters"=w1018, "error in"=w1035, "Display"=w1040) -> ("Ellipse"=→"Ellipse":T10, "Image Out"=w1029:T1, "Beam is IN"=w1042:bool, "Ellipse edges"=→"Ellipse edges":cluster{"X":sgl, "Y":sgl}[], "Best Rectangle"=w1026:T13, "ImgData"=w1041:T42, "error out"=w1027:errorcluster)  [unwired: 8 in]
                            n348 = case shown="False" w1042 {
                              selector: w1042 -> [_ w1061]
                              tunnel: w1029 -> [w1052 w1060]
                              tunnel: [w1057 w1062] -> w1032
                              tunnel: w1041 -> [_ w1062]
                              tunnel: [w1056 w1061] -> w1020
                              tunnel: [w1047 w1059] -> w1036
                              tunnel: w1027 -> [w1050 w1058]
                              tunnel: [w1055 w1058] -> w1034
                              tunnel: w1040 -> [w1053 _]
                              tunnel: [w1049 w1060] -> w1037
                              tunnel: w1018 -> [w1048 _]
                              tunnel: w1026 -> [_ w1059]
                              tunnel: w1019 -> [w1046 _]
                              frame False {
                                n349 = call "IMAQ GetImageSize"("Image"=w1052) -> ()  [unwired: 1 in, 5 out]
                                n350 = call "IMAQ Clear Overlay"("error in (no error)"=w1050, "Image"=w1052) -> ("error out"=w1051:errorcluster, "Image Out"=w1054:T1)  [unwired: 1 in, 7 out]
                                n351 = call "Beam Detection-v6.vi"("Image Src"=w1054, "Pretreatment"=w1046, "DetectionParameters"=w1048, "error in"=w1051, "Display"=w1053) -> ("Image Out"=w1049:T1, "Beam is IN"=w1056:bool, "Best Rectangle"=w1047:T13, "ImgData"=w1057:T42, "error out"=w1055:errorcluster)  [unwired: 8 in, 2 out]
                              }
                              frame True {
                              }
                            }
                            n352 = local read "Region of Interest"() -> (w1033:i32[])
                            n353 = call-poly "Add ROI Offset.vi"("Region of Interest"=w1033, "ImgData In"=w1032) -> ("ImgData Out"=w1031:T43)  [unwired: 3 in]
                            n354 = case shown="True" w1020 {
                              tunnel: w1034 -> [_ w1045]
                              frame False {
                              }
                              frame True {
                                n355 = local write "error CamS"(w1045) -> ()
                              }
                            }
                            n356 = local read "Beam Detected"() -> (w1023:bool)
                            n357 = Not(x=w1023) -> (.not. x?=w1021:bool)
                            n358 = And(x=w1021, y=w1020) -> (x .and. y?=w1022:bool)
                            n359 = case shown="True" w1022 {
                              selector: w1022 -> [_ w1044]
                              tunnel: w1020 -> [w1043 _]
                              frame False {
                                n360 = local write "Beam Detected"(w1043) -> ()
                              }
                              frame True {
                                n361 = property on="Beam Detected" class="Bool (strict)"("Val(Sgnl)"=w1044) -> ()  [unwired: 2 in, 2 out]
                              }
                            }
                          }
                        }
                        n362 = local write "State"(3 ("State")) -> ()
                      }
                      frame #6 {
                        # "Display current centroid"
                        # "Display current data"
                        n363 = local read "Beam Detected"() -> (w1068:bool)
                        n364 = Select(t="Detected", s=w1068, f=":( Not Detected") -> (s? t:f=w1065:string)
                        n365 = local read "Detection status"() -> (w1070:string[])
                        n366 = local read "Det"() -> (w1072:bool[])
                        n367 = Replace Array Subset(array=w1072, new element=w1068, index=w1064) -> (w1071:bool[])
                        n368 = Replace Array Subset(array=w1070, new element=w1065, index=w1064) -> (w1069:string[])
                        n369 = local read "Auto Detect Param"() -> (w1081:bool)
                        n370 = local write "Det"(w1071) -> ()
                        n371 = local write "Detection status"(w1069) -> ()
                        n372 = Or(x=w1081, y=w1068) -> (x .or. y?=w1082:bool)
                        n373 = And(x=w1079, y=w1082) -> (x .and. y?=w1080:bool)
                        n374 = case shown="True" w1080 {
                          tunnel: w1084 -> [_ w1105]
                          tunnel: w1073 -> [_ w1090]
                          tunnel: w1083 -> [_ w1088]
                          frame False {
                            n375 = local read "Image Selector"() -> (w1086:u16)
                            n376 = Greater?(x=w1086, y=u16 0) -> (0:w1085:bool)
                            n377 = property on="Warning !" class="Str"("Visible"=w1085) -> ()  [unwired: 2 in, 2 out]
                          }
                          frame True {
                            # "Calculate deviation of centroid position from Target"
                            # "add data in buffer"
                            # "add image in buffer"
                            n378 = property on="Warning !" class="Str"("Visible"=FALSE) -> ()  [unwired: 2 in, 2 out]
                            n379 = local write "RectFilter"(w1088) -> ()
                            n380 = Unbundle By Name(w1090) -> ("Center"=w1094:cluster{"X":sgl, "Y":sgl})
                            n381 = local read "ImgDataArray"() -> (w1103:T15)
                            n382 = local read "error CamS"() -> (w1096:errorcluster)
                            n383 = local read "Target"() -> (w1095:cluster{"X Target":sgl, "Y Target":sgl})
                            n384 = local read "Img Buffer"() -> (w1101:T1[])
                            n385 = local read "DeviationArray"() -> (w1093:cluster{"X Centroid":sgl, "Y Centroid":sgl}[])
                            n386 = Subtract(x=w1094, y=w1095) -> (x-y=w1091:cluster{sgl, sgl})
                            "Deviation" <- w1091
                            n387 = Build Array (concatenate)(w1103, w1090) -> (w1100:T15)
                            n388 = Array Size(array=w1101) -> (size(s)=→"ImgBufferSize":i32)
                            n389 = local write "ImgDataArray"(w1100) -> ()
                            n390 = local read "# imgs to avg"() -> (w1099:i32)
                            n391 = Array Size(array=w1100) -> (size(s)=w1097:i32)
                            "# imgs in buffer" <- w1097
                            n392 = call "Copy i_th image to array v2.vi"("Img Array In"=w1101, "Image Src"=w1105, "error in (no error)"=w1096, "Index"=w1097) -> ("error out"=w1104:errorcluster)  [unwired: 10 in, 1 out]
                            n393 = local write "error CamS"(w1104) -> ()
                            n394 = Build Array (concatenate)(w1093, w1091) -> (→"DeviationArray":cluster{"X Centroid":sgl, "Y Centroid":sgl}[])
                            n395 = Equal?(x=w1097, y=w1099) -> (x = y?=w1098:bool)
                            n396 = local write "NewAvg"(w1098) -> ()
                          }
                        }
                        n397 = Unbundle By Name(w1073) -> ("Center"=w1074:cluster{"X":sgl, "Y":sgl}, "Radius"=w1077:cluster{"Rx":sgl, "Ry":sgl}, "Max Intensity"=w1076:sgl)
                        n398 = local read "Img Data"() -> (w1078:T22)
                        n399 = Bundle By Name(cluster=w1078, "Centroid"=w1074, "Radius"=w1077, "Max Intensity"=w1076) -> (→"Img Data":T22)
                        n400 = property on="Displayed Image" class="IntGraph (strict)"("Active Cursor"=u32 3, "Cursor.Cursor Position"=w1074) -> ()  [unwired: 2 in, 2 out]
                      }
                      frame #7 {
                        n401 = local read "ImgDataArray"() -> (w1110:T15)
                        n402 = local read "NewAvg"() -> (w1107:bool)
                        n403 = local read "error CamS"() -> (w1112:errorcluster)
                        n404 = local read "Img Buffer"() -> (w1111:T1[])
                        n405 = Array Size(array=w1110) -> (size(s)=w1109:i32)
                        n406 = local write "State"(5) -> ()
                        n407 = Not Equal To 0?(x=w1109) -> (x != 0?=w1106:bool)
                        n408 = And(x=w1106, y=w1107) -> (x .and. y?=w1108:bool)
                        n409 = case shown="True" w1108 {
                          tunnel: w1112 -> [_ w1137]
                          tunnel: w1111 -> [_ w1136]
                          tunnel: w1110 -> [_ w1135]
                          frame False {
                          }
                          frame True {
                            # "Display Avg Data"
                            # "average image"
                            # "sort images and average data"
                            # "averaging"
                            n410 = call "RemoveBadSpotImage-v3.vi"("error in"=w1137, "ImgDataArray"=w1135, "Img Array In"=w1136) -> ("error out"=w1133:errorcluster, "Averages"=w1129:T23, "Img Array Sorted"=w1121:T1[])  [unwired: 1 in, 1 out]
                            n411 = local read "Avg Img"() -> (w1134:T1)
                            n412 = property on="Warning !" class="Str"("Visible"=FALSE) -> ()  [unwired: 2 in, 2 out]
                            n413 = call "Greyscale Image Averager3.vi"("Img Array IN"=w1121, "Image Dst In"=w1134, "usb"=FALSE, "error in (no error)"=w1133) -> ("Img Array Out"=w1124:T1[], "Image Dst Out"=w1125:T1, "error out"=w1123:errorcluster)  [unwired: 9 in]
                            n414 = call "IMAQ Dispose Buffer.vi"("error in"=w1123, "Img Buffer In"=w1124) -> ("error out"=w1122:errorcluster)  [unwired: 1 in]
                            n415 = case shown="True" "Avg data/ data of avg img" {
                              tunnel: w1122 -> [w1140 w1158]
                              tunnel: w1125 -> [w1138 w1152]
                              tunnel: [w1140 w1151] -> w1130
                              tunnel: [w1139 w1146] -> w1116
                              tunnel: w1129 -> [w1139 _]
                              tunnel: [w1138 w1144] -> w1120
                              frame False {
                              }
                              frame True {
                                n416 = local read "Display"() -> (w1156:T26)
                                n417 = local read "Detection Parameters"() -> (w1157:T21)
                                n418 = Unbundle By Name(w1156) -> ("Show Best Rect"=w1155:bool, "Show Centroid"=w1154:bool)
                                n419 = local read "Pretreatment"() -> (w1141:bool)
                                n420 = Bundle("Show Best Rect"=w1155, "Show Centroid"=w1154) -> (w1153:T41)  [unwired: 1 out]
                                n421 = call "Beam Detection-v6.vi"("Image Src"=w1152, "Pretreatment"=w1141, "DetectionParameters"=w1157, "error in"=w1158, "Display"=w1153) -> ("Ellipse"=w1143:T10, "Image Out"=w1144:T1, "Ellipse edges"=w1142:cluster{"X":sgl, "Y":sgl}[], "ImgData"=w1150:T42, "error out"=w1151:errorcluster)  [unwired: 8 in, 2 out]
                                n422 = local write "Ellipse"(w1143) -> ()
                                n423 = local write "Ellipse edges"(w1142) -> ()
                                n424 = Unbundle By Name(w1150) -> ("Max Intensity"=w1148:u8, "Centroid"=w1145:cluster{"X":i32, "Y":i32}, "Radius"=w1147:cluster{"Rx":i32, "Ry":i32})
                                n425 = local read "ImgData Avg"() -> (w1149:T23)
                                n426 = Bundle By Name(cluster=w1149, "Max Intensity Avg"=w1148, "Centroid Avg"=w1145, "Radius Avg"=w1147) -> (w1146:T23)
                              }
                            }
                            n427 = local read "Detection Parameters"() -> (w1127:T21)
                            n428 = Unbundle By Name(w1127) -> ("Treshold"=w1126:u8)
                            n429 = local read "Thresh Img"() -> (w1132:T1)
                            n430 = call "Threshold Img v2.vi"("error in (no error)"=w1130, "Threshold"=w1126, "Img Dst"=w1132, "Img Src"=w1120) -> ("error out"=w1131:errorcluster)  [unwired: 6 in, 1 out]
                            n431 = local write "error CamS"(w1131) -> ()
                            n432 = local write "ImgData Avg"(w1116) -> ()
                            n433 = Unbundle By Name(w1116) -> ("Centroid Avg"=w1115:cluster{"X":sgl, "Y":sgl})
                            n434 = local read "BestRects Cluster"() -> (w1117:T12)
                            n435 = Bundle By Name(cluster=w1117, "CurrentCenter"=w1115) -> (w1118:T12)
                            n436 = local write "BestRects Cluster"(w1118) -> ()
                          }
                        }
                      }
                      frame #8 {
                        # "image saving"
                        n437 = local read "NewAvg"() -> (w1161:bool)
                        n438 = local read "ImgDataArray"() -> (w1165:T15)
                        n439 = Array Size(array=w1165) -> (size(s)=w1164:i32)
                        n440 = Not Equal To 0?(x=w1164) -> (x != 0?=w1162:bool)
                        n441 = Compound Arithmetic op=AND("SavePict", w1162, w1161) -> (w1160:bool)
                        n442 = case shown="True" w1160 {
                          tunnel: w1159 -> [_ w1166]
                          frame False {
                          }
                          frame True {
                            n443 = stacked-sequence {
                              seq-local: [w1168 _] -> [_ w1194]
                              tunnel: w1166 -> [_ w1181]
                              frame #0 {
                                n444 = local read "MirrorsNames"() -> (w1167:string[])
                                n445 = for {
                                tunnel: [w1170] -> w1168 mode=indexing
                                tunnel: w1167 -> [w1169] mode=indexing
                                n446 = Search and Replace String(input string=w1169, search string=":", replace string="-" ("replace string (\"\")")) -> (result string=w1173:string)  [unwired: 5 in, 3 out]
                                n447 = Build Path(base path="Base Directory", name or relative path=w1173) -> (appended path=w1172:path)
                                n448 = List Folder(path="Base Directory") -> (folder names=w1174:string[])  [unwired: 3 in, 3 out]
                                n449 = Search 1D Array(1D array=w1174, element=w1173) -> (index of element=w1171:i32)  [unwired: 1 in]
                                n450 = case shown="-1" w1171 {
                                tunnel: w1172 -> [w1178 w1180]
                                tunnel: [w1178 w1179] -> w1170
                                frame 0, Default {
                                }
                                frame -1 {
                                n451 = Create Folder(path (use dialog)=w1180) -> (created path=w1179:path)  [unwired: 2 in, 2 out]
                                }
                                }
                                }
                              }
                              frame #1 {
                                n452 = local read "Avg Img"() -> (w1186:T1)
                                n453 = local read "Beam Detected"() -> (w1198:bool)
                                n454 = call "IMAQ Create"("Image Name"="toDeinterlace") -> ("New Image"=w1190:T1)  [unwired: 4 in, 1 out]
                                n455 = Index Array(array=w1194, index=w1181) -> (element=w1193:path)
                                n456 = Select(t="Beam In.png" ("string"), s=w1198, f="Beam Out.png" ("string")) -> (s? t:f=w1196:string)
                                n457 = call "IMAQ Copy"("Image Dst"=w1190, "Image Src"=w1186) -> ("Image Dst Out"=w1182:T1)  [unwired: 4 in, 1 out]
                                n458 = local read "Main processing loop i"() -> (w1202:i32)
                                n459 = Path To String(path=w1193) -> (string=w1192:string)
                                n460 = Number To Decimal String(number=w1202) -> (decimal integer string=w1201:string)  [unwired: 1 out]
                                n461 = call "IMAQ Interlace"("Image Even"=w1182, "Image Odd"=w1182, "Image Frame"=w1182, "Interlace/Separate (Interlace)"=TRUE) -> ("Image Odd Out"=→"Image Odd Out":T1, "Image Even Out"=w1184:T1)  [unwired: 1 in, 2 out]
                                n462 = Concatenate Strings(w1192, "\\" ("string"), w1201, w1196) -> (w1203:string)
                                n463 = Select(t=w1184, s="Boolean", f=w1186) -> (s? t:f=w1185:T1)
                                n464 = String To Path(string=w1203) -> (path=w1200:path)
                                n465 = call "IMAQ Write Image And Vision Info"("File Path"=w1200, "Image"=w1185) -> ("error out"=→"SaveImgError":errorcluster)  [unwired: 2 in, 7 out]
                              }
                            }
                          }
                        }
                      }
                      frame #9 {
                        # "Calclulate average values for correction"
                        n466 = local read "NewAvg"() -> (w1206:bool)
                        n467 = case shown="True" w1206 {
                          tunnel: [w1208 w1218] -> w1205
                          tunnel: [w1208 w1212] -> w1204
                          frame False {
                            w1208 = cluster{bool, bool} {FALSE, FALSE}
                          }
                          frame True {
                            n468 = local read "ImgData Avg"() -> (w1219:T23)
                            n469 = local read "ImgData Avg"() -> (w1221:T23)
                            n470 = local read "Initiate Correction Range"() -> (w1215:i16)
                            n471 = Unbundle By Name(w1219) -> ("Centroid Avg"=w1222:cluster{"X":sgl, "Y":sgl})
                            n472 = Unbundle By Name(w1221) -> ("Radius Avg"=w1220:cluster{"Rx":sgl, "Ry":sgl})
                            n473 = local read "Target"() -> (w1216:cluster{"X Target":sgl, "Y Target":sgl})
                            n474 = local read "DeviationArray"() -> (w1209:cluster{"X Centroid":sgl, "Y Centroid":sgl}[])
                            n475 = Divide(x=w1215, y=sgl 100.0) -> (x/y=w1211:sgl)
                            n476 = Subtract(x=w1222, y=w1216) -> (x-y=w1224:cluster{sgl, sgl})
                            "Avg Deviation" <- w1224
                            n477 = Multiply(x=w1220, y=w1211) -> (x*y=w1217:cluster{"Rx":sgl, "Ry":sgl})
                            n478 = Absolute Value(x=w1224) -> (abs(x)=w1223:cluster{sgl, sgl})
                            n479 = Greater?(x=w1223, y=w1217) -> (0:w1218:cluster{bool, bool})
                            n480 = call "percent true of DeviationArray.vi"("DeviationArray"=w1209, "Threshold"=w1217) -> ("% XY State True"=w1214:cluster{dbl, dbl})  [unwired: 7 out]
                            "% XY State True" <- w1214
                            n481 = Greater?(x=w1214, y="Threshold [%]") -> (0:w1212:cluster{bool, bool})
                          }
                        }
                        "Out of Range?" <- w1205
                        "%Out of Range" <- w1204
                        n482 = local write "State"(7) -> ()
                      }
                      frame #10 {
                        # "Auto set detection parameters"
                        n483 = local read "Auto Detect Param"() -> (w1225:bool)
                        n484 = case shown="True" w1225 {
                          frame False {
                          }
                          frame True {
                            n485 = local read "Acq Img"() -> (w1227:T1)
                            n486 = local write "Auto Detect Param"(FALSE ("Auto Detect Param")) -> ()
                            n487 = call "AutoDetect.vi"("Image"=w1227) -> ("Detection Parameters Out"=w1228:T21)
                            n488 = local write "Detection Parameters"(w1228) -> ()
                          }
                        }
                      }
                      frame #11 {
                        # "Decide wether or not to initiate a correction sequence"
                        n489 = local read "Feedback"() -> (w1229:bool)
                        n490 = local read "NewAvg"() -> (w1230:bool)
                        n491 = And(x=w1229, y=w1230) -> (x .and. y?=w1231:bool)
                        n492 = case shown="True" w1231 {
                          frame False {
                          }
                          frame True {
                            n493 = local read "%Out of Range"() -> (w1233:cluster{"Dev. X":bool, "Dev. Y":bool})
                            n494 = local read "Out of Range?"() -> (w1237:cluster{"Dev. X":bool, "Dev. Y":bool})
                            n495 = And(x="use Avg Out of Range?", y=w1237) -> (x .and. y?=w1236:cluster{"Dev. X":bool, "Dev. Y":bool})
                            n496 = And(x="use % Out of Range", y=w1233) -> (x .and. y?=w1239:cluster{"Dev. X":bool, "Dev. Y":bool})
                            n497 = Compound Arithmetic op=OR(w1236, w1239) -> (w1241:cluster{"Dev. X":bool, "Dev. Y":bool})
                            n498 = Unbundle(w1241) -> ("Dev. X"=→"Move X":bool, "Dev. Y"=→"Move Y":bool)
                          }
                        }
                        n499 = local write "State"(9) -> ()
                      }
                      frame #12 {
                        # "Calculate required move parameters to correct beam pointing"
                        n500 = Unbundle By Name("Correction Parameters") -> ("Movement Type"=w1245:u16, "X"=w1243:sgl, "Y"=w1242:sgl)
                        n501 = local read "Corrective Move XY"() -> (w1248:T5)
                        n502 = local read "Avg Deviation"() -> (w1249:cluster{sgl, sgl})
                        n503 = local read "Move Y"() -> (w1250:bool)
                        n504 = local read "Move X"() -> (w1251:bool)
                        n505 = Unbundle(w1249) -> (w1253:sgl, w1252:sgl)
                        n506 = case shown="True" w1251 {
                          tunnel: w1253 -> [w1285 _]
                          tunnel: w1245 -> [w1284 _]
                          tunnel: w1248 -> [w1280 w1292]
                          tunnel: [w1281 w1292] -> w1247
                          tunnel: w1243 -> [w1275 _]
                          frame True {
                            n507 = case shown="1" w1284 {
                              tunnel: w1285 -> [_ w1289]
                              tunnel: [w1287 w1290] -> w1276
                              tunnel: w1275 -> [w1287 _]
                              frame 0, Default {
                              }
                              frame 1 {
                                n508 = local read "X calibration"() -> (w1291:cluster{dbl, dbl}[])
                                n509 = Negate(x=w1289) -> (-x=w1288:sgl)
                                n510 = call "FindNrSteps.vi"("X calibration"=w1291, "pixels"=w1288) -> ("NrSteps"=w1290:dbl)
                              }
                            }
                            n511 = Index Array(array=w1280, index=0) -> (element=w1282:T3)
                            n512 = Greater Or Equal To 0?(x=w1285) -> (x >= 0?=w1274:bool)
                            n513 = Absolute Value(x=w1276) -> (abs(x)=w1277:dbl)
                            n514 = Not(x=w1274) -> (.not. x?=w1286:bool)
                            n515 = Bundle By Name(cluster=w1282, "Left"=w1274, "Right"=w1286, "APulses X"=w1277) -> (w1279:T3)
                            n516 = Replace Array Subset(array=w1280, new element=w1279, index=0) -> (w1281:T5)
                          }
                          frame False {
                          }
                        }
                        n517 = case shown="True" w1250 {
                          tunnel: w1252 -> [w1267 _]
                          tunnel: w1245 -> [w1266 _]
                          tunnel: w1247 -> [w1262 w1273]
                          tunnel: [w1261 w1273] -> w1246
                          tunnel: w1242 -> [w1257 _]
                          frame True {
                            n518 = case shown="1" w1266 {
                              tunnel: w1267 -> [_ w1270]
                              tunnel: [w1268 w1271] -> w1259
                              tunnel: w1257 -> [w1268 _]
                              frame 0, Default {
                              }
                              frame 1 {
                                n519 = local read "Y calibration"() -> (w1272:cluster{dbl, dbl}[])
                                n520 = Negate(x=w1270) -> (-x=w1269:sgl)
                                n521 = call "FindNrSteps.vi"("X calibration"=w1272, "pixels"=w1269) -> ("NrSteps"=w1271:dbl)
                              }
                            }
                            n522 = Absolute Value(x=w1259) -> (abs(x)=w1258:dbl)
                            n523 = Greater Or Equal To 0?(x=w1267) -> (x >= 0?=w1255:bool)
                            n524 = Not(x=w1255) -> (.not. x?=w1256:bool)
                            n525 = Index Array(array=w1262, index=1) -> (element=w1263:T3)
                            n526 = Bundle By Name(cluster=w1263, "Down"=w1256, "Up"=w1255, "APulses Y"=w1258) -> (w1260:T3)
                            n527 = Replace Array Subset(array=w1262, new element=w1260, index=1) -> (w1261:T5)
                          }
                          frame False {
                          }
                        }
                        n528 = local write "Corrective Move XY"(w1246) -> ()
                        n529 = local write "State"(10) -> ()
                      }
                      frame #13 {
                        # "Send Corrective Move command"
                        n530 = local read "Corrective Move XY"() -> (w1318:T5)
                        n531 = local read "last move time"() -> (w1316:u32)
                        n532 = Index Array(array=w1309, index=w1305) -> (element=w1310:T36)
                        n533 = Tick Count (ms)() -> (millisecond timer value=w1317:u32)
                        n534 = expression code="x*1000" "[ms/s]"("Min time between moves (s)") -> (w1313:u32)
                        n535 = for {
                          tunnel: w1318 -> [w1327] mode=indexing
                          shift-right: [w1321] -> w1293
                          shift-left: FALSE -> [w1322]
                          n536 = Unbundle By Name(w1327) -> ("Right"=w1326:bool, "Left"=w1325:bool, "Up"=w1324:bool, "Down"=w1323:bool, "StopButton"=w1320:bool)
                          n537 = Compound Arithmetic op=OR(w1322, w1326, w1325, w1324, w1323, w1320) -> (w1321:bool)
                        }
                        "conn req" <- w1293
                        n538 = Subtract(x=w1317, y=w1316) -> (x-y=w1315:u32)
                        n539 = Greater?(x=w1315, y=w1313) -> (0:w1312:bool)
                        n540 = local read "Calibrate"() -> (w1308:bool)
                        n541 = Not(x=w1308) -> (.not. x?=w1307:bool)
                        n542 = local read "Last Move"() -> (w1304:string[])
                        n543 = And(x=w1312, y=w1293) -> (x .and. y?=w1306:bool)
                        n544 = And(x=w1307, y=w1306) -> (x .and. y?=w1294:bool)
                        "will move" <- w1294
                        n545 = case shown="True" w1294 {
                          tunnel: w1310 -> [_ w1334]
                          tunnel: w1318 -> [_ w1337]
                          tunnel: w1305 -> [_ w1329]
                          frame False {
                          }
                          frame True {
                            n546 = Get Date/Time In Seconds() -> (seconds since 1Jan1904=w1333:timestamp)
                            n547 = local read "Last Move"() -> (w1331:string[])
                            n548 = Get Date/Time String(seconds (now)=w1333, want seconds? (F)=TRUE) -> (time string=w1330:string)  [unwired: 1 in, 1 out]
                            n549 = local read "ConnectArray"() -> (w1336:T7)
                            n550 = Replace Array Subset(array=w1331, new element=w1330, index=w1329) -> (w1328:string[])
                            n551 = local write "Last Move"(w1328) -> ()
                            n552 = Tick Count (ms)() -> (millisecond timer value=→"last move time":u32)
                            n553 = stacked-sequence {
                              tunnel: w1337 -> [w1345 _ _]
                              tunnel: w1336 -> [w1344 _ _]
                              tunnel: "webcam" ("client name") -> [w1343 _ _]
                              tunnel: w1334 -> [w1342 _ _]
                              frame #0 {
                                n554 = call "Send Move Command.vi"("ConnectArray IN"=w1344, "client name"=w1343, "CamConfig"=w1342, "Move XY"=w1345) -> ("ConnectArray Out"=w1341:T7, "TCPconnecCmd"=w1339:bool, "status"=w1340:string)
                                n555 = local write "ConnectArray"(w1341) -> ()
                                n556 = local write "TCPconnecCmd"(w1339) -> ()
                                n557 = local write "Status"(w1340) -> ()
                              }
                              frame #1 {
                                n558 = Wait (ms)(milliseconds to wait=u32 1000) -> ()  [unwired: 1 out]
                              }
                              frame #2 {
                                n559 = Tick Count (ms)() -> (millisecond timer value=w1348:u32)
                                n560 = while {
                                tunnel: w1348 -> [w1352]
                                tunnel: [w1349] -> w1347
                                i -> [w1361]
                                stop <- w1354 stop-if-true
                                n561 = Tick Count (ms)() -> (millisecond timer value=w1353:u32)
                                n562 = Subtract(x=w1353, y=w1352) -> (x-y=w1351:u32)
                                n563 = local read "MoveInProgress"() -> (w1356:bool)
                                n564 = Greater?(x=w1351, y=u32 10000) -> (0:w1349:bool)
                                n565 = local read "RunON/OFF"() -> (w1358:bool)
                                n566 = local read "restart"() -> (w1359:bool)
                                n567 = local read "stop"() -> (w1360:bool)
                                n568 = Wait (ms)(milliseconds to wait=u32 100) -> ()  [unwired: 1 out]
                                n569 = Not(x=w1356) -> (.not. x?=w1355:bool)
                                n570 = Not(x=w1358) -> (.not. x?=w1357:bool)
                                n571 = Compound Arithmetic op=OR(w1355, w1360, w1359, w1357, w1349) -> (w1354:bool)
                                "# loops waiting 4 move" <- w1361
                                }
                                "MoveInProgress 2" <- w1347
                              }
                            }
                          }
                        }
                        n572 = Index Array(array=w1304) -> (element #1=→"element":string, element #2=→"element 2":string, element #3=→"element 3":string, element #4=→"element 4":string, element #5=→"element 5":string, element #6=→"element 6":string, element #7=→"element 7":string, element #8=→"element 8":string, element #9=→"element 9":string)  [unwired: 9 in]
                        n573 = local write "State"(11) -> ()
                      }
                      frame #14 {
                        # "Statistics"
                        n574 = local read "Beam Detected"() -> (w1363:bool)
                        n575 = case shown="True" w1363 {
                          tunnel: w1365 -> [_ w1376]
                          tunnel: w1364 -> [_ w1375]
                          frame False {
                          }
                          frame True {
                            # "Save history"
                            n576 = local read "History XY Buffer"() -> (w1374:T14)
                            n577 = local read "Main processing loop i"() -> (w1372:i32)
                            n578 = Index Array(array=w1374, index (row)=w1375) -> (element=w1367:T17)  [unwired: 1 in]
                            n579 = Unbundle By Name(w1376) -> ("Center"=w1373:cluster{"X":sgl, "Y":sgl})
                            n580 = Equal To 0?(x=w1372) -> (x = 0?=w1371:bool)
                            n581 = call "Add point in History v2.vi"("History XY In"=w1367, "New Point"=w1373, "clear first (no:F)"=w1371, "chart length (points)"="History # of points") -> ("History XY Out"=w1368:T17)  [unwired: 4 in]
                            n582 = local read "History XY Buffer"() -> (w1369:T14)
                            n583 = call "Add Or Replace History Array.vi"("History XY Buffer In"=w1369, "History XY In"=w1368, "Index"=w1375, "# of points"="History # of points") -> ("History XY Buffer Out"=w1370:T14)  [unwired: 6 in]
                            n584 = local write "History XY Buffer"(w1370) -> ()
                          }
                        }
                      }
                      frame #15 {
                        # "Statistics"
                        n585 = local read "NewAvg"() -> (w1378:bool)
                        n586 = case shown="True" w1378 {
                          tunnel: w1377 -> [_ w1379]
                          frame False {
                          }
                          frame True {
                            # "Save data in buffers to display"
                            n587 = local read "ImgData Avg"() -> (w1387:T23)
                            n588 = local read "Centroid Avg Buffer"() -> (w1382:cluster{"X Centroid":sgl, "Y Centroid":sgl}[])
                            n589 = Unbundle By Name(w1387) -> ("Centroid Avg"=w1386:cluster{"X":sgl, "Y":sgl})
                            n590 = call-poly "Replace Or Add.vi"("Coord"=w1386, "Index"=w1379, "Coord Array In"=w1382) -> ("Coord Array Out"=w1380:cluster{"X":sgl, "Y":sgl}[])  [unwired: 8 in]
                            n591 = local write "Centroid Avg Buffer"(w1380) -> ()
                            n592 = local read "Avg Img Buffer"() -> (w1383:u8[][][])
                            n593 = local read "Avg Img"() -> (w1381:T1)
                            n594 = call "IMAQ ImageToArray"("Image"=w1381) -> ("Image Pixels (U8)"=w1385:u8[][])  [unwired: 2 in, 5 out]
                            n595 = call-poly "Replace Or Add.vi"("Img"=w1385, "Index"=w1379, "Img Array In"=w1383) -> ("Img Array Out"=w1384:u8[][][])  [unwired: 8 in]
                            n596 = local write "Avg Img Buffer"(w1384) -> ()
                          }
                        }
                      }
                      frame #16 {
                        # "Choose image to display"
                        n597 = local read "Fancy Display Options"() -> (w1398:T24)
                        n598 = local read "Output Img"() -> (w1404:T1)
                        n599 = local read "Display"() -> (w1393:T26)
                        n600 = local read "Thresh Img"() -> (w1401:T1)
                        n601 = local read "Avg Img"() -> (w1402:T1)
                        n602 = local read "Displayed Image"() -> (w1390:u8[][])
                        n603 = Unbundle By Name(w1393) -> ("Show Best Rect"=w1392:bool)
                        n604 = Build Array(w1404, w1402, w1401) -> (w1400:T1[])
                        n605 = Unbundle By Name(w1398) -> ("Use fancy display"=w1397:bool, "show acquired image"=w1396:bool, "Show Edges"=w1395:bool, "Show Full Ellipse"=w1391:bool, "Show Ellipses points"=w1394:bool)
                        n606 = Array Size(array=w1390) -> (size(s)=→"size(s)":i32[])
                        n607 = Index Array(array=w1400, index="Image Selector") -> (element=w1399:T1)
                        n608 = local write "State"(6) -> ()
                        n609 = call "IMAQ ImageToArray"("Image"=w1399) -> ("Image Pixels (U8)"=w1388:u8[][])  [unwired: 2 in, 5 out]
                        "Displayed Image" <- w1388
                        n610 = case shown="True" w1397 {
                          tunnel: w1388 -> [_ w1414]
                          tunnel: w1396 -> [_ w1428]
                          tunnel: w1395 -> [_ w1427]
                          tunnel: w1394 -> [_ w1426]
                          tunnel: w1392 -> [_ w1412]
                          tunnel: w1391 -> [_ w1416]
                          frame False {
                          }
                          frame True {
                            n611 = local read "Fancy Display"() -> (w1410:picture)
                            n612 = call <vilib>:"Flatten Pixmap.vi"("8-bit pixmap"=w1414) -> ("image data"=w1430:T44)  [unwired: 10 in]
                            n613 = call <vilib>:"Draw Rect.vi"("picture"=w1410, "rect"=T33 {"left"=0, "top"=0, "right"=800, "bottom"=600}, "fill?(F)"=TRUE, "color(black)"=u32 16777226) -> ("new picture"=w1407:picture)  [unwired: 5 in]
                            n614 = local read "Beam Detected"() -> (w1413:bool)
                            n615 = call <vilib>:"Draw Flattened Pixmap.vi"("image data"=w1430, "picture"=w1407) -> ("new picture"=w1429:picture)  [unwired: 7 in]
                            n616 = local read "RectFilter"() -> (w1422:T13)
                            n617 = Select(t=w1429, s=w1428, f=w1407) -> (s? t:f=w1424:picture)
                            n618 = Unbundle By Name(w1422) -> ("Left"=w1421:i32, "Top"=w1420:i32, "Right"=w1419:i32, "Bottom"=w1418:i32)
                            n619 = And(x=w1413, y=w1412) -> (x .and. y?=w1411:bool)
                            n620 = Bundle("Left"=w1421, "Top"=w1420, "Right"=w1419, "Bottom"=w1418) -> (w1417:T45)  [unwired: 1 in]
                            n621 = case shown="True" w1411 {
                              tunnel: w1424 -> [w1435 w1440]
                              tunnel: [w1435 w1439] -> w1423
                              tunnel: w1417 -> [_ w1438]
                              frame False {
                              }
                              frame True {
                                n622 = call <vilib>:"Draw Rect.vi"("picture"=w1440, "rect"=w1438, "color(black)"=u32 16323327, "pen"=T34 {"Width"=2, "Style"=enum."Solid"}) -> ("new picture"=w1439:picture)  [unwired: 5 in]
                              }
                            }
                            n623 = case shown="True" w1427 {
                              tunnel: w1423 -> [w1456 w1458]
                              tunnel: [w1456 w1457] -> w1425
                              frame False {
                              }
                              frame True {
                                n624 = local read "Ellipse edges"() -> (w1460:cluster{"X":sgl, "Y":sgl}[])
                                n625 = Index Array(array=w1460, index=0) -> (element=w1459:cluster{"X":sgl, "Y":sgl})
                                n626 = call <vilib>:"Move Pen.vi"("new position"=w1459, "picture"=w1458) -> ("new picture"=w1462:picture)  [unwired: 3 in]
                                n627 = for {
                                tunnel: w1460 -> [w1466] mode=indexing
                                shift-right: [w1464] -> w1457
                                shift-left: w1462 -> [w1463]
                                n628 = call <vilib>:"Draw Line.vi"("picture"=w1463, "end point"=w1466, "color(black)"=u32 4390888, "pen"=T35 {"Width"=4, "Style"=enum."Solid"}) -> ("new picture"=w1464:picture)  [unwired: 5 in]
                                }
                              }
                            }
                            n629 = case shown="True" w1426 {
                              tunnel: w1425 -> [w1441 w1443]
                              tunnel: [w1441 w1442] -> w1415
                              frame False {
                              }
                              frame True {
                                w1450 = T35 {"Width"=10, "Style"=enum."Solid"} ("pen")
                                w1451 = u32 3473194 ("color(black)")
                                n630 = local read "Ellipse"() -> (w1444:T10)
                                n631 = Unbundle By Name(w1444) -> ("Major Axis.Point 1"=w1448:cluster{"X":sgl, "Y":sgl})
                                n632 = Unbundle By Name(w1444) -> ("Major Axis.Point 2"=w1447:cluster{"X":sgl, "Y":sgl})
                                n633 = Unbundle By Name(w1444) -> ("Center"=w1449:cluster{"X":sgl, "Y":sgl})
                                n634 = Unbundle By Name(w1444) -> ("Minor Axis.Point 1"=w1446:cluster{"X":sgl, "Y":sgl})
                                n635 = Unbundle By Name(w1444) -> ("Minor Axis.Point 2"=w1445:cluster{"X":sgl, "Y":sgl})
                                n636 = call <vilib>:"Draw Point.vi"("picture"=w1443, "point(x,y)"=w1449, "color(black)"=w1451, "pen"=w1450) -> ("new picture"=w1455:picture)  [unwired: 5 in]
                                n637 = call <vilib>:"Draw Point.vi"("picture"=w1455, "point(x,y)"=w1448, "color(black)"=w1451, "pen"=w1450) -> ("new picture"=w1454:picture)  [unwired: 5 in]
                                n638 = call <vilib>:"Draw Point.vi"("picture"=w1454, "point(x,y)"=w1447, "color(black)"=w1451, "pen"=w1450) -> ("new picture"=w1453:picture)  [unwired: 5 in]
                                n639 = call <vilib>:"Draw Point.vi"("picture"=w1453, "point(x,y)"=w1446, "color(black)"=w1451, "pen"=w1450) -> ("new picture"=w1452:picture)  [unwired: 5 in]
                                n640 = call <vilib>:"Draw Point.vi"("picture"=w1452, "point(x,y)"=w1445, "color(black)"=w1451, "pen"=w1450) -> ("new picture"=w1442:picture)  [unwired: 5 in]
                              }
                            }
                            n641 = case shown="True" w1416 {
                              tunnel: w1415 -> [w1431 w1433]
                              frame False {
                                n642 = local write "Fancy Display"(w1431) -> ()
                              }
                              frame True {
                                n643 = local read "Ellipse"() -> (w1432:T10)
                                n644 = call "Draw Ellipse.vi"("picture"=w1433, "Ellipse"=w1432) -> ("new picture"=w1434:picture)  [unwired: 9 in]
                                n645 = local write "Fancy Display"(w1434) -> ()
                              }
                            }
                          }
                        }
                      }
                      frame #17 {
                        n646 = local read "LoopMode"() -> (w1470:bool)
                        n647 = case shown="False" w1470 {
                          tunnel: w1468 -> [w1471 _]
                          frame False {
                            # "Display croos hairs of Detection ROI"
                            # "Accumulate statistics on whether beam centroid  is within specified range of target"
                            n648 = local read "ImgData Avg"() -> (w1488:T23)
                            n649 = Unbundle By Name("Target Area  Display") -> ("Show Target Reached"=w1490:bool)
                            n650 = Unbundle By Name("Target Area  Display") -> ("Show Init Correction"=w1489:bool)
                            n651 = Unbundle By Name("Target Area  Display") -> ("Show Variance"=w1491:bool)
                            n652 = local read "ImgDataArray"() -> (w1487:T15)
                            n653 = Unbundle By Name(w1488) -> ("Centroid Avg"=w1486:cluster{"X":sgl, "Y":sgl})
                            n654 = for {
                              tunnel: w1487 -> [w1525] mode=indexing
                              tunnel: [w1528] -> w1518 mode=indexing
                              tunnel: [w1527] -> w1517 mode=indexing
                              tunnel: w1486 -> [w1523]
                              n655 = Unbundle By Name(w1525) -> ("Center"=w1524:cluster{"X":sgl, "Y":sgl})
                              n656 = Subtract(x=w1524, y=w1523) -> (x-y=w1526:cluster{"X":sgl, "Y":sgl})
                              n657 = Absolute Value(x=w1526) -> (abs(x)=w1522:cluster{"X":sgl, "Y":sgl})
                              n658 = Unbundle(w1522) -> ("X"=w1528:sgl, "Y"=w1527:sgl)
                            }
                            n659 = Select(t=u32 16711680 ("Color"), s=w1491, f=u32 16777216 ("Color")) -> (s? t:f=w1503:u32)
                            n660 = Select(t=u32 16776704 ("Color"), s=w1490, f=u32 16777216 ("Color")) -> (s? t:f=w1496:u32)
                            n661 = Select(t=u32 3381759 ("Color"), s=w1489, f=u32 16777216 ("Color")) -> (s? t:f=w1507:u32)
                            n662 = property on="Target Area" class="XYGraph (strict)"("Active Plot"=u32 1, "Plot.Fill/Pt. Color"=w1496) -> ()  [unwired: 2 in, 2 out]
                            n663 = property on="Target Area" class="XYGraph (strict)"("Active Plot"=u32 0, "Plot.Plot Color"=w1503) -> ()  [unwired: 2 in, 2 out]
                            n664 = property on="Target Area" class="XYGraph (strict)"("Active Plot"=u32 2, "Plot.Plot Color"=w1507) -> ()  [unwired: 2 in, 2 out]
                            n665 = local read "Region of Interest"() -> (w1472:i32[])
                            n666 = call <vilib>:"Std Deviation and Variance.vi"("X"=w1518) -> ("mean"=w1499:dbl)  [unwired: 1 in, 2 out]
                            n667 = call <vilib>:"Std Deviation and Variance.vi"("X"=w1517) -> ("mean"=w1498:dbl)  [unwired: 1 in, 2 out]
                            n668 = Bundle("mean"=w1499, "mean"=w1498) -> (w1485:cluster{"mean":dbl, "mean":dbl})  [unwired: 1 out]
                            "Avg Variation" <- w1485
                            n669 = local read "DeviationArray"() -> (w1516:cluster{"X Centroid":sgl, "Y Centroid":sgl}[])
                            n670 = call-poly "Add ROI Offset.vi"("Region of Interest"=w1472, "RectFilter In"=w1471) -> ("RectFilter Out"=w1473:T13)  [unwired: 3 in]
                            n671 = Unbundle By Name(w1473) -> ("Left"=w1479:i32, "Top"=w1478:i32, "Right"=w1476:i32, "Bottom"=w1475:i32)
                            n672 = for {
                              tunnel: w1516 -> [w1521] mode=indexing
                              tunnel: [w1520] -> w1515 mode=indexing
                              tunnel: [w1519] -> w1514 mode=indexing
                              n673 = Unbundle(w1521) -> ("X Centroid"=w1520:sgl, "Y Centroid"=w1519:sgl)
                            }
                            n674 = local read "Deviation"() -> (w1497:cluster{"Dev. X":sgl, "Dev. Y":sgl})
                            n675 = Divide(x="Initiate Correction Range", y=sgl 100.0) -> (x/y=w1484:sgl)
                            n676 = call "ellipse graph.vi"("# of points"=100, "Avg Variation"=w1485, "Center"=w1497) -> ("ellipse graph"=w1508:cluster{dbl[], dbl[]})  [unwired: 1 in, 5 out]
                            n677 = Bundle("Right"=w1476, "Bottom"=w1475) -> (w1474:cluster{"Right":i32, "Bottom":i32})  [unwired: 1 in]
                            n678 = Bundle("Left"=w1479, "Top"=w1478) -> (w1477:cluster{"Left":i32, "Top":i32})  [unwired: 1 in]
                            n679 = call "circle graph.vi"("# of points"=100, "Radius"=w1484) -> ("circle graph"=w1482:cluster{dbl[], dbl[]})  [unwired: 7 out]
                            n680 = Bundle(w1515, w1514) -> (w1510:cluster{sgl[], sgl[]})  [unwired: 1 out]
                            n681 = Build Array(w1482, w1510, w1508) -> (→"Target Area":cluster{dbl[], dbl[]}[])
                            n682 = property on="Displayed Image" class="IntGraph (strict)"("Active Cursor"=u32 6, "Cursor.Cursor Position"=w1477, "Active Cursor"=u32 7, "Cursor.Cursor Position"=w1474) -> ()  [unwired: 2 in, 2 out]
                          }
                          frame True {
                          }
                        }
                        n683 = local write "State"(8) -> ()
                      }
                      frame #18 {
                        # "Target Area"
                        # "overlay cross-hairs on image at centroid and target locations"
                        # "X and Y profile"
                        # "Display"
                        # "cursor position"
                        # "target"
                        # "centroid avg"
                        n684 = local read "Display Current"() -> (w1552:bool)
                        n685 = case shown="True" w1552 {
                          tunnel: [w1605 w1612] -> w1584
                          tunnel: [w1609 w1611] -> w1548
                          tunnel: [w1606 w1610] -> w1569
                          tunnel: w1547 -> [w1608 _]
                          frame False {
                            n686 = local read "Image Selector"() -> (w1609:u16)
                            n687 = Index Array(array=w1608, index=w1609) -> (element=w1607:T36)
                            n688 = Unbundle By Name(w1607) -> ("CorrectConfig Cluster.Target"=w1606:cluster{"X Target":sgl, "Y Target":sgl}, "CorrectConfig Cluster.Region of Interest"=w1605:i32[])
                          }
                          frame True {
                            n689 = local read "USB cameras Indic"() -> (w1611:i32)
                            n690 = local read "Region of Interest"() -> (w1612:i32[])
                            n691 = local read "Target"() -> (w1610:cluster{"X Target":sgl, "Y Target":sgl})
                          }
                        }
                        n692 = local read "Centroid Avg Buffer"() -> (w1562:cluster{"X Centroid":sgl, "Y Centroid":sgl}[])
                        n693 = local read "History XY Buffer"() -> (w1531:T14)
                        n694 = local read "Img Size"() -> (w1551:i32[])
                        n695 = Not Equal?(x=w1584, y=i32[] [0, 0, 0, 0] ("Region of Interest")) -> (x != y?=w1550:bool)
                        n696 = Index Array(array=w1531, index (col)=0 ("disabled index (col)")) -> (element=→"history last shots":T17)  [unwired: 1 in]
                        n697 = Select(t=w1584, s=w1550, f=w1551) -> (s? t:f=w1549:i32[])
                        n698 = property on="Displayed Image" class="IntGraph (strict)"("Active Cursor"=u32 0) -> ("Cursor.Cursor Position"=w1582:T40)  [unwired: 2 in, 2 out]
                        n699 = property on="Displayed Image" class="IntGraph (strict)"("Active Cursor"=u32 1, "Cursor.Cursor Position"=w1569) -> ()  [unwired: 2 in, 2 out]
                        n700 = Index Array(array=w1562, index=w1548) -> (element=w1553:cluster{"X Centroid":sgl, "Y Centroid":sgl})
                        n701 = case shown="True" "set scales" {
                          tunnel: w1549 -> [_ w1598]
                          frame False {
                          }
                          frame True {
                            n702 = for {
                              tunnel: w1598 -> [w1599] mode=indexing
                              i -> [w1600]
                              # "set scales"
                              n703 = case shown="3" w1600 {
                                tunnel: w1599 -> [w1601 w1602 w1603 w1604 _]
                                frame 0 {
                                n704 = property on="Displayed Image" class="IntGraph (strict)"("XScale.Offset"=w1601, "XScale.Minimum"=w1601) -> ()  [unwired: 2 in, 2 out]
                                n705 = property on="X Intensity" class="WFGraph (strict)"("XScale.Offset"=w1601, "XScale.Minimum"=w1601) -> ()  [unwired: 2 in, 2 out]
                                }
                                frame 1 {
                                n706 = property on="Displayed Image" class="IntGraph (strict)"("YScale.Offset"=w1602, "YScale.Minimum"=w1602) -> ()  [unwired: 2 in, 2 out]
                                n707 = property on="Y Intensity" class="WFGraph (strict)"("XScale.Offset"=w1602, "XScale.Minimum"=w1602) -> ()  [unwired: 2 in, 2 out]
                                }
                                frame 2 {
                                n708 = property on="Displayed Image" class="IntGraph (strict)"("XScale.Maximum"=w1603) -> ()  [unwired: 2 in, 2 out]
                                n709 = property on="X Intensity" class="WFGraph (strict)"("XScale.Maximum"=w1603) -> ()  [unwired: 2 in, 2 out]
                                }
                                frame 3 {
                                n710 = property on="Displayed Image" class="IntGraph (strict)"("YScale.Maximum"=w1604) -> ()  [unwired: 2 in, 2 out]
                                n711 = property on="Y Intensity" class="WFGraph (strict)"("XScale.Maximum"=w1604) -> ()  [unwired: 2 in, 2 out]
                                }
                                frame 4, Default {
                                }
                              }
                            }
                          }
                        }
                        n712 = for {
                          tunnel: w1531 -> [w1593] mode=indexing
                          tunnel: [w1588] -> _ mode=indexing
                          tunnel: [w1587] -> _ mode=indexing
                          tunnel: [w1586] -> w1541 mode=indexing
                          n713 = call "History remove zeros.vi"("History XY In"=w1593) -> ("History XY Out"=w1592:T17)  [unwired: 2 in]
                          n714 = for {
                            tunnel: w1592 -> [w1597] mode=indexing
                            tunnel: [w1596] -> w1590 mode=indexing
                            tunnel: [w1595] -> w1591 mode=indexing
                            tunnel: [w1594] -> w1589 mode=indexing
                            n715 = Unbundle(w1597) -> ("seconds since 1Jan1904"=w1596:timestamp, "number: 0 to 1"=w1595:dbl, "number: 0 to 1"=w1594:dbl)
                          }
                          n716 = Bundle(w1590, w1591) -> (w1588:cluster{timestamp[], dbl[]})  [unwired: 1 in]
                          n717 = Bundle(w1590, w1589) -> (w1587:cluster{timestamp[], dbl[]})  [unwired: 1 in]
                          n718 = Build Array(w1588, w1587) -> (w1586:cluster{timestamp[], dbl[]}[])
                        }
                        n719 = local read "Initiate Correction Range"() -> (w1555:i16)
                        n720 = property on="Displayed Image" class="IntGraph (strict)"("Active Cursor"=u32 2, "Cursor.Cursor Position"=w1553) -> ()  [unwired: 2 in, 2 out]
                        n721 = Unbundle By Name(w1582) -> ("Cursor Y"=w1581:dbl, "Cursor X"=w1578:dbl)
                        n722 = Index Array(array=w1584, index #1=0 ("index"), index #2=1 ("index")) -> (element #1=w1571:i32, element #2=w1570:i32)
                        n723 = Unbundle By Name(w1569) -> ("X Target"=w1565:sgl, "Y Target"=w1564:sgl)
                        n724 = local read "Displayed Image"() -> (w1544:u8[][])
                        n725 = Subtract(x=w1578, y=w1571) -> (x-y=w1574:dbl)
                        n726 = Subtract(x=w1581, y=w1570) -> (x-y=w1575:dbl)
                        n727 = Divide(x=w1555, y=sgl 100.0) -> (x/y=w1556:sgl)
                        n728 = local read "History XY Buffer"() -> (w1542:T14)
                        n729 = Multiply(x=w1553, y=w1556) -> (x*y=w1561:cluster{"X Centroid":sgl, "Y Centroid":sgl})
                        n730 = property on="History Display" class="XYGraph (strict)"("Active Cursor"=u32 0, "Cursor.Cursor Y"=w1565, "Active Cursor"=u32 1, "Cursor.Cursor Y"=w1564) -> ()  [unwired: 2 in, 2 out]
                        n731 = Index Array(array=w1541) -> (element #1=→"History Display 2":cluster{timestamp[], dbl[]}[], element #2=→"History Display 3":cluster{timestamp[], dbl[]}[], element #3=→"History Display 4":cluster{timestamp[], dbl[]}[], element #4=→"History Display 5":cluster{timestamp[], dbl[]}[], element #5=→"History Display 6":cluster{timestamp[], dbl[]}[], element #6=→"History Display 7":cluster{timestamp[], dbl[]}[], element #7=→"History Display 8":cluster{timestamp[], dbl[]}[], element #8=→"History Display 9":cluster{timestamp[], dbl[]}[], element #9=→"History Display 10":cluster{timestamp[], dbl[]}[])  [unwired: 18 in]
                        n732 = Index Array(array=w1544, index (row)=w1575) -> (element=→"X Intensity":u8[])  [unwired: 1 in]
                        n733 = Delete From Array(array=w1544, length=1, index (col)=w1574) -> (deleted portion=w1577:u8[][])  [unwired: 1 in, 1 out]
                        n734 = call "Rectangle Overlay for 2 Cursors.vi"("Radius"=w1561, "Coord"=w1569) -> ("Right Bottom"=w1559:cluster{dbl, dbl}, "Left Top"=w1560:cluster{dbl, dbl})  [unwired: 2 in, 6 out]
                        n735 = Transpose 2D Array(2D array=w1577) -> (transposed array=→"Y Intensity":u8[][])
                        n736 = Index Array(array=w1542, index (row)=w1548) -> (element=w1546:T17)  [unwired: 1 in]
                        n737 = call "History remove zeros.vi"("History XY In"=w1546) -> ("History XY Out"=→"History Display":T17)  [unwired: 2 in]
                        n738 = property on="Displayed Image" class="IntGraph (strict)"("Active Cursor"=u32 4, "Cursor.Cursor Position"=w1560, "Active Cursor"=u32 5, "Cursor.Cursor Position"=w1559) -> ()  [unwired: 2 in, 2 out]
                      }
                      frame #19 {
                        n739 = local read "MoveInProgressTimeIN"() -> (w1620:u32)
                        n740 = local read "LoopMode"() -> (w1628:bool)
                        n741 = local read "NewAvg"() -> (w1625:bool)
                        n742 = local read "start"() -> (w1622:u32)
                        n743 = Tick Count (ms)() -> (millisecond timer value=w1621:u32)
                        n744 = Wait (ms)(milliseconds to wait="milliseconds to wait") -> ()  [unwired: 1 out]
                        n745 = Subtract(x=w1621, y=w1622) -> (x-y=→"one loop":u32)
                        n746 = case shown="True" w1628 {
                          tunnel: [w1649 w1663] -> w1624
                          tunnel: w1616 -> [w1646 w1661]
                          tunnel: w1613 -> [w1639 w1652]
                          frame False {
                            # "Manual mode"
                            n747 = local read "Auto Detect Param"() -> (w1643:bool)
                            n748 = local read "error CamS"() -> (w1650:errorcluster)
                            n749 = local read "RunON/OFF"() -> (w1651:bool)
                            n750 = Greater Or Equal?(x=w1646, y=20) -> (x >= y?=w1642:bool)
                            n751 = Implies(1:w1642, 2:w1643) -> (0:w1641:bool)
                            n752 = Unbundle By Name(w1650) -> ("status"=w1647:bool)
                            n753 = Not(x=w1641) -> (.not. x?=w1640:bool)
                            n754 = Not(x=w1651) -> (.not. x?=w1648:bool)
                            n755 = local write "Auto Detect Param"(w1640) -> ()
                            n756 = And(x=w1643, y=w1642) -> (x .and. y?=w1644:bool)
                            n757 = Compound Arithmetic op=OR(w1639, w1648, w1647, w1644) -> (w1649:bool)
                          }
                          frame True {
                            # "Automatic mode"
                            n758 = local read "OpenTime"() -> (w1656:u32)
                            n759 = local read "# imgs to avg"() -> (w1662:i32)
                            n760 = Tick Count (ms)() -> (millisecond timer value=w1657:u32)
                            n761 = Subtract(x=w1657, y=w1656) -> (x-y=w1655:u32)
                            n762 = local read "NewAvg"() -> (w1664:bool)
                            n763 = Multiply(x=w1662, y=10) -> (x*y=w1660:i32)
                            n764 = Greater?(x=w1655, y="Auto Time Out (ms)") -> (0:w1654:bool)
                            n765 = Greater?(x=w1661, y=w1660) -> (0:w1659:bool)
                            n766 = Compound Arithmetic op=OR(w1652, w1664, w1659, w1654) -> (w1663:bool)
                          }
                        }
                        n767 = case shown="True" w1625 {
                          frame False {
                          }
                          frame True {
                            # "re-intialize for new average"
                            n768 = Initialize Array(T31 {"X Intensity"=[], "Y Intensity"=[], "Max Intensity"=0, "Center"={"X"=0, "Y"=0}, "Radius"={"Rx"=0, "Ry"=0}} ("ImgData"), 0 ("dimension size")) -> (w1637:T37)
                            n769 = Initialize Array(cluster{"Width (x)":sgl, "Height (y)":sgl} {"Width (x)"=0.0, "Height (y)"=0.0} ("SpotSizeAvg"), 0 ("dimension size")) -> (w1634:cluster{"Width (x)":sgl, "Height (y)":sgl}[])
                            n770 = local write "ImgDataArray"(w1637) -> ()
                            n771 = local write "DeviationArray"(w1634) -> ()
                          }
                        }
                        n772 = Subtract(x=w1621, y=w1620) -> (x-y=w1619:u32)
                        n773 = Greater?(x=w1619, y=u32 10000) -> (0:w1617:bool)
                        n774 = case shown="True" w1617 {
                          frame False {
                          }
                          frame True {
                            # "reset InProgress if  stuck for more \nthan 10s."
                            n775 = Initialize Array("", 0 ("dimension size")) -> (w1632:string[])
                            n776 = local write "InProgress"(w1632) -> ()
                          }
                        }
                        n777 = case shown="True" w1624 {
                          tunnel: w1627 -> [_ w1668]
                          tunnel: w1615 -> [w1665 w1667]
                          tunnel: [w1665 w1666] -> w1614
                          frame False {
                          }
                          frame True {
                            n778 = stacked-sequence {
                              tunnel: w1668 -> [w1675 _]
                              tunnel: w1667 -> [w1685 _]
                              tunnel: [w1672 _] -> w1666
                              frame #0 {
                                # "save data"
                                n779 = local read "Correction Parameters"() -> (w1684:cluster{"X":sgl, "Y":sgl, "Movement Type":u16})
                                n780 = local read "Background Path"() -> (w1677:path)
                                n781 = local read "Detection Parameters"() -> (w1680:T21)
                                n782 = local read "X calibration"() -> (w1671:cluster{dbl, dbl}[])
                                n783 = local read "Y calibration"() -> (w1670:cluster{dbl, dbl}[])
                                n784 = local read "Region of Interest"() -> (w1683:i32[])
                                n785 = local read "Reference Path"() -> (w1676:path)
                                n786 = local read "Target"() -> (w1682:cluster{"X Target":sgl, "Y Target":sgl})
                                n787 = local read "Reverse"() -> (w1681:cluster{"Reverse X":bool, "Reverse Y":bool})
                                n788 = case shown="True" FALSE {
                                tunnel: w1675 -> [_ w1686]
                                frame False {
                                }
                                frame True {
                                n789 = local read "Feedback"() -> (w1687:bool)
                                n790 = local read "Corr"() -> (w1689:bool[])
                                n791 = Replace Array Subset(array=w1689, new element=w1687, index=w1686) -> (w1688:bool[])
                                n792 = local write "Corr"(w1688) -> ()
                                }
                                }
                                n793 = Index Array(array=w1685, index=w1675) -> (element=w1679:T36)
                                n794 = local read "Mirrors"() -> (w1674:u8[])
                                n795 = Bundle By Name(cluster=w1679, "CorrectConfig Cluster.Detection Parameters"=w1680, "CorrectConfig Cluster.Reverse"=w1681, "CorrectConfig Cluster.Target"=w1682, "CorrectConfig Cluster.Region of Interest"=w1683, "CorrectConfig Cluster.Correction Parameters"=w1684, "CorrectConfig Cluster.Background Path"=w1677, "CorrectConfig Cluster.Reference Path"=w1676, "CorrectConfig Cluster.XCalibration"=w1671, "CorrectConfig Cluster.YCalibration"=w1670) -> (w1678:T36)
                                n796 = Replace Array Subset(array=w1685, new element=w1678, index=w1675) -> (w1673:T9)
                                n797 = for {
                                tunnel: w1674 -> [w1694] mode=indexing
                                tunnel: w1673 -> [w1693] mode=indexing
                                tunnel: [w1690] -> w1672 mode=indexing
                                n798 = local read "DeviceList"() -> (w1695:T16)
                                n799 = call "NumberToDeviceID-v2.vi"("device raw"=w1694, "DeviceList"=w1695) -> ("DeviceID"=w1691:T32, "Name"=w1692:string)  [unwired: 5 in, 3 out]
                                n800 = Bundle By Name(cluster=w1693, "Name"=w1692, "DeviceID"=w1691) -> (w1690:T36)
                                }
                              }
                              frame #1 {
                                # "Dispose buffer"
                                n801 = local read "Img Buffer"() -> (w1698:T1[])
                                n802 = local read "error CamS"() -> (w1697:errorcluster)
                                n803 = local read "OpenTime"() -> (w1700:u32)
                                n804 = Tick Count (ms)() -> (millisecond timer value=w1699:u32)
                                "Switch in" <- w1699
                                n805 = call "IMAQ Dispose Buffer.vi"("error in"=w1697, "Img Buffer In"=w1698) -> ("error out"=w1696:errorcluster)  [unwired: 1 in]
                                n806 = Subtract(x=w1699, y=w1700) -> (x-y=→"AcqTime":u32)
                                n807 = local write "error CamS"(w1696) -> ()
                              }
                            }
                          }
                        }
                        n808 = local write "State"(12) -> ()
                      }
                    }
                    "Main processing loop i" <- w736
                  }
                  n809 = local write "CamConfigArray"(w728) -> ()
                }
              }
            }
            n810 = for {
              tunnel: w404 -> [w481] mode=indexing
              tunnel: [w480] -> w403 mode=indexing
              tunnel: [w479] -> w402 mode=indexing
              n811 = Unbundle By Name(w481) -> ("ImageServer"=w482:cluster{"IPAddress":string, "Port":i32})
              n812 = Unbundle By Name(w482) -> ("IPAddress"=w480:string, "Port"=w479:i32)
            }
            "Image IPs" <- w403
            "Image Ports" <- w402
            n813 = while {
              tunnel: w405 -> [w483]
              stop <- w484 stop-if-true
              n814 = local read "restart"() -> (w484:bool)
              n815 = event shown="[15] \"Reset ROI\": Value Change" {
                selector: _ -> [_ _ _ _ _ _ _ _ _ _ _ _ _ _ _ _ _ _ _ _ _ _]
                dyn-events: _ -> [_ _ _ _ _ _ _ _ _ _ _ _ _ _ _ _ _ _ _ _ _ _]
                timeout: 500 -> [_ _ _ _ _ _ _ _ _ _ _ _ _ _ _ _ _ _ _ _ _ _]
                tunnel: w483 -> [_ _ _ _ _ _ w560 _ _ _ _ _ _ _ _ _ _ _ _ _ _ _]
                event Timeout {
                  n816 = event-data() -> ()  [unwired: 3 out]
                }
                event "MoveInProgress": Value Change {
                  n817 = event-data() -> ("OldVal"=w487:bool, "NewVal"=w486:bool)  [unwired: 1 out]
                  n818 = Not(x=w487) -> (.not. x?=w488:bool)
                  n819 = And(x=w488, y=w486) -> (x .and. y?=w489:bool)
                  n820 = case shown="False" w489 {
                    frame False {
                    }
                    frame True {
                      n821 = Tick Count (ms)() -> (millisecond timer value=→"MoveInProgressTimeIN":u32)
                    }
                  }
                }
                event "Calibrate": Value Change {
                  n822 = event-data() -> ("NewVal"=w491:bool)  [unwired: 2 out]
                  n823 = case shown="False" w491 {
                    frame False {
                      n824 = local read "X calibration"() -> (w504:cluster{dbl, dbl}[])
                      n825 = local read "Y calibration"() -> (w508:cluster{dbl, dbl}[])
                      n826 = Array Size(array=w504) -> (size(s)=w506:i32)
                      n827 = Array Size(array=w508) -> (size(s)=w510:i32)
                      n828 = for {
                        tunnel: w508 -> [w523] mode=indexing
                        tunnel: w504 -> [w522] mode=indexing
                        tunnel: [w521] -> w494 mode=indexing
                        tunnel: [w520] -> w502 mode=indexing
                        tunnel: [w519] -> w495 mode=indexing
                        tunnel: [w518] -> w498 mode=indexing
                        n829 = Unbundle(w522) -> (w521:dbl, w520:dbl)
                        n830 = Unbundle(w523) -> (w519:dbl, w518:dbl)
                      }
                      n831 = Decrement(x=w506) -> (x-1=w507:i32)
                      n832 = Decrement(x=w510) -> (x-1=w511:i32)
                      n833 = Initialize Array(5.0 ("element"), w507) -> (w503:dbl[])
                      n834 = Initialize Array(5.0 ("element"), w511) -> (w499:dbl[])
                      n835 = call <vilib>:"Cubic Spline Fit.vi"("Y"=w502, "X"=w494, "balance parameter"=-1.0, "Smoothness"=w503) -> ("Best Cubic Spline Fit"=w497:dbl[])  [unwired: 10 in, 1 out]
                      n836 = call <vilib>:"Cubic Spline Fit.vi"("Y"=w498, "X"=w495, "balance parameter"=-1.0, "Smoothness"=w499) -> ("Best Cubic Spline Fit"=w496:dbl[])  [unwired: 10 in, 1 out]
                      n837 = for {
                        tunnel: w497 -> [w517] mode=indexing
                        tunnel: w496 -> [w516] mode=indexing
                        tunnel: w495 -> [w515] mode=indexing
                        tunnel: w494 -> [w514] mode=indexing
                        tunnel: [w513] -> w493 mode=indexing
                        tunnel: [w512] -> w492 mode=indexing
                        n838 = Bundle(w515, "Numeric"=w516) -> (w512:cluster{dbl, "Numeric":dbl})  [unwired: 1 in]
                        n839 = Bundle(w514, "Numeric"=w517) -> (w513:cluster{dbl, "Numeric":dbl})  [unwired: 1 in]
                      }
                      n840 = local write "X calibration"(w493) -> ()
                      n841 = local write "Y calibration"(w492) -> ()
                    }
                    frame True {
                      w526 = cluster{dbl, dbl}[] [{0.0, 0.0}] ("X calibration")
                      n842 = local write "X calibration"(w526) -> ()
                      n843 = local write "Y calibration"(w526) -> ()
                      n844 = local read "ImgData Avg"() -> (w525:T23)
                      n845 = Unbundle By Name(w525) -> ("Centroid Avg"=w524:cluster{"X":sgl, "Y":sgl})
                      n846 = local read "BestRects Cluster"() -> (w528:T12)
                      n847 = Bundle By Name(cluster=w528, "PreviousCenter"=w524, "CurrentCenter"=w524) -> (w527:T12)
                      n848 = local write "BestRects Cluster"(w527) -> ()
                    }
                  }
                }
                event "Add Camera": Mouse Up {
                  n849 = event-data() -> ()  [unwired: 2 out]
                  n850 = local read "DeviceNames"() -> (w529:string[])
                  n851 = call "newCameraPrompt.vi"("DeviceList"=w529) -> ("valid"=w532:bool, "ontrakOut"=w531:i32, "DeviceOut"=w530:string)  [unwired: 8 in]
                  n852 = case shown="True" w532 {
                    tunnel: w531 -> [_ _]
                    tunnel: w530 -> [_ w534]
                    frame False {
                    }
                    frame True {
                      n853 = local read "DeviceNames"() -> (w537:string[])
                      n854 = local write "Add Camera"(FALSE ("Add Camera")) -> ()
                      n855 = local read "AddCameraCluster"() -> (w536:T8)
                      n856 = Search 1D Array(1D array=w537, element=w534) -> (index of element=w538:i32)  [unwired: 1 in]
                      n857 = Bundle By Name(cluster=w536, "Add?"=TRUE, "Device Name"=w534) -> (w533:T8)
                      n858 = local read "Mirrors"() -> (w539:u8[])
                      n859 = Array Size(array=w539) -> (size(s)=w540:i32)
                      n860 = Insert Into Array(array=w539, new element=w538) -> ()  [unwired: 1 in, 1 out]
                      n861 = local write "AddCameraCluster"(w533) -> ()
                      n862 = Increment(x=w540) -> (x+1=w541:i32)
                      n863 = local write "# of cams"(w541) -> ()
                      n864 = property on="Mirrors" class="Arr (strict)"("Number of Rows"=w541) -> ()  [unwired: 2 in, 2 out]
                    }
                  }
                }
                event "Remove Camera": Mouse Up {
                  n865 = event-data() -> ()  [unwired: 2 out]
                  n866 = local read "CamConfigArray"() -> (w544:T9)
                  n867 = local read "Mirrors"() -> (w552:u8[])
                  n868 = property on="USB cameras" class="LstBox (strict)"() -> ("Value"=w545:i32)  [unwired: 2 in, 2 out]
                  n869 = local read "Mirrors"() -> (w554:u8[])
                  n870 = Delete From Array(array=w554, length=1, index=w545) -> (array with subset deleted=w546:u8[])  [unwired: 1 out]
                  n871 = Delete From Array(array=w544, length=1, index=w545) -> (array with subset deleted=w543:T9)  [unwired: 1 out]
                  n872 = Delete From Array(array=w552, length=1, index=w545) -> (array with subset deleted=w551:u8[])  [unwired: 1 out]
                  n873 = local write "Mirrors"(w551) -> ()
                  n874 = local write "CamConfigArray"(w543) -> ()
                  n875 = local write "Mirrors"(w546) -> ()
                  n876 = for {
                    tunnel: [w557] -> w548 mode=indexing
                    tunnel: w546 -> [w556] mode=indexing
                    n877 = local read "DeviceList"() -> (w555:T16)
                    n878 = call "NumberToDeviceID-v2.vi"("device raw"=w556, "DeviceList"=w555) -> ("Name"=w557:string)  [unwired: 5 in, 4 out]
                  }
                  n879 = local write "Remove Camera"(FALSE ("RunON/OFF")) -> ()
                  n880 = property on="USB cameras" class="LstBox (strict)"("Item Names"=w548) -> ()  [unwired: 2 in, 2 out]
                }
                event "USB cameras", "Acquisition Parameters", "Acquisition Parameters dx": Value Change {
                  n881 = event-data() -> ()  [unwired: 7 out]
                  n882 = stacked-sequence {
                    frame #0 {
                      # "stop the main loop"
                      n883 = local write "RunON/OFF"(FALSE ("RunON/OFF")) -> ()
                    }
                    frame #1 {
                      # "run the main loop with the new camera"
                      n884 = local write "RunON/OFF"(TRUE ("RunON/OFF")) -> ()
                    }
                  }
                }
                event "LoopMode": Value Change {
                  n885 = event-data() -> ("NewVal"=w564:bool)  [unwired: 1 out]
                  n886 = local write "RunON/OFF"(w564) -> ()
                  n887 = Not(x=w564) -> (.not. x?=w565:bool)
                  n888 = local read "# of cams"() -> (w562:i32)
                  n889 = property on="USB cameras Indic" class="LstBox (strict)"("Visible"=w564) -> ()  [unwired: 2 in, 2 out]
                  n890 = call-poly "Replace Or Add.vi"("String"="Acquired Image" ("new element/subarray"), "Index"=w562, "Array In"=w560) -> ()  [unwired: 8 in, 1 out]
                  n891 = property on="Manual Move" class="Clust"("Visible"=w565) -> ()  [unwired: 2 in, 2 out]
                  n892 = local read "Image Selector"() -> (w561:u16)
                  n893 = property on="Image Selector" class="Ring (strict)"("Val(Sgnl)"=w561) -> ()  [unwired: 2 in, 2 out]
                }
                event "Display": Value Change {
                  n894 = event-data() -> ("NewVal"=w571:T26)  [unwired: 1 out]
                  n895 = local read "Display Current"() -> (w567:bool)
                  n896 = Unbundle By Name(w571) -> ("Show Centroid"=w573:bool)
                  n897 = Unbundle By Name(w571) -> ("Show Target Area"=w566:bool)
                  n898 = Unbundle By Name(w571) -> ("Show Target"=w580:bool)
                  n899 = And(x=w573, y=w567) -> (x .and. y?=w574:bool)
                  n900 = property on="Displayed Image" class="IntGraph (strict)"("Active Cursor"=u32 1 ("Active Plot"), "Cursor.Visible"=w580, "Active Cursor"=u32 3 ("Active Plot"), "Cursor.Visible"=w574, "Active Cursor"=u32 4 ("Active Plot"), "Cursor.Visible"=w566, "Active Cursor"=u32 5 ("Active Plot"), "Cursor.Visible"=w566) -> ()  [unwired: 2 in, 2 out]
                  n901 = Unbundle By Name(w571) -> ("Show Avg Centroid"=w569:bool)
                  n902 = Unbundle By Name(w571) -> ("Show Best Rect"=w568:bool)
                  n903 = And(x=w568, y=w567) -> (x .and. y?=w572:bool)
                  n904 = property on="Displayed Image" class="IntGraph (strict)"("Active Cursor"=u32 6 ("Active Plot"), "Cursor.Visible"=w572, "Active Cursor"=u32 7 ("Active Plot"), "Cursor.Visible"=w572, "Active Cursor"=u32 2 ("Active Plot"), "Cursor.Visible"=w569) -> ()  [unwired: 2 in, 2 out]
                }
                event "Fancy Display Options.Use fancy display": Value Change {
                  n905 = event-data() -> ("NewVal"=w582:bool, "OldVal"=w583:bool)  [unwired: 1 out]
                  n906 = property on="Displayed Image" class="IntGraph (strict)"("Visible"=w583) -> ()  [unwired: 2 in, 2 out]
                  n907 = property on="Fancy Display" class="Pict"("Visible"=w582) -> ()  [unwired: 2 in, 2 out]
                }
                event "restart": Value Change {
                  # "if stop set to true, stop the main loop"
                  n908 = event-data() -> ("NewVal"=w585:bool)  [unwired: 6 out]
                  n909 = Not(x=w585) -> (.not. x?=w584:bool)
                  n910 = local write "RunON/OFF"(w584) -> ()
                }
                event "Auto": Value Change {
                  n911 = event-data() -> ()  [unwired: 7 out]
                  n912 = stacked-sequence {
                    frame #0 {
                      n913 = local write "RunON/OFF"(FALSE ("RunON/OFF")) -> ()
                    }
                    frame #1 {
                      n914 = Wait (ms)(milliseconds to wait=u32 100) -> ()  [unwired: 1 out]
                    }
                    frame #2 {
                      n915 = local write "RunON/OFF"(TRUE ("RunON/OFF")) -> ()
                    }
                  }
                }
                event "stop": Value Change {
                  n916 = event-data() -> ()  [unwired: 7 out]
                  n917 = local write "restart"(TRUE ("restart")) -> ()
                  n918 = local write "RunON/OFF"(FALSE ("restart")) -> ()
                }
                event "# imgs to avg": Value Change {
                  n919 = event-data() -> ("OldVal"=w592:i32)  [unwired: 6 out]
                  n920 = local write "# imgs to avg"(w592) -> ()
                  n921 = local write "Status"("Stop and restart to change this value." ("status")) -> ()
                }
                event "Correction Parameters.Movement Type": Value Change {
                  n922 = event-data() -> ("NewVal"=w594:u16)  [unwired: 1 out]
                  n923 = case shown="0, Default" w594 {
                    tunnel: ["Steps" "Scalers"] -> w593
                    frame 0, Default {
                    }
                    frame 1 {
                    }
                  }
                  n924 = property on="X" class="DigNum (strict)"("Caption.Text"=w593) -> ()  [unwired: 2 in, 2 out]
                  n925 = property on="Y" class="DigNum (strict)"("Caption.Text"=w593) -> ()  [unwired: 2 in, 2 out]
                }
                event "Select ROI": Value Change {
                  n926 = event-data() -> ()  [unwired: 2 out]
                  n927 = local read "Acq Img"() -> (w607:T1)
                  n928 = local read "error CamS"() -> (w606:errorcluster)
                  n929 = call "IMAQ Select Rectangle"("error in (no error)"=w606, "Image In"=w607) -> ("error out"=w605:errorcluster, "Cancelled"=w597:bool, "Rectangle"=w604:T13)  [unwired: 6 in, 1 out]
                  n930 = local write "error CamS"(w605) -> ()
                  n931 = Unbundle(w604) -> ("Left"=w603:i32, "Top"=w602:i32, "Right"=w601:i32, "Bottom"=w600:i32)  [unwired: 1 out]
                  n932 = Build Array(w603, w602, w601, w600) -> (w599:i32[])
                  n933 = Select(t=i32[] [0, 0, 0, 0] ("Region of Interest"), s=w597, f=w599) -> (s? t:f=w608:i32[])
                  n934 = property on="Region of Interest" class="Arr (strict)"("Val(Sgnl)"=w608) -> ()  [unwired: 2 in, 2 out]
                  n935 = local write "Select ROI"(FALSE ("Select ROI")) -> ()
                }
                event "Reset ROI": Value Change {
                  n936 = event-data() -> ()  [unwired: 2 out]
                  n937 = Initialize Array(0 ("element"), 4 ("dimension size")) -> (w613:i32[])
                  n938 = local write "Region of Interest"(w613) -> ()
                  n939 = local write "Reset ROI"(FALSE ("Reset ROI")) -> ()
                }
                event "Image Selector": Value Change {
                  n940 = event-data() -> ("NewVal"=w619:u16)  [unwired: 1 out]
                  n941 = local read "LoopMode"() -> (w618:bool)
                  n942 = local read "# of cams"() -> (w620:i32)
                  n943 = Not Equal?(x=w619, y=w620) -> (x != y?=w617:bool)
                  n944 = And(x=w617, y=w618) -> (x .and. y?=w616:bool)
                  n945 = Not(x=w616) -> (.not. x?=w615:bool)
                  n946 = local write "Display Current"(w615) -> ()
                  n947 = local read "Display"() -> (w614:T26)
                  n948 = property on="Display" class="Clust (strict)"("Val(Sgnl)"=w614) -> ()  [unwired: 2 in, 2 out]
                }
                event "Auto Detect Param": Value Change {
                  n949 = event-data() -> ("NewVal"=w626:bool)  [unwired: 6 out]
                  n950 = local read "Select ROI"() -> (w624:bool)
                  n951 = Not(x=w624) -> (.not. x?=w622:bool)
                  n952 = Not(x="LoopMode") -> (.not. x?=w623:bool)
                  n953 = Compound Arithmetic op=AND(w626, w623, w622) -> (w625:bool)
                  n954 = case shown="False" w625 {
                    selector: w625 -> [w627 _]
                    frame False {
                      n955 = local write "Auto Detect Param"(w627) -> ()
                      n956 = local write "Status"("Auto Detect Param\n unable in automatic mode\nor when select ROI is on." ("status")) -> ()
                    }
                    frame True {
                      n957 = local write "RunON/OFF"(TRUE ("Substract Background")) -> ()
                    }
                  }
                }
                event "Grab Backround Image": Mouse Up {
                  w641 = FALSE ("Visible")
                  n958 = event-data() -> ()  [unwired: 9 out]
                  n959 = property on="Image to save" class="IntGraph (strict)"("Visible"=TRUE) -> ()  [unwired: 2 in, 2 out]
                  n960 = property on="Grab reference Image" class="Bool (strict)"("Visible"=w641) -> ()  [unwired: 2 in, 2 out]
                  n961 = property on="Grab Backround Image" class="Bool (strict)"("Visible"=w641) -> ()  [unwired: 2 in, 2 out]
                  n962 = property on="Base Directory" class="Path"("Visible"=w641) -> ()  [unwired: 2 in, 2 out]
                  n963 = property on="SavePict" class="Bool (strict)"("Visible"=w641) -> ()  [unwired: 2 in, 2 out]
                  n964 = local read "Acq Img"() -> (w633:T1)
                  n965 = local read "CamConfigArray"() -> (w636:T9)
                  n966 = local read "USB cameras"() -> (w635:i32)
                  n967 = local read "Buffer"() -> (w634:T1)
                  n968 = call "IMAQ ImageToArray"("Image"=w633) -> ("Image Pixels (U8)"=w638:u8[][])  [unwired: 3 in, 4 out]
                  n969 = call "IMAQ Copy"("Image Dst"=w634, "Image Src"=w633) -> ()  [unwired: 4 in, 2 out]
                  n970 = local write "Image to save"(w638) -> ()
                  n971 = call "Display Message Background"() -> ("OK"=w640:bool)  [unwired: 10 in, 1 out]
                  n972 = Index Array(array=w636, index=w635) -> (element=w637:T36)
                  n973 = case shown="False" w640 {
                    tunnel: [TRUE ("Visible") TRUE ("Visible")] -> w639
                    tunnel: w637 -> [_ w646]
                    frame False {
                    }
                    frame True {
                      n974 = local read "Buffer"() -> (w645:T1)
                      n975 = local read "Background Img"() -> (w647:T1)
                      n976 = call "Save Background Img.vi"("Acq Img"=w645, "CamConfigCluster"=w646) -> ("Background Path"=w643:path)  [unwired: 9 in]
                      n977 = call "IMAQ Copy"("Image Dst"=w647, "Image Src"=w645) -> ("Image Dst Out"=w644:T1)  [unwired: 4 in, 1 out]
                      n978 = local write "Background Path"(w643) -> ()
                      n979 = local write "Background Img"(w644) -> ()
                    }
                  }
                  n980 = local write "Grab Backround Image"(FALSE ("Grab Backround Image")) -> ()
                  n981 = Not(x=w639) -> (.not. x?=w630:bool)
                  n982 = property on="Grab reference Image" class="Bool (strict)"("Visible"=w639) -> ()  [unwired: 2 in, 2 out]
                  n983 = property on="Grab Backround Image" class="Bool (strict)"("Visible"=w639) -> ()  [unwired: 2 in, 2 out]
                  n984 = property on="Base Directory" class="Path"("Visible"=w639) -> ()  [unwired: 2 in, 2 out]
                  n985 = property on="SavePict" class="Bool (strict)"("Visible"=w639) -> ()  [unwired: 2 in, 2 out]
                  n986 = property on="Image to save" class="IntGraph (strict)"("Visible"=w630) -> ()  [unwired: 2 in, 2 out]
                }
                event "Grab reference Image": Mouse Up {
                  w661 = FALSE ("Visible")
                  n987 = event-data() -> ()  [unwired: 9 out]
                  n988 = property on="Image to save" class="IntGraph (strict)"("Visible"=TRUE) -> ()  [unwired: 2 in, 2 out]
                  n989 = property on="Grab reference Image" class="Bool (strict)"("Visible"=w661) -> ()  [unwired: 2 in, 2 out]
                  n990 = property on="Grab Backround Image" class="Bool (strict)"("Visible"=w661) -> ()  [unwired: 2 in, 2 out]
                  n991 = property on="Base Directory" class="Path"("Visible"=w661) -> ()  [unwired: 2 in, 2 out]
                  n992 = property on="SavePict" class="Bool (strict)"("Visible"=w661) -> ()  [unwired: 2 in, 2 out]
                  n993 = local read "CamConfigArray"() -> (w655:T9)
                  n994 = local read "Acq Img"() -> (w654:T1)
                  n995 = local read "USB cameras"() -> (w656:i32)
                  n996 = local read "Buffer"() -> (w653:T1)
                  n997 = call "IMAQ ImageToArray"("Image"=w654) -> ("Image Pixels (U8)"=w658:u8[][])  [unwired: 3 in, 4 out]
                  n998 = local write "Image to save"(w658) -> ()
                  n999 = call "IMAQ Copy"("Image Dst"=w653, "Image Src"=w654) -> ("Image Dst Out"=w649:T1)  [unwired: 4 in, 1 out]
                  n1000 = local write "Buffer"(w649) -> ()
                  n1001 = Index Array(array=w655, index=w656) -> (element=w657:T36)
                  n1002 = call "Display Message Reference"() -> ("OK"=w660:bool)  [unwired: 10 in, 1 out]
                  n1003 = case shown="False" w660 {
                    tunnel: [TRUE ("Visible") TRUE ("Visible")] -> w659
                    tunnel: w657 -> [_ w664]
                    frame False {
                    }
                    frame True {
                      n1004 = local read "Buffer"() -> (w665:T1)
                      n1005 = local read "Reference Img"() -> (w667:T1)
                      n1006 = call "Save Reference Img.vi"("Acq Img"=w665, "CamConfigCluster"=w664) -> ("Reference Path"=w666:path)  [unwired: 9 in]
                      n1007 = local write "Reference Path"(w666) -> ()
                      n1008 = call "IMAQ Copy"("Image Dst"=w667, "Image Src"=w665) -> ("Image Dst Out"=w663:T1)  [unwired: 4 in, 1 out]
                      n1009 = local write "Reference Img"(w663) -> ()
                    }
                  }
                  n1010 = local write "Grab reference Image"(FALSE ("Grab reference Image")) -> ()
                  n1011 = Not(x=w659) -> (.not. x?=w650:bool)
                  n1012 = property on="Grab reference Image" class="Bool (strict)"("Visible"=w659) -> ()  [unwired: 2 in, 2 out]
                  n1013 = property on="Grab Backround Image" class="Bool (strict)"("Visible"=w659) -> ()  [unwired: 2 in, 2 out]
                  n1014 = property on="Base Directory" class="Path"("Visible"=w659) -> ()  [unwired: 2 in, 2 out]
                  n1015 = property on="SavePict" class="Bool (strict)"("Visible"=w659) -> ()  [unwired: 2 in, 2 out]
                  n1016 = property on="Image to save" class="IntGraph (strict)"("Visible"=w650) -> ()  [unwired: 2 in, 2 out]
                }
                event "Set Color Map": Value Change {
                  n1017 = event-data() -> ("NewVal"=w669:bool)  [unwired: 1 out]
                  n1018 = case shown="True" w669 {
                    frame False {
                    }
                    frame True {
                      n1019 = call "Color Table Generator.vi"() -> ("Color Map"=w670:u32[])
                      n1020 = property on="Displayed Image" class="IntGraph (strict)"("Color Table"=w670) -> ()  [unwired: 2 in, 2 out]
                    }
                  }
                }
                event "Open CamCenter": Value Change {
                  n1021 = event-data() -> ("NewVal"=w671:bool)  [unwired: 1 out]
                  n1022 = case shown="True" w671 {
                    frame False {
                    }
                    frame True {
                      # "open creative live! cam center"
                      n1023 = call <vilib>:"System Exec.vi"("wait until completion? (T)"=FALSE, "command line"="open \"C:\\BeamPointing\\trunk\\Beam Poin\nting v22 Library\\xml Settings\\ConfigFile.xml\"") -> ("error out"=w672:errorcluster)  [unwired: 4 in, 5 out]
                      n1024 = call <vilib>:"Simple Error Handler.vi"("error in (no error)"=w672) -> ()  [unwired: 4 in, 5 out]
                    }
                  }
                }
              }
            }
            n1025 = disable-structure shown="Disabled" {
              disable-tunnel: w402 -> [w406 _]
              frame Disabled {
                n1026 = for {
                  tunnel: "image::" ("image prefix") -> [w413]
                  tunnel: w406 -> [_] mode=indexing
                  tunnel: [w414] -> _ mode=indexing
                  tunnel: [w412] -> w408 mode=indexing
                  i -> [w411]
                  n1027 = Increment(x=w411) -> (x+1=w410:i32)
                  n1028 = Number To Decimal String(number=w410) -> (decimal integer string=w409:string)  [unwired: 1 in]
                  n1029 = Concatenate Strings(w413, w409) -> (w412:string)
                  n1030 = Type Cast(type=T1 refnum ("New Image"), x=w412) -> (*(type *) &x=w414:T1)
                }
                "image names" <- w408
              }
              frame Enabled {
              }
            }
            n1031 = Array Size(array=w402) -> (size(s)=w400:i32)
            n1032 = Array Subset(array=w401, length=w400) -> (w399:T1[])  [unwired: 1 in]
            n1033 = while {
              tunnel: w399 -> [w417]
              stop <- w416 stop-if-true
              n1034 = local read "Detection status"() -> (w421:string[])
              n1035 = local read "USB cameras"() -> (w423:i32)
              n1036 = local read "Raw images"() -> (w437:T1[])
              n1037 = local read "CamConfigArray"() -> (w426:T9)
              n1038 = call "Select Target Circle Colors.vi"("USB cameras"=w423) -> ("Array"=w425:u32[])  [unwired: 1 in]
              n1039 = local read "Ann. Images"() -> (w419:T1[])
              n1040 = Array Size(array=w437) -> (size(s)=w436:i32)
              n1041 = for {
                workers-P: w436 -> [_]
                tunnel: w437 -> [w468] mode=indexing
                tunnel: [w467] -> w418 mode=indexing
                tunnel: w426 -> [w466] mode=indexing
                tunnel: w425 -> [w464] mode=indexing
                tunnel: "CamOn" -> [w463] mode=indexing
                tunnel: w421 -> [w462] mode=indexing
                tunnel: "UDP timeout ms" -> [w461]
                tunnel: w419 -> [w460] mode=indexing
                tunnel: w417 -> [w459] mode=indexing
                i -> [w465]
                n1042 = case shown="True" w463 {
                  tunnel: w468 -> [_ w478]
                  tunnel: [w469 w475] -> w467
                  tunnel: w466 -> [_ w477]
                  tunnel: w464 -> [_ w474]
                  tunnel: w462 -> [_ w473]
                  tunnel: w461 -> [_ _]
                  tunnel: w460 -> [w469 w472]
                  tunnel: w459 -> [_ w470]
                  frame False {
                  }
                  frame True {
                    n1043 = call "IMAQ Copy"("Image Dst"=w478, "Image Src"=w470) -> ("Image Dst Out"=w476:T1)  [unwired: 4 in, 1 out]
                    n1044 = call "annotate image.vi"("Detection string"=w473, "Color"=w474, "CamConfigArray"=w477, "rescale"="rescale", "Image Dst"=w472, "Image in"=w476) -> ("Image Dst Out"=w475:T1)  [unwired: 4 in, 1 out]
                  }
                }
                "grab loop i" <- w465
              }
              n1045 = local write "Ann. Images"(w418) -> ()
              n1046 = Index Array(array=w418) -> (element #1=→"Image":T1, element #2=→"Image 2":T1, element #3=→"Image 3":T1, element #4=→"Image 4":T1, element #5=→"Image 5":T1, element #6=→"Image 6":T1, element #7=→"Image 7":T1, element #8=→"Image 8":T1, element #9=→"Image 9":T1)  [unwired: 9 in]
              n1047 = Wait (ms)(milliseconds to wait=u32 100) -> ()  [unwired: 1 out]
              n1048 = case shown="False" "recenter" {
                frame False {
                }
                frame True {
                  n1049 = control-ref of="Image"() -> (w441:refnum<vi>)
                  n1050 = control-ref of="Image 2"() -> (w443:refnum<vi>)
                  n1051 = control-ref of="Image 3"() -> (w444:refnum<vi>)
                  n1052 = control-ref of="Image 4"() -> (w445:refnum<vi>)
                  n1053 = control-ref of="Image 5"() -> (w446:refnum<vi>)
                  n1054 = control-ref of="Image 6"() -> (w447:refnum<vi>)
                  n1055 = control-ref of="Image 7"() -> (w448:refnum<vi>)
                  n1056 = control-ref of="Image 8"() -> (w449:refnum<vi>)
                  n1057 = control-ref of="Image 9"() -> (w450:refnum<vi>)
                  n1058 = local read "CamConfigArray"() -> (w439:T9)
                  n1059 = local write "recenter"(FALSE ("recenter")) -> ()
                  n1060 = Build Array(w441, w443, w444, w445, w446, w447, w448, w449, w450) -> (w442:refnum<vi>[])
                  n1061 = for {
                    tunnel: w442 -> [w458] mode=indexing
                    tunnel: w439 -> [w457] mode=indexing
                    n1062 = Unbundle By Name(w457) -> ("CorrectConfig Cluster.Target"=w456:cluster{"X Target":sgl, "Y Target":sgl}, "CorrectConfig Cluster.Detection Parameters.Rx"=w453:i32)
                    n1063 = Reciprocal(x=w453) -> (1/x=w452:dbl)
                    n1064 = Divide(x=w452, y=0.01 ("1/x")) -> (x/y=w454:dbl)
                    n1065 = Bundle(w454, w454) -> (w455:cluster{dbl, dbl})  [unwired: 1 in]
                    n1066 = property class="ImageControl"(reference=w458, "ZoomSingle"=w455, "Image Center Position"=w456) -> ()  [unwired: 1 in, 2 out]
                  }
                }
              }
              n1067 = local read "restart"() -> (w416:bool)
            }
            n1068 = while {
              stop <- w677 stop-if-true
              # "TCP reception from picodrivers server"
              n1069 = local read "ConnectArray"() -> (w678:T7)
              n1070 = local read "restart"() -> (w677:bool)
              n1071 = for {
                tunnel: w678 -> [w687] mode=indexing
                i -> [w680]
                n1072 = Unbundle(w687) -> ("connection ID"=w686:refnum<k5>, "TCP error"=w683:errorcluster)  [unwired: 2 out]
                n1073 = Wait (ms)(milliseconds to wait=u32 200) -> ()  [unwired: 1 out]
                n1074 = call "TCPread8bytes.vi"("Error in"=w683, "timeout ms (25000)"=500, "connection ID in"=w686) -> ("Error out"=w681:errorcluster, "string out"=w684:string, "connection ID out"=w679:refnum<k5>)  [unwired: 6 out]
                n1075 = case shown="\"close\"" w684 {
                  selector: w684 -> [w688 _ w698]
                  tunnel: w681 -> [w691 _ w702]
                  tunnel: w680 -> [w693 _ _]
                  tunnel: w679 -> [_ _ w703]
                  frame Default {
                    n1076 = local write "Status"(w688) -> ()
                    n1077 = local read "InProgress"() -> (w690:string[])
                    n1078 = Decrement(x=w693) -> (x-1=w692:i32)
                    n1079 = Unbundle By Name(w691) -> ("status"=w696:bool)
                    n1080 = local read "ConnectArray"() -> (w694:T7)
                    n1081 = Not(x=w696) -> (.not. x?=w697:bool)
                    n1082 = call "EndOfMove-2.vi"("InProgressIN"=w690, "String in"=w688) -> ("InProgressOUT"=w689:string[])  [unwired: 8 out]
                    n1083 = local write "TCPconnecAnswer"(w697) -> ()
                    n1084 = local write "InProgress"(w689) -> ()
                    n1085 = call "LoadConnectionIDerror.vi"("ArrayIN"=w694, "ErrorIn"=w691, "index"=w692) -> ("ArrayOUT"=w695:T7)  [unwired: 8 out]
                    n1086 = local write "ConnectArray"(w695) -> ()
                  }
                  frame "" {
                  }
                  frame "close" {
                    n1087 = local write "Status"(w698) -> ()
                    n1088 = TCP Close Connection(connection ID=w703, error in (no error)=w702) -> (connection ID out=w701:refnum<k5>)  [unwired: 2 out]
                    n1089 = local read "ConnectArray"() -> (w700:T7)
                    n1090 = call "RemoveConnectionID.vi"("ArrayIN"=w700, "connection ID"=w701) -> ("ArrayOUT"=w699:T7)  [unwired: 9 out]
                    n1091 = local write "ConnectArray"(w699) -> ()
                  }
                }
              }
              n1092 = local read "InProgress"() -> (w676:string[])
              n1093 = call "EndOfMove-2.vi"("InProgressIN"=w676) -> ("InProgress"=w675:bool)  [unwired: 1 in, 8 out]
              n1094 = property on="MoveInProgress" class="Bool (strict)"("Val(Sgnl)"=w675) -> ()  [unwired: 2 in, 2 out]
            }
          }
          frame #2 {
            n1095 = local read "ConnectArray"() -> (w1718:T7)
            n1096 = local write "restart"(FALSE ("stop")) -> ()
            n1097 = for {
              tunnel: w1718 -> [w1769] mode=indexing
              # "close all connection"
              n1098 = Unbundle(w1769) -> ("connection ID"=w1767:refnum<k5>, "TCP error"=w1766:errorcluster)  [unwired: 2 out]
              n1099 = call "TCPwrite8bytes.vi"("Error in"=w1766, "Cmd In"="webcam:close", "connection ID in"=w1767) -> ("Error out"=w1765:errorcluster, "connection ID out"=w1764:refnum<k5>)  [unwired: 7 in]
              n1100 = TCP Close Connection(connection ID=w1764, error in (no error)=w1765) -> (error out=w1768:errorcluster)  [unwired: 2 out]
              n1101 = local write "error close connect"(w1768) -> ()
            }
            n1102 = stacked-sequence {
              frame #0 {
                n1103 = local read "AddCameraCluster"() -> (w1722:T8)
                n1104 = Unbundle By Name(w1722) -> ("Add?"=w1721:bool, "Channel"=w1719:i32, "Device Name"=w1720:string)
                n1105 = case shown="True" w1721 {
                  tunnel: w1720 -> [_ w1723]
                  tunnel: w1719 -> [_ _]
                  frame False {
                  }
                  frame True {
                    w1724 = T36 {"ID"=0.0, "Name"="no-device", "DeviceID"={"Slot Connector"=0, "IP Adress"="Ipaddress", "Port"=0, "Type"="Type"}, "CorrectConfig Cluster"={"Detection Parameters"={"Contrast"=0, "Treshold"=0, "Max Intensity"=0, "Max Intensity%"=0, "Rx"=0, "Ry"=0, "R%"=0.0}, "Reverse"={"Reverse X"=FALSE, "Reverse Y"=FALSE}, "Target"={"X Target"=0.0, "Y Target"=0.0}, "Region of Interest"=[0, 0, 0, 0], "Correction Parameters"={"X"=0.0, "Y"=0.0, "Movement Type"=0}, "Acquisition Parameters"={"Brightness"=0.0, "Contrast"=0.0, "Saturation"=0.0, "White level"=0.0}, "Background Path"=path "", "Reference Path"=path "", "XCalibration"=[], "YCalibration"=[]}, "Ontrak Channel"=0, "IMAQdx Session 2"="cam2", "ImageServer"={"IPAddress"="", "Port"=0}}
                    n1106 = local read "AddCameraCluster"() -> (w1726:T8)
                    n1107 = Bundle By Name(cluster=w1726, "Add?"=FALSE) -> (w1727:T8)
                    n1108 = local write "AddCameraCluster"(w1727) -> ()
                    n1109 = local read "CamConfigArray"() -> (w1729:T9)
                    n1110 = Bundle By Name(cluster=w1724, "Name"=w1723) -> ()  [unwired: 1 out]
                    n1111 = Build Array (concatenate)(w1729, w1724) -> (w1728:T9)
                    n1112 = local write "CamConfigArray"(w1728) -> ()
                  }
                }
              }
              frame #1 {
                n1113 = local read "XML errors"() -> (w1730:bool)
                n1114 = case shown="False" w1730 {
                  frame False {
                    n1115 = stacked-sequence {
                      frame #0 {
                        n1116 = local read "Mirror List Path"() -> (w1739:path)
                        n1117 = call "LoadDeviceList.vi"("usb/RS170"=FALSE, "path to XML document"=w1739) -> ("DeviceList"=w1740:T16)  [unwired: 7 in, 2 out]
                        n1118 = local read "CamConfigArray"() -> (w1732:T9)
                        n1119 = call "parse device list by type.vi"("DeviceListin"=w1740) -> ("DeviceListout"=w1738:T16)  [unwired: 1 in]
                        n1120 = local read "Mirrors"() -> (w1737:u8[])
                        n1121 = call "associate mirrors and cameras.vi"("Mirrors"=w1737, "DeviceList"=w1738) -> ("CamConfigArray"=w1734:T9)  [unwired: 1 in]
                        n1122 = Not Equal?(x=w1734, y=w1732) -> (x != y?=w1736:bool)
                        "configarraychanged" <- w1736
                        n1123 = case shown="True" w1736 {
                          tunnel: [TRUE ("T button?") w1743] -> w1735
                          frame False {
                          }
                          frame True {
                            n1124 = Two Button Dialog(message="READ! config has changed.\nplease ensure all other BP\ninstances SHARING same\n cameras are shutdown\nbefore saving config.", 1:"Dont save config" ("F button name (\"Cancel\")"), 2:"save" ("T button name (\"OK\")")) -> (T button?=w1743:bool)
                          }
                        }
                        "really save cfg?" <- w1735
                        n1125 = Select(t=w1732, s=w1735, f=w1734) -> (s? t:f=w1733:T9)
                        n1126 = local write "CamConfigArray"(w1733) -> ()
                      }
                      frame #1 {
                        n1127 = local read "really save cfg?"() -> (w1746:bool)
                        n1128 = case shown="True" w1746 {
                          frame False {
                          }
                          frame True {
                            n1129 = local read "CamConfigArray"() -> (w1753:T9)
                            n1130 = local read "Cameras Names"() -> (w1748:string[])
                            n1131 = Array Size(array=w1753) -> (size(s)=w1751:i32)
                            n1132 = Array Size(array=w1748) -> (size(s)=w1750:i32)
                            n1133 = Subtract(x=w1751, y=w1750) -> (x-y=w1752:i32)
                            n1134 = for {
                              N: w1752 -> [_]
                              shift-right: [w1758] -> w1749
                              shift-left: w1748 -> [w1759]
                              n1135 = Build Array (concatenate)(w1759, "Null") -> (w1758:string[])
                            }
                            n1136 = local read "Mirror List Path"() -> (w1757:path)
                            n1137 = local read "XML Config File Path"() -> (w1756:path)
                            n1138 = call "SaveCamConfig-v5.vi"("file path in"=w1757, "CamConfigArray"=w1753) -> ("parse errors"=w1754:string)  [unwired: 7 in]
                            n1139 = call "SaveConfig.vi"("path to XML document"=w1756, "USB/RS170 cams"=FALSE, "CamerasNames"=w1749, "DeviceConfigArray"=w1753) -> ("error out"=w1755:errorcluster)  [unwired: 7 in]
                            n1140 = local write "Status"(w1754) -> ()
                            n1141 = call <vilib>:"Simple Error Handler.vi"("error in (no error)"=w1755) -> ()  [unwired: 4 in, 5 out]
                          }
                        }
                      }
                    }
                  }
                  frame True {
                  }
                }
              }
              frame #2 {
                n1142 = disable-structure shown="Enabled" {
                  frame Disabled {
                    n1143 = local read "Mirror List Path"() -> (w1762:path)
                    n1144 = local read "XML Config File Path"() -> (w1761:path)
                    n1145 = call "StripEmtyLines.vi"("Path"=w1762) -> ()
                    n1146 = call "StripEmtyLines.vi"("Path"=w1761) -> ()
                  }
                  frame Enabled {
                  }
                }
              }
            }
            n1147 = local read "error CamS"() -> (w1711:errorcluster)
            n1148 = local read "Acq Img"() -> (w1716:T1)
            n1149 = local read "Background Img"() -> (w1707:T1)
            n1150 = local read "Thresh Img"() -> (w1717:T1)
            n1151 = local read "Thresh Img"() -> (w1706:T1)
            n1152 = local read "Thresh Img"() -> (w1704:T1)
            n1153 = local read "Avg Img"() -> (w1715:T1)
            n1154 = call "IMAQ Dispose"("Image"=w1716, "error in (no error)"=w1711) -> ("error out"=w1713:errorcluster)  [unwired: 1 in, 3 out]
            n1155 = call "IMAQ Dispose"("Image"=w1715, "error in (no error)"=w1713) -> ("error out"=w1712:errorcluster)  [unwired: 1 in, 3 out]
            n1156 = call "IMAQ Dispose"("Image"=w1717, "error in (no error)"=w1712) -> ("error out"=w1705:errorcluster)  [unwired: 1 in, 3 out]
            n1157 = call "IMAQ Dispose"("Image"=w1707, "error in (no error)"=w1705) -> ("error out"=w1708:errorcluster)  [unwired: 1 in, 3 out]
            n1158 = call "IMAQ Dispose"("Image"=w1706, "error in (no error)"=w1708) -> ("error out"=w1703:errorcluster)  [unwired: 1 in, 3 out]
            n1159 = call "IMAQ Dispose"("Image"=w1704, "error in (no error)"=w1703) -> ("error out"=w1702:errorcluster)  [unwired: 1 in, 3 out]
            n1160 = call <vilib>:"Clear Errors.vi"("error in (no error)"=w1702) -> ("error out"=w1710:errorcluster)  [unwired: 6 in]
            n1161 = local write "error CamS"(w1710) -> ()
            n1162 = local read "stop"() -> (w1709:bool)
          }
        }
      }
    }
    frame #2 {
      n1163 = local read "Raw images"() -> (w1772:T1[])
      n1164 = local read "XML Config File Path"() -> (w1771:path)
      n1165 = local read "Mirror List Path"() -> (w1770:path)
      n1166 = for {
        tunnel: w1772 -> [w1774] mode=indexing
        n1167 = call "IMAQ Dispose"("Image"=w1774) -> ()  [unwired: 2 in, 4 out]
      }
      n1168 = local write "stop"(FALSE ("Stop")) -> ()
      n1169 = call "StripEmtyLines.vi"("Path"=w1770) -> ()
      n1170 = call "StripEmtyLines.vi"("Path"=w1771) -> ()
    }
  }
  n1171 = for {
    N: 8 -> [_]
    tunnel: "sdfsesdfsdf" ("string") -> [w1778]
    tunnel: [w1777] -> w4 mode=indexing
    tunnel: w11 -> [w1775]
    i -> [w1780]
    n1172 = Increment(x=w1780) -> (x+1=w1776:i32)
    n1173 = Number To Decimal String(number=w1776) -> (decimal integer string=w1779:string)  [unwired: 1 in]
    n1174 = Concatenate Strings(w1778, w1779) -> (w1781:string)
    n1175 = call "IMAQ Create"("Image Name"=w1781, "Image Type"=w1775) -> ("New Image"=w1777:T1)  [unwired: 3 in, 1 out]
  }
  n1176 = Index Array(array=w4) -> (element #1=→"image::1":T1, element #2=→"image::2":T1, element #3=→"image::3":T1, element #4=→"image::4":T1, element #5=→"image::5":T1, element #6=→"image::6":T1, element #7=→"image::7":T1, element #8=→"image::8":T1, element #9=→"image::9":T1)  [unwired: 9 in]
  n1177 = stacked-sequence {
    frame #0 {
      n1178 = while {
        tunnel: [w1801] -> w1790
        tunnel: [w1799] -> w1789
        tunnel: [w1798] -> w1788
        tunnel: [w1797] -> w1787
        tunnel: [w1796] -> w1786
        tunnel: [w1795] -> w1785
        tunnel: [w1794] -> w1784
        tunnel: [w1793] -> w1783
        tunnel: [w1792] -> _
        tunnel: [w1791] -> w1782
        stop <- w1802 stop-if-true
        n1179 = local read "MirrorsNames"() -> (w1805:string[])
        n1180 = Empty Array?(array=w1805) -> (empty?=w1804:bool)
        n1181 = Not(x=w1804) -> (.not. x?=w1803:bool)
        n1182 = local read "stop"() -> (w1800:bool)
        n1183 = Or(x=w1803, y=w1800) -> (x .or. y?=w1802:bool)
        n1184 = Index Array(array=w1805) -> (element #1=w1801:string, element #2=w1799:string, element #3=w1798:string, element #4=w1797:string, element #5=w1796:string, element #6=w1795:string, element #7=w1794:string, element #8=w1793:string, element #9=w1792:string, element #10=w1791:string)  [unwired: 12 in, 2 out]
      }
      "GUIdevice 1" <- w1790
      "GUIdevice 2" <- w1789
      "GUIdevice 3" <- w1788
      "GUIdevice 4" <- w1787
      "GUIdevice 5" <- w1786
      "GUIdevice 6" <- w1785
      "GUIdevice 7" <- w1784
      "GUIdevice 8" <- w1783
      "GUIdevice 9" <- w1782
    }
    frame #1 {
      n1185 = call "supergui create stop queue.vi"() -> ("STOP Queue out"=w1806:refnum<queue>)  [unwired: 11 in]
      n1186 = Create User Event(user event datatype=T46 {"EventEnum"=enum."new data", "Device name"="Device name"} ("New Event")) -> (user event=w1808:refnum<user-event>, error out=w1809:errorcluster)  [unwired: 1 in]
      "tcp data event" <- w1808
      n1187 = control-ref of="This VI"() -> (w1812:refnum<vi>)
      n1188 = control-ref of="This Application"() -> (w1807:refnum<vi>)
      n1189 = Current VI's Menubar() -> (w1811:refnum<k9>)
      n1190 = call "GUI_Master_subvi_reentrant_queues.vi"("STOP Queue in"=w1806, "This Application"=w1807, "error in (no error)"=w1809, "tcp data event"=w1808, "Caller menu reference"=w1811, "Caller VI ref"=w1812) -> ("error out"=→"error IO 2":errorcluster)  [unwired: 5 in]
    }
    frame #2 {
      n1191 = disable-structure shown="Enabled" {
        frame Enabled {
          n1192 = local write "MirrorsNames"(string[] [] ("MirrorsNames")) -> ()
        }
        frame Disabled {
        }
      }
    }
  }
  n1193 = local write "Main tab"(T18."User Main View" ("Main tab")) -> ()
